vi "Diagnostics.Main.CmdResp.Engine.vi"(8 "error in (no error)":errorcluster, 11 "State Variables":T1={"Comm"=refnum, "Parameters"={"Name"="", "CAN"={"Interface"="", "Baud Rate"=0, "Diagnostic Protocol"=enum."GMLAN", "Transport Protocol"=enum."ISO TP - Normal Mode", "Transmit ID"=0, "Receive ID"=2, "Transmit Extension"=1, "Receive Extension"=255, "Receive UUDT ID"=0, "Enable Stream"=TRUE, "VW TP Channel ID"=1, "Fill Frame"=FALSE, "Fill Byte"=0, "Termination"=FALSE, "LIN Cluster"="", "NAD"=8, "IO Mode"=0, "Max DLC"=0, "FD Baud Rate"=2, "Timeout"=1, "FD ISO Mode"=0}, "986x"={"Enable"=FALSE, "RIO Device"="", "Bitfile"=path ""}, "Reads"=[], "Frames Lookup"=variant(enum16{"GMLAN", "KWP-2000", "UDS"} enum."GMLAN"), "Writes"=[], "DPIDs"=[], "DPID Lookup"=variant(u32 0), "DTC"={"Descriptor"={"DTC Byte Length"=1, "Status Byte Length"=1, "Add Data Byte Length"=1, "Byte Order"=enum."Motorola"}, "Value.Code"=[], "Value.String"=[], "Value.J2012String"=[], "Status.Code"=[], "Status.String"=[]}, "Created DTCs"=0, "Polls"=[], "Service Channels Status Lookup"=variant, "Trigger Lookup"=variant, "Security"={"Type"=enum."None", "Source DLL Path"=path "", "Target DLL Path"=path "", "Security Level"=0}}, "ADCS Connection"={"Diag CAN Handle"=0, "Transport Protocol"=enum."ISO TP - Normal Mode", "Receive Address Extension"=0, "Transmit Address Extension"=0, "Receive CAN Id"=0, "Transmit CAN Id"=0, "Log Frames ?"=FALSE, "My TP Address"=0, "Other TP Address"=0, "T1"=0, "T2"=0, "T3"=0, "T4"=0, "Tx SN"=0, "Block Size"=0, "Rx SN"=0, "VW TP Initialized?"=FALSE, "Tx block no"=0, "baud rate"=0, "Interface"="", "Channel Diag CAN Handle"=0, "UDP Connection ID"=refnum, "TCP Connection ID"=refnum, "Target IP Addr"=0, "Source Address"=0, "Target Address"=0, "Send Header NACK?"=FALSE, "DLL Handle"=0, "NAD"=0, "Time Stamp read first"=0.0, "Time Stamp read last"=0.0, "Time Stamp write first"=0.0, "Time Stamp write last"=0.0, "Time Stamp write"=0.0, "Time Stamp read"=0.0, " I/O Mode"=0, "FD Baudrate"=0, "TX_DL"=8, "RX_DL"=8, "DoIP Protocol Version"=1, " Selected I/O Mode"=0, "TesterPresent Counter"=0, "TesterPresent Limit"=0, "TesterPresent Tick[ms]"=10, "TesterPresent RequireResponse?"=FALSE, "TesterPresent Stored Ref?"=FALSE, "TesterPresent Message"=[], "TesterPresent Task Handle"=0, "TesterPresent Semaphore"=refnum, "Response Plausibility Check"=1, "Default Version?"=TRUE, "Diagostic Globals"={"Timeout FC (Bs)"=250, "Timeout CF (Cr)"=250, "Timeout Diag Command"=1000, "Receive Block Size (BS)"=0, "Wait Time CF (STmin)"=5, "Max Waits (N_WFTmax)"=10, "Waits to Send (N_WAIT)"=0, "Time between Waits (TW)"=25, "Fill CAN Frames?"=TRUE, "Fill Byte"=255, "Invalid Response as Error?"=FALSE, "Max RspPending Count"=5, "VWTP Command Timeout"=50, "Transport Protocol"=enum."Diagnostics on IP", "Diag CAN Handle"=0, "DLL Handle"=0, "Timeout RspPending"=1000}, "Session-based Properties?"=FALSE}, "XNET References"={"Database"="", "GMLAN.DPID.Frame"="", "Cluster.Convert"=""}, "XNETEngine (GMLAN)"=refnum, "Process"=refnum, "Reads"=refnum, "Writes"=refnum, "Cmds"=refnum, "DTCs"=refnum, "DTC Count"=refnum, "Status"=refnum, "Triggers"=refnum, "CANConnected"=refnum, "LocalStop"=refnum, "LocalCommStatus"=refnum, "Service Channels Status"=refnum, "Settings"=refnum, "Streaming Refs"={"Addon"="", "Port"="", "Filter Ref"=refnum, "Default Filter"={"ID Filters"=[], "Direction Filter"=enum."Tx/Rx", "Type Filter"=enum."All"}, "Port Settings"={"Mode"=0, "Baud Rate"=0, "Termination"=0, "FD ISO Mode"=0, "FD Baud Rate"=0}}} {"Streaming Refs"."Port Settings"."FD ISO Mode" items=["ISO", "Non ISO", "ISO Legacy"]; "Streaming Refs"."Port Settings"."Termination" items=["Off", "On"]; "Streaming Refs"."Port Settings"."Mode" items=["CAN 2.0", "CAN FD", "CAN FD+BRS"]; "ADCS Connection"."Diagostic Globals"."Fill Byte" format="%x"; "ADCS Connection"."TesterPresent Message" format="%.0x"; "ADCS Connection"."Selected I/O Mode" items=["CAN", "CAN FD", "CAN FD+BRS", "ECU Determined"]; "ADCS Connection"."DoIP Protocol Version" items=["2010"=1, "2012"=2]; "ADCS Connection"."RX_DL" items=["8"=8, "12"=12, "16"=16, "20"=20, "24"=24, "32"=32, "48"=48, "64"=64]; "ADCS Connection"."TX_DL" items=["8"=8, "12"=12, "16"=16, "20"=20, "24"=24, "32"=32, "48"=48, "64"=64]; "ADCS Connection"."I/O Mode" items=["CAN", "CAN FD", "CAN FD+BRS", "Not yet determined"]; "Parameters"."Writes"."Signals"."Byte Order" items=["Little Endian", "Big Endian"]; "Parameters"."Writes"."Signals"."Data Type" items=["Signed", "Unsigned", "IEEE Float"]; "Parameters"."CAN"."FD ISO Mode" items=["ISO", "Non ISO", "ISO Legacy"]; "Parameters"."CAN"."IO Mode" items=["CAN 2.0", "CAN FD", "CAN FD+BRS"]; "Parameters"."CAN"."Fill Byte" format="%.0x"; "Parameters"."CAN"."VW TP Channel ID" format="%.0x"; "Parameters"."CAN"."Receive UUDT ID" format="%.0x"; "Parameters"."CAN"."Receive Extension" format="%.0x"; "Parameters"."CAN"."Transmit Extension" format="%.0x"; "Parameters"."CAN"."Receive ID" format="%.0x"; "Parameters"."CAN"."Transmit ID" format="%.0x"; "Parameters"."Reads"."Signals"."Byte Order" items=["Little Endian", "Big Endian"]; "Parameters"."Reads"."Signals"."Data Type" items=["Signed", "Unsigned", "IEEE Float"]}) -> (0 "error out":errorcluster)   [LabVIEW 2019, in "Diagnostics Addon Engine.lvlib"]
doc: "Async loop that handles the UDS commands sent either by the channel engine or the TCP engine"
uses:
  Diagnostics Addon Engine.lvlib
  Types/Diagnostics.State.ctl
  <vilib>/NI/NIVS Inline Async API/_VS Inline Async API/Process/Process.lvclass
  <vilib>/NI/NI VeriStand Addon Network Comm/Engine/VeriStand Comm.lvclass
  Addon Shared/Types/SysDef.Compile.ctl
  Addon Shared/Types/CAN.ctl
  Addon Shared/Types/CAN.Interface.ctl
  Addon Shared/Types/Protocol.ctl
  Addon Shared/Types/Transport.ctl
  Addon Shared/Types/986x.ctl
  Addon Shared/Types/Frame.Compile.ctl
  Addon Shared/Types/Type.ctl
  Addon Shared/Types/Signal.ctl
  Addon Shared/Types/DPID.ctl
  Addon Shared/Types/DPID.Rate.ctl
  Addon Shared/Types/DTC.Settings.ctl
  Addon Shared/Types/DTC.Descriptor.ctl
  Addon Shared/Types/Poll.Compiled.ctl
  Addon Shared/Types/Security.ctl
  Addon Shared/Types/Security.Type.ctl
  <vilib>/Automotive Diagnostic Command Set/Diagnostic Transport.llb/Diag Reference.ctl
  <vilib>/Automotive Diagnostic Command Set/Diagnostic Transport.llb/Transport Protocol Selector.ctl
  <vilib>/Automotive Diagnostic Command Set/Diagnostic Transport.llb/DoIP Protocol Version.ctl
  <vilib>/Automotive Diagnostic Command Set/Diagnostic Transport.llb/Diag Globals.ctl
  Types/XNET.Refs.ctl
  <vilib>/NI/AMC/Message Queue.ctl
  <vilib>/NI/AMC/Message.ctl
  <vilib>/NI/Tools/Keyed Array/KeyedArray.ctl
  <vilib>/NI/NIVS Inline Async API/_Data Access Engine/Data Access Engine/Types/Write.DVR.ctl
  <vilib>/NI/NIVS Inline Async API/_Data Access Engine/Access Type Classes/Write/Write.lvclass
  <vilib>/NI/NIVS Inline Async API/_Data Access Engine/Data Access Engine/Types/Read.DVR.ctl
  <vilib>/NI/NIVS Inline Async API/_Data Access Engine/Access Type Classes/Read/Read.lvclass
  <vilib>/NI/NIVS Inline Async API/_Data Access Engine/Data Access Engine/Types/ReadWrite.DVR.ctl
  <vilib>/NI/NIVS Inline Async API/_Data Access Engine/Access Type Classes/ReadWrite/ReadWrite.lvclass
  SubModules/CAN-Streaming-Support/Source/Addon/Addon Engine/Types/Engine Stream Refs.ctl
  SubModules/CAN-Streaming-Support/Source/Addon/Addon Shared/Types/Direction Filter.ctl
  SubModules/CAN-Streaming-Support/Source/Addon/Addon Shared/Types/Type Filter.ctl
  SubModules/CAN-Streaming-Support/Source/Addon/Addon Shared/Types/Filter Parameters.ctl
  SubModules/CAN-Streaming-Support/Source/Addon/Addon Engine/Types/Engine Stream Port Settings.ctl
  Types/Polling.States.ctl
  Addon Shared/Types/DTC.Info.ctl
  <vilib>/NI/NI VeriStand Addon Network Comm/Engine/VeriStand Comm.lvclass/VeriStand Comm.ctl
  <vilib>/NI/NIVS Inline Async API/_Data Access Engine/Access Type Classes/Write/Write.lvclass/Write.ctl
  <vilib>/Automotive Diagnostic Command Set/Diagnostic Transport.llb/Property ID.ctl
  Support Libraries/GMLAN/_Types/ReadFailureRecordData_readFailureRecordParameters_failureRecordIdentifier.ctl
  Addon Shared/Types/Command.ReadDTCbyDTCNumber.ctl
  Support Libraries/GMLAN/_Types/ReadDataByPacketIdentifier_SubFunctions.ctl
  <vilib>/NI/NIVS Inline Async API/_Data Access Engine/Access Type Classes/Read/Read.lvclass/Read.ctl
  Support Libraries/GMLAN/_Types/TesterPresent_Parameter.ctl
  Support Libraries/GMLAN/_Types/InitiateDiagnosticOperation_Parameter.ctl
  Support Libraries/GMLAN/_Types/InitiateDiagnosticOperation_SubFunctions.ctl
  Addon Shared/Types/Command.Communication.ctl
  Support Libraries/GMLAN/_Types/DisableNormalCommunication_Parameter.ctl
  Addon Shared/Types/Command.ReadDTC.ctl
  Addon Shared/Types/DTC.Descriptor.Override.ctl
  Addon Shared/Types/Command.ClearDTC.ctl
  Addon Shared/Types/Frame.Data.ctl
  Addon Shared/Types/Command.PassThru.Channel.ctl
  Addon Shared/Types/Command.ControlDTC.ctl
  Addon Shared/Types/Command.Memory.ctl
  Addon Shared/Types/Command.IO.ctl
  <vilib>/NI/NIVS Inline Async API/_VS Inline Async API/Process/Process.lvclass/Process.ctl
  <vilib>/NI/NIVS Inline Async API/_Data Access Engine/Data Access Engine/Methods/Write.Data.Commit.vi
  <vilib>/NI/NIVS Inline Async API/_Data Access Engine/Data Access Engine/Methods/Write.Data.vi
  <vilib>/NI/NIVS Inline Async API/_Data Access Engine/Data Access Engine/Methods/Write.Data.Buffer.vi
  Addon Shared/SubVIs/LookupID.Create.vi
  <vilib>/NI/AMC/Send Local Messages.vi
  <vilib>/Utility/error.llb/Clear Errors.vi
  <vilib>/NI/NIVS Inline Async API/_Data Access Engine/Access Type Classes/Write/Write.Commit.vi
  <vilib>/NI/NIVS Inline Async API/_Data Access Engine/Data Access Engine/Methods/Read.Data.vi
  Support Libraries/GMLAN/Utilities/GMLAN Service Broadcast.vi
  Support Libraries/GMLAN/GMLAN SecurityAccess.vi
  Support Libraries/GMLAN/_SubVIs/SecurityAccess_sendKey.vi
  Security.DLL.vi
  Support Libraries/GMLAN/_SubVIs/SecurityAccess_requestSeed.vi
  <vilib>/NI/NIVS Inline Async API/_Data Access Engine/Access Type Classes/Write/Write.ProcessData.vi
  <vilib>/NI/AMC/Create Single Message.vi
  <vilib>/NI/AMC/Update Message Routing Info.vi
  <vilib>/NI/NIVS Inline Async API/_VS Inline Async API/Error Handling Process/SubVIs/Error.ConvertArray.vi
  <vilib>/NI/AMC/Read Next Message.vi
  <vilib>/NI/Tools/Keyed Array/Index.vi
  <vilib>/NI/NIVS Inline Async API/_Data Access Engine/Access Type Classes/Write/Write.Buffer.vi
  <vilib>/NI/AMC/Create Multiple Messages.vi
  <vilib>/NI/NIVS Inline Async API/_Data Access Engine/Access Type Classes/Read/Read.ProcessData.vi
  <vilib>/Automotive Diagnostic Command Set/Diagnostic Transport.llb/Diagnostic Service Send.vi
  <vilib>/Automotive Diagnostic Command Set/Diagnostic Transport.llb/Diagnostic Response Recv.vi
  <vilib>/NI/AMC/Read Termination Message.vi
  <vilib>/NI/Tools/Keyed Array/Map String.vi
  <vilib>/Automotive Diagnostic Command Set/Diagnostic Transport.llb/ISOTP Transmit.vi
  <vilib>/Automotive Diagnostic Command Set/Diagnostic Transport.llb/ISOTP7 Transmit.vi
  <vilib>/Automotive Diagnostic Command Set/Diagnostic Transport.llb/DoIP Transmit.vi
  <vilib>/Automotive Diagnostic Command Set/Diagnostic Transport.llb/LIN ISOTP Transmit.vi
  <vilib>/Automotive Diagnostic Command Set/Diagnostic Transport.llb/Diagnostic Service Recv.vi
  <vilib>/NI/Tools/String/Get Case Matching.vi
  <vilib>/Automotive Diagnostic Command Set/Diagnostic Transport.llb/ISOTP Send FF.vi
  <vilib>/Automotive Diagnostic Command Set/Diagnostic Transport.llb/ISOTP Send CFs.vi
  <vilib>/Automotive Diagnostic Command Set/Diagnostic Transport.llb/ISOTP Send Frame.vi
  <vilib>/Automotive Diagnostic Command Set/Diagnostic Transport.llb/ISOTP7 Send FF.vi
  <vilib>/Automotive Diagnostic Command Set/Diagnostic Transport.llb/ISOTP7 Send CFs.vi
  <vilib>/Automotive Diagnostic Command Set/Diagnostic Transport.llb/ISOTP7 Send Frame.vi
  <vilib>/Automotive Diagnostic Command Set/Diagnostic Transport.llb/DoIP TCP Msg Send.vi
  <vilib>/Automotive Diagnostic Command Set/Diagnostic Transport.llb/DoIP TCP Msg Recv.vi
  <vilib>/Automotive Diagnostic Command Set/Diagnostic Transport.llb/DoIP Check Addresses.vi
  <vilib>/Automotive Diagnostic Command Set/Diagnostic Transport.llb/DoIP Check ACK Code.vi
  <vilib>/Automotive Diagnostic Command Set/Diagnostic Transport.llb/ISOTP Receive.vi
  <vilib>/Automotive Diagnostic Command Set/Diagnostic Transport.llb/ISOTP7 Receive.vi
  <vilib>/Automotive Diagnostic Command Set/Diagnostic Transport.llb/DoIP Receive.vi
  <vilib>/Automotive Diagnostic Command Set/Diagnostic Transport.llb/LIN ISOTP Receive.vi
  <vilib>/Automotive Diagnostic Command Set/Diagnostic Transport.llb/Diag Get Globals.vi
  <vilib>/Automotive Diagnostic Command Set/Diagnostic Transport.llb/ISOTP Recv FC.vi
  <vilib>/Automotive Diagnostic Command Set/Diagnostic Transport.llb/ISOTP Send CF.vi
  <vilib>/Automotive Diagnostic Command Set/Diagnostic Transport.llb/Diag Fill Frame.vi
  <vilib>/Automotive Diagnostic Command Set/Diagnostic Transport.llb/ISOTP Calc Send Params.vi
  <vilib>/Automotive Diagnostic Command Set/Diagnostic Transport.llb/ISOTP7 Recv FC.vi
  <vilib>/Automotive Diagnostic Command Set/Diagnostic Transport.llb/ISOTP7 Send CF.vi
  <vilib>/Automotive Diagnostic Command Set/Diagnostic Transport.llb/DoIP Add Addresses.vi
  <vilib>/Automotive Diagnostic Command Set/Diagnostic Transport.llb/DoIP TCP Send.vi
  <vilib>/Automotive Diagnostic Command Set/Diagnostic Transport.llb/DoIP TCP Recv.vi
  <vilib>/Automotive Diagnostic Command Set/Diagnostic Transport.llb/DoIP Add Header.vi
  <vilib>/Automotive Diagnostic Command Set/Diagnostic Transport.llb/ISOTP Recv Frame.vi
  <vilib>/Automotive Diagnostic Command Set/Diagnostic Transport.llb/ISOTP Recv CFs.vi
  <vilib>/Automotive Diagnostic Command Set/Diagnostic Transport.llb/ISOTP7 Recv Frame.vi
  <vilib>/Automotive Diagnostic Command Set/Diagnostic Transport.llb/ISOTP7 Recv CFs.vi
  <vilib>/Automotive Diagnostic Command Set/Diagnostic Transport.llb/DoIP Send Alive.vi
  <vilib>/Automotive Diagnostic Command Set/Diagnostic Transport.llb/DoIP Check Error.vi
  <vilib>/Automotive Diagnostic Command Set/Diagnostic Transport.llb/ISOTP Check Redo.vi
  <vilib>/Automotive Diagnostic Command Set/Diagnostic Transport.llb/ISOTP Recv Block.vi
  <vilib>/Automotive Diagnostic Command Set/Diagnostic Transport.llb/ISOTP7 Recv Block.vi
  <vilib>/Automotive Diagnostic Command Set/Diagnostic Transport.llb/ISOTP Send FC.vi
  <vilib>/Automotive Diagnostic Command Set/Diagnostic Transport.llb/ISOTP Add CF.vi
  <vilib>/Automotive Diagnostic Command Set/Diagnostic Transport.llb/ISOTP7 Send FC.vi
  <vilib>/Automotive Diagnostic Command Set/Diagnostic Transport.llb/ISOTP7 Add CF.vi
  <vilib>/NI/NI VeriStand Addon Network Comm/Shared/Comm Constants.vi
  <vilib>/NI/AMC/Globals.vi
  <vilib>/NI/AMC/Send Message.vi
  <vilib>/Automotive Diagnostic Command Set/Diagnostic Transport.llb/Apply Success Failure Error.vi
  Addon Shared/SubVIs/Constants.vi
  <vilib>/xnet/xnet.llb/XNET Convert.vi
  <vilib>/xnet/xnet.llb/XNET Convert (Frame CAN to Signal).vi
  <vilib>/xnet/xnet.llb/XNET Convert (Signal to Frame CAN).vi
  <vilib>/Automotive Diagnostic Command Set/Diagnostic Transport.llb/Diag Globals.vi
  <vilib>/Automotive Diagnostic Command Set/Diagnostic Transport.llb/CAN Send Frame Check Queue.vi
  <vilib>/Automotive Diagnostic Command Set/Diagnostic Transport.llb/Diag CAN get timestamp.vi
  <vilib>/Automotive Diagnostic Command Set/Diagnostic Transport.llb/Diag CAN read.vi
  <vilib>/Automotive Diagnostic Command Set/Diagnostic Transport.llb/ISOTP Calc Actual IO Mode.vi
  <vilib>/Automotive Diagnostic Command Set/Diagnostic Transport.llb/ISOTP Get FC Data.vi
  <vilib>/Automotive Diagnostic Command Set/Diagnostic Transport.llb/VWTP Write.vi
  <vilib>/Automotive Diagnostic Command Set/Diagnostic Transport.llb/DoIP Analyze Header.vi
  <vilib>/Automotive Diagnostic Command Set/Diagnostic Transport.llb/Diag CAN status.vi
  <vilib>/Automotive Diagnostic Command Set/Diagnostic Transport.llb/VWTP Read.vi
  <vilib>/Automotive Diagnostic Command Set/Diagnostic Transport.llb/Apply Diagnostic Error.vi
  <vilib>/Automotive Diagnostic Command Set/Diagnostic Protocols.llb/UDS RequestSeed.vi
  <vilib>/Automotive Diagnostic Command Set/Diagnostic Protocols.llb/RequestSeed.vi
  <vilib>/Automotive Diagnostic Command Set/Diagnostic Protocols.llb/UDS SendKey.vi
  <vilib>/Automotive Diagnostic Command Set/Diagnostic Protocols.llb/SendKey.vi
  Addon Shared/Diagnostics Addon Shared.lvlib
  <vilib>/NI/AMC/AMC.lvlib
  Support Libraries/GMLAN/GMLAN.lvlib
  <vilib>/addons/Automotive Diagnostic Command Set/NI_Automotive Diagnostic Command Set.lvlib
  <vilib>/NI/NIVS Inline Async API/_Data Access Engine/Data Access Engine/Data Access Engine.lvclass
  <vilib>/Utility/SystemLogging/NI_SystemLogging.lvlib
  SubModules/CAN-Streaming-Support/Source/Addon/Addon Engine/CAN Stream Support Engine.lvlib
  SubModules/CAN-Streaming-Support/Source/Addon/Addon Shared/CAN Stream Support Shared.lvlib
  <vilib>/NI/Tools/Keyed Array/Tools_KeyedArray.lvlib
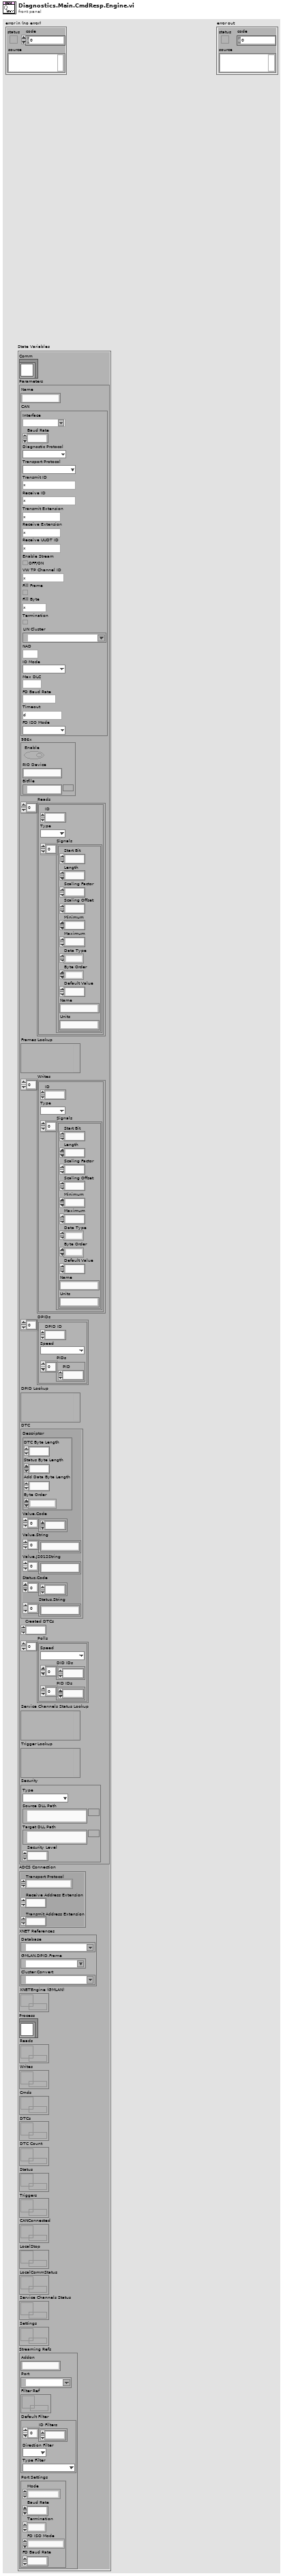
[diagram p1: front panel]
types:
  T1 = typedef "Diagnostics Addon Engine.lvlib/Diagnostics.State.ctl" = cluster{"Comm":refnum<class "VeriStand Comm.lvclass">, "Parameters":T2, "ADCS Connection":T18, "XNET References":T23, "XNETEngine (GMLAN)":T24, "Process":refnum<class "Process.lvclass">, "Reads":T25, "Writes":T26, "Cmds":T27, "DTCs":T25, "DTC Count":T25, "Status":T25, "Triggers":T27, "CANConnected":T25, "LocalStop":refnum<data-value>, "LocalCommStatus":refnum<data-value>, "Service Channels Status":T25, "Settings":T26, "Streaming Refs":T28}
  T2 = typedef "Diagnostics Addon Shared.lvlib/SysDef.Compile.ctl" = cluster{"Name":string, "CAN":T3, "986x":T7, "Reads":T8[], "Frames Lookup":variant, "Writes":T8[], "DPIDs":T11[], "DPID Lookup":variant, "DTC":T13, "Created DTCs":u32, "Polls":T15[], "Service Channels Status Lookup":variant, "Trigger Lookup":variant, "Security":T16}
  T3 = typedef "Diagnostics Addon Shared.lvlib/CAN.ctl" = cluster{"Interface":T4, "Baud Rate":u64, "Diagnostic Protocol":T5, "Transport Protocol":T6, "Transmit ID":u32, "Receive ID":u32, "Transmit Extension":u8, "Receive Extension":u8, "Receive UUDT ID":u32, "Enable Stream":bool, "VW TP Channel ID":u32, "Fill Frame":bool, "Fill Byte":u8, "Termination":bool, "LIN Cluster":refnum<k21>, "NAD":u8, "IO Mode":u32, "Max DLC":u16, "FD Baud Rate":u64, "Timeout":u32, "FD ISO Mode":u32}
  T4 = typedef "Diagnostics Addon Shared.lvlib/CAN.Interface.ctl" = string
  T5 = typedef "Diagnostics Addon Shared.lvlib/Protocol.ctl" = enum16{"GMLAN", "KWP-2000", "UDS", "User-Defined"}
  T6 = typedef "Diagnostics Addon Shared.lvlib/Transport.ctl" = enum16{"ISO TP - Normal Mode", "ISO TP - Mixed Mode", "VW TP 2.0", "Diagnostics on IP", "ISO TP LIN"}
  T7 = typedef "Diagnostics Addon Shared.lvlib/986x.ctl" = cluster{"Enable":bool, "RIO Device":string, "Bitfile":path}
  T8 = typedef "Diagnostics Addon Shared.lvlib/Frame.Compile.ctl" = cluster{"ID":u32, "Type":T9, "Signals":T10[]}
  T9 = typedef "Diagnostics Addon Shared.lvlib/Type.ctl" = enum16{"DID", "CDID", "PID", "CPID", "Read Memory", "Write Memory", "IO Control", "Routine Start", "Routine Request", "Routine Stop", "User Defined", "DTC Control", "Clear DTCs", "Read DTCs", "Start DTCs", "DTC Change Count", "Tester Present", "Unlock ECU", "Reset ECU", "Diag Session Control", "Communication Control", "DPID Control", "Poll Control", "Diag CAN Control"}
  T10 = typedef "Diagnostics Addon Shared.lvlib/Signal.ctl" = cluster{"Start Bit":u32, "Length":u32, "Scaling Factor":dbl, "Scaling Offset":dbl, "Minimum":dbl, "Maximum":dbl, "Data Type":u32, "Byte Order":u32, "Default Value":dbl, "Name":string, "Units":string}
  T11 = typedef "Diagnostics Addon Shared.lvlib/DPID.ctl" = cluster{"DPID ID":u8, "Speed":T12, "PIDs":u16[]}
  T12 = typedef "Diagnostics Addon Shared.lvlib/DPID.Rate.ctl" = enum16{"Slow", "Medium", "Fast"}
  T13 = typedef "Diagnostics Addon Shared.lvlib/DTC.Settings.ctl" = cluster{"Descriptor":T14, "Value.Code":dbl[], "Value.String":string[], "Value.J2012String":string[], "Status.Code":dbl[], "Status.String":string[]}
  T14 = typedef "Diagnostics Addon Shared.lvlib/DTC.Descriptor.ctl" = cluster{"DTC Byte Length":i32, "Status Byte Length":i32, "Add Data Byte Length":i32, "Byte Order":enum16{"Motorola", "Intel"}}
  T15 = typedef "Diagnostics Addon Shared.lvlib/Poll.Compiled.ctl" = cluster{"Speed":T12, "DID IDs":u32[], "PID IDs":u32[]}
  T16 = typedef "Diagnostics Addon Shared.lvlib/Security.ctl" = cluster{"Type":T17, "Source DLL Path":path, "Target DLL Path":path, "Security Level":u8}
  T17 = typedef "Diagnostics Addon Shared.lvlib/Security.Type.ctl" = enum16{"None", "SeedKey", "MasterKey"}
  T18 = typedef "NI_Automotive Diagnostic Command Set.lvlib/Diag Reference.ctl" = cluster{"Diag CAN Handle":u32, "Transport Protocol":T19, "Receive Address Extension":u8, "Transmit Address Extension":u8, "Receive CAN Id":u32, "Transmit CAN Id":u32, "Log Frames ?":bool, "My TP Address":u8, "Other TP Address":u8, "T1":u16, "T2":u16, "T3":u16, "T4":u16, "Tx SN":u8, "Block Size":u8, "Rx SN":u8, "VW TP Initialized?":bool, "Tx block no":u8, "baud rate":u64, "Interface":string, "Channel Diag CAN Handle":u32, "UDP Connection ID":refnum<k16>, "TCP Connection ID":refnum<k5>, "Target IP Addr":u32, "Source Address":u16, "Target Address":u16, "Send Header NACK?":bool, "DLL Handle":u32, "NAD":u8, "Time Stamp read first":dbl, "Time Stamp read last":dbl, "Time Stamp write first":dbl, "Time Stamp write last":dbl, "Time Stamp write":dbl, "Time Stamp read":dbl, " I/O Mode":u32, "FD Baudrate":u64, "TX_DL":u16, "RX_DL":u16, "DoIP Protocol Version":T20, " Selected I/O Mode":u32, "TesterPresent Counter":u32, "TesterPresent Limit":u32, "TesterPresent Tick[ms]":i32, "TesterPresent RequireResponse?":bool, "TesterPresent Stored Ref?":bool, "TesterPresent Message":u8[], "TesterPresent Task Handle":i32, "TesterPresent Semaphore":T21, "Response Plausibility Check":u32, "Default Version?":bool, "Diagostic Globals":T22, "Session-based Properties?":bool}
  T19 = typedef "NI_Automotive Diagnostic Command Set.lvlib/Transport Protocol Selector.ctl" = enum16{"ISO TP - Normal Mode", "ISO TP - Mixed Mode", "VW TP 2.0", "Diagnostics on IP", "ISO TP LIN"}
  T20 = typedef "NI_Automotive Diagnostic Command Set.lvlib/DoIP Protocol Version.ctl" = u8
  T21 = typedef "Semaphore RefNum" = refnum<k1>
  T22 = typedef "NI_Automotive Diagnostic Command Set.lvlib/Diag Globals.ctl" = cluster{"Timeout FC (Bs)":u32, "Timeout CF (Cr)":u32, "Timeout Diag Command":u32, "Receive Block Size (BS)":u8, "Wait Time CF (STmin)":u8, "Max Waits (N_WFTmax)":u8, "Waits to Send (N_WAIT)":i32, "Time between Waits (TW)":u32, "Fill CAN Frames?":bool, "Fill Byte":u32, "Invalid Response as Error?":bool, "Max RspPending Count":u32, "VWTP Command Timeout":u32, "Transport Protocol":T19, "Diag CAN Handle":u32, "DLL Handle":u32, "Timeout RspPending":u32}
  T23 = typedef "Diagnostics Addon Engine.lvlib/XNET.Refs.ctl" = cluster{"Database":refnum<k21>, "GMLAN.DPID.Frame":refnum<k21>, "Cluster.Convert":refnum<k21>}
  T24 = typedef "AMC.lvlib/Message Queue.ctl" = refnum<queue>
  T25 = typedef "Data Access Engine.lvlib/Data Access Engine.lvclass/Write.DVR.ctl" = refnum<data-value>
  T26 = typedef "Data Access Engine.lvlib/Data Access Engine.lvclass/Read.DVR.ctl" = refnum<data-value>
  T27 = typedef "Data Access Engine.lvlib/Data Access Engine.lvclass/ReadWrite.DVR.ctl" = refnum<data-value>
  T28 = typedef "CAN Stream Support Engine.lvlib/Engine Stream Refs.ctl" = cluster{"Addon":string, "Port":refnum<k21>, "Filter Ref":refnum<data-value>, "Default Filter":T29, "Port Settings":T32}
  T29 = typedef "CAN Stream Support Shared.lvlib/Filter Parameters.ctl" = cluster{"ID Filters":u32[], "Direction Filter":T30, "Type Filter":T31}
  T30 = typedef "CAN Stream Support Shared.lvlib/Direction Filter.ctl" = enum16{"Tx/Rx", "Rx", "Tx"}
  T31 = typedef "CAN Stream Support Shared.lvlib/Type Filter.ctl" = enum16{"All", "CAN Data", "CAN Remote", "CAN Bus Error", "CAN 2.0 Data", "CAN FD Data", "CAN FD+BRS Data", "J1939 Data", "Delay", "Log Trigger", "Start Trigger"}
  T32 = typedef "CAN Stream Support Engine.lvlib/Engine Stream Port Settings.ctl" = cluster{"Mode":u32, "Baud Rate":u64, "Termination":u32, "FD ISO Mode":u32, "FD Baud Rate":u64}
  T33 = typedef "Diagnostics Addon Engine.lvlib/Polling.States.ctl" = cluster{"Enabled":bool[], "Last Generation":u32[], "Queued":bool[]}
  T34 = typedef "Diagnostics Addon Shared.lvlib/DTC.Info.ctl" = cluster{"Timestamp":dbl, "DTC":dbl, "Status":dbl, "Add Data":dbl}
  T35 = cluster{"Active DTCs":T34[], "status mask":u8, "PID IDs":u32[], "DID IDs":u32[], "Memory IDs":u32[], "TesterPresentEnabled?":bool, "Polling":T33}
  T36 = typedef "NI_Automotive Diagnostic Command Set.lvlib/Property ID.ctl" = enum16{"Timeout Diag Command", "Timeout FC (Bs)", "Timeout CF (Cr)", "Receive Block Size (BS)", "Wait Time CF (STmin)", "Max Wait Frames (N_WFTmax)", "Wait Frames to Send (N_WAIT)", "Time between Waits (T_W)", "Fill CAN Frames", "Fill Byte", "Invalid Response as Error", "Max RspPending Count", "VWTP Command Timeout", "STmin", "P2min", "Termination", "Timeout RspPending", "LIN Sleep", "Actual CAN IO Mode", "Response Plausibility Check", "Session-based Properties"}
  T37 = typedef "GMLAN.lvlib/ReadFailureRecordData_readFailureRecordParameters_failureRecordIdentifier.ctl" = cluster{"failureRecordNumber":u8, "DTC ID":u16, "DTCFailureType":u8}
  T38 = enum16{"open", "replace", "create", "open or create", "replace or create", "replace or create with confirmation"}
  T39 = typedef "Diagnostics Addon Shared.lvlib/Command.ReadDTCbyDTCNumber.ctl" = cluster{"DTC":u16, "FailTypeByte":u8}
  T40 = typedef "GMLAN.lvlib/ReadDataByPacketIdentifier_SubFunctions.ctl" = enum8{"stopSending", "sendOneResponse", "scheduleAtSlowRate", "scheduleAtMediumRate", "scheduleAtFastRate"}
  T41 = typedef "GMLAN.lvlib/TesterPresent_Parameter.ctl" = enum8{"SpecificECU", "EntireNetwork"}
  T42 = typedef "GMLAN.lvlib/InitiateDiagnosticOperation_Parameter.ctl" = enum8{"SpecificECU", "EntireNetwork"}
  T43 = typedef "Diagnostics Addon Shared.lvlib/Command.Communication.ctl" = cluster{"Type":u8, "CommType":u8}
  T44 = typedef "GMLAN.lvlib/DisableNormalCommunication_Parameter.ctl" = enum8{"SpecificECU", "EntireNetwork"}
  T45 = typedef "Diagnostics Addon Shared.lvlib/Command.ReadDTC.ctl" = cluster{"Extension":u32, "Mask":u32, "Mode/Status":u32, "Byte Lengths":T46}
  T46 = typedef "Diagnostics Addon Shared.lvlib/DTC.Descriptor.Override.ctl" = cluster{"Override":bool, "DTC":u32, "Status":u32, "Failure":u32}
  T47 = typedef "Diagnostics Addon Shared.lvlib/Command.ClearDTC.ctl" = cluster{"Group of DTC":u32, "Byte Lengths":T46}
  T48 = typedef "Diagnostics Addon Shared.lvlib/Frame.Data.ctl" = cluster{"ID":u32, "Raw Frame":u8[], "error out":errorcluster}
  T49 = typedef "Diagnostics Addon Shared.lvlib/Command.PassThru.Channel.ctl" = cluster{"Service":u64, "Service Length":u8, "Data Length":u32, "Response Required":bool}
  T50 = cluster{"resp":u8[], "error code":u8, "error out":errorcluster}
  T51 = typedef "Diagnostics Addon Shared.lvlib/Command.ControlDTC.ctl" = cluster{"Group/Type":u32, "Byte Lengths (KWP only)":T46}
  T52 = typedef "Diagnostics Addon Shared.lvlib/Command.Memory.ctl" = cluster{"Address":u64, "Service Type":u32, "Address Length":u8, "Size Length":u8}
  T53 = typedef "Diagnostics Addon Shared.lvlib/Command.IO.ctl" = cluster{"ID":u16, "Mode":u8}
  T54 = typedef "NI VeriStand Addon Network Comm.lvlib/VeriStand Comm.lvclass/Response Information.ctl" = cluster{"response name":string, "responseQ":string}
  T55 = cluster{"ID Filters":u32[], "Direction Filter":T30, "Type Filter":T31}
  T56 = cluster{"Boolean array[0]":bool, "Boolean array[1]":bool, "Boolean array[2]":bool, "Boolean array[3]":bool, "Boolean array[4]":bool, "Boolean array[5]":bool, "Boolean array[6]":bool, "Boolean array[7]":bool}
  T57 = typedef "Diagnostics Addon Engine.lvlib/DPIDs.IDs.Sorted.ctl" = cluster{"Slow":u8[], "Medium":u8[], "Fast":u8[]}
  T58 = typedef "GMLAN.lvlib/InitiateDiagnosticOperation_SubFunctions.ctl" = u8
  T59 = typedef "Diagnostic Trouble Code.ctl" = cluster{"DTC":u32, "Status":u32, "Add Data":u32}
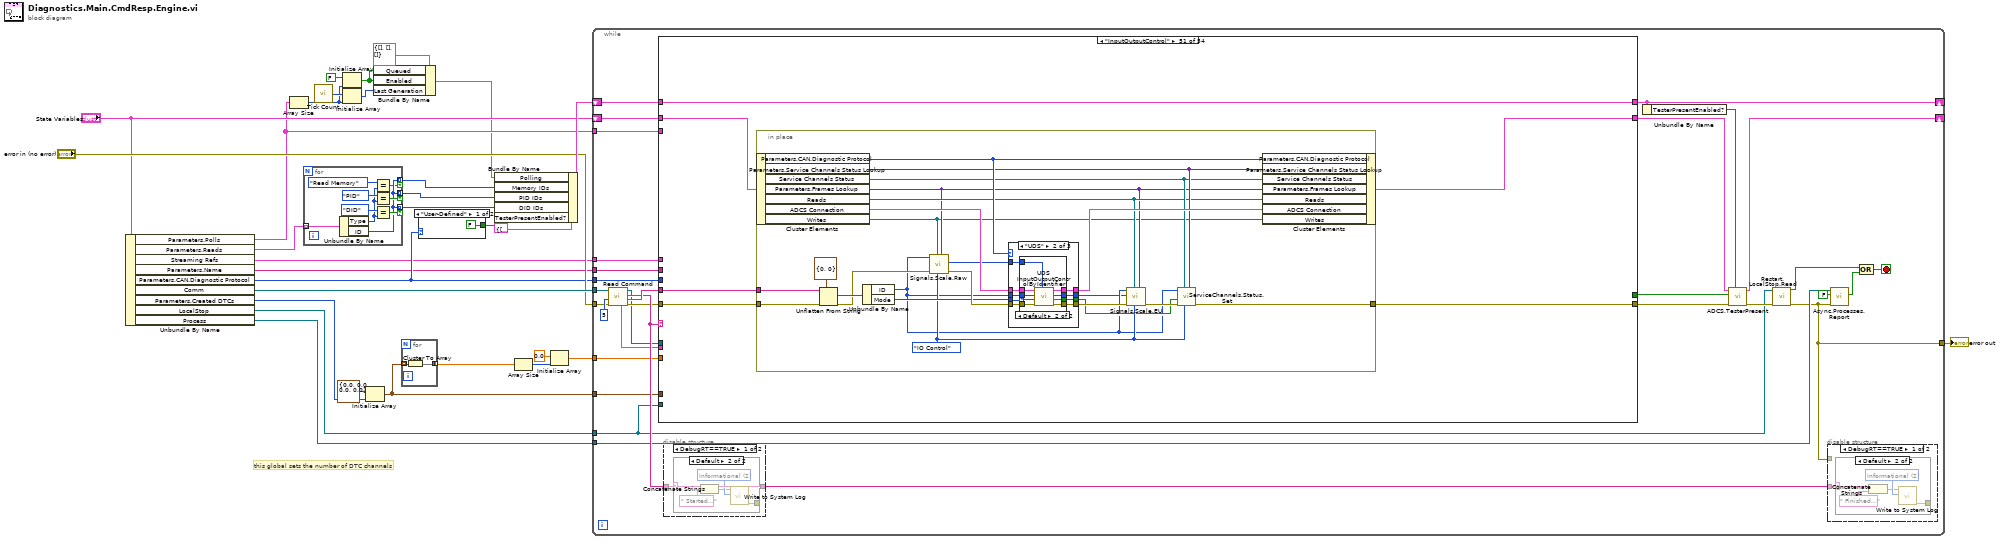
[diagram p0: block diagram]
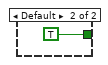
[diagram p2: hidden frame]
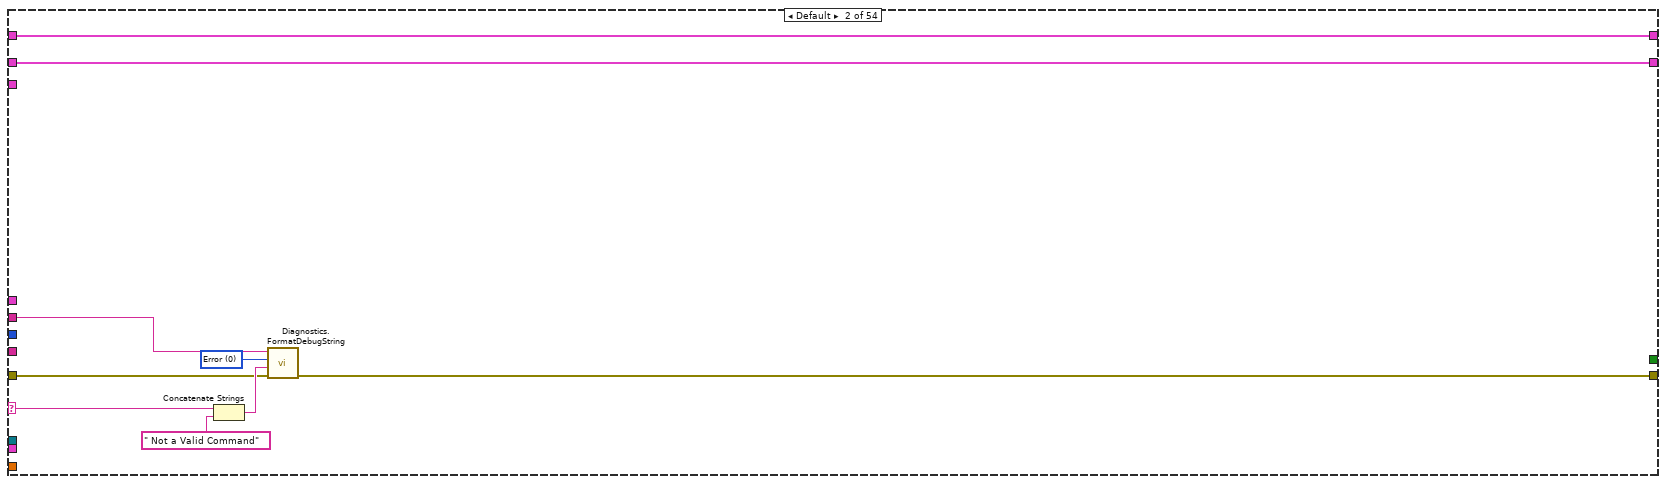
[diagram p8: hidden frame]
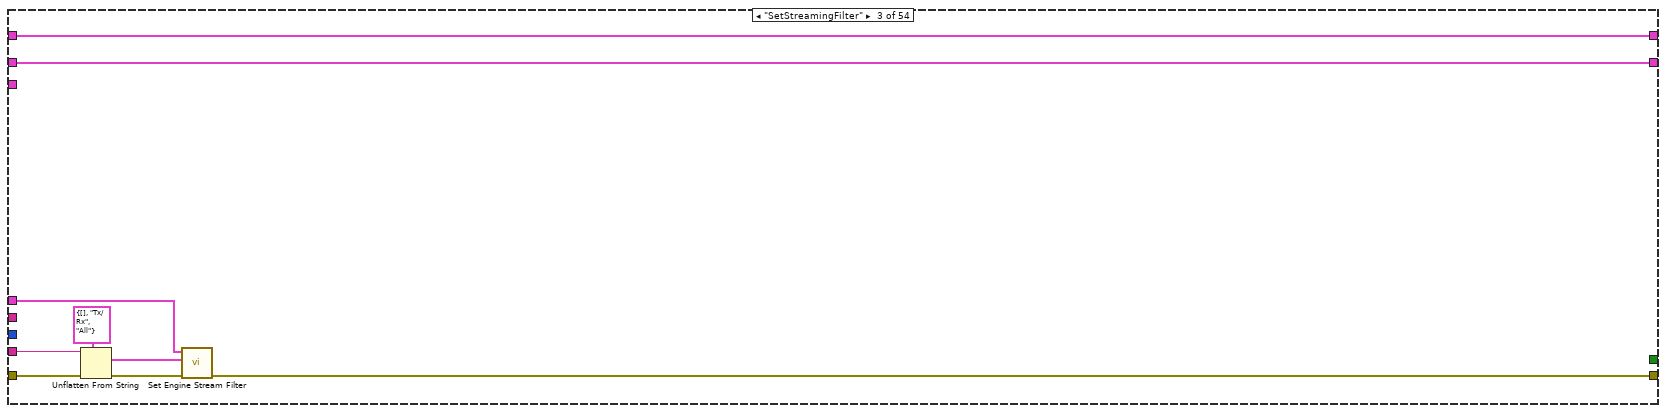
[diagram p9: hidden frame]
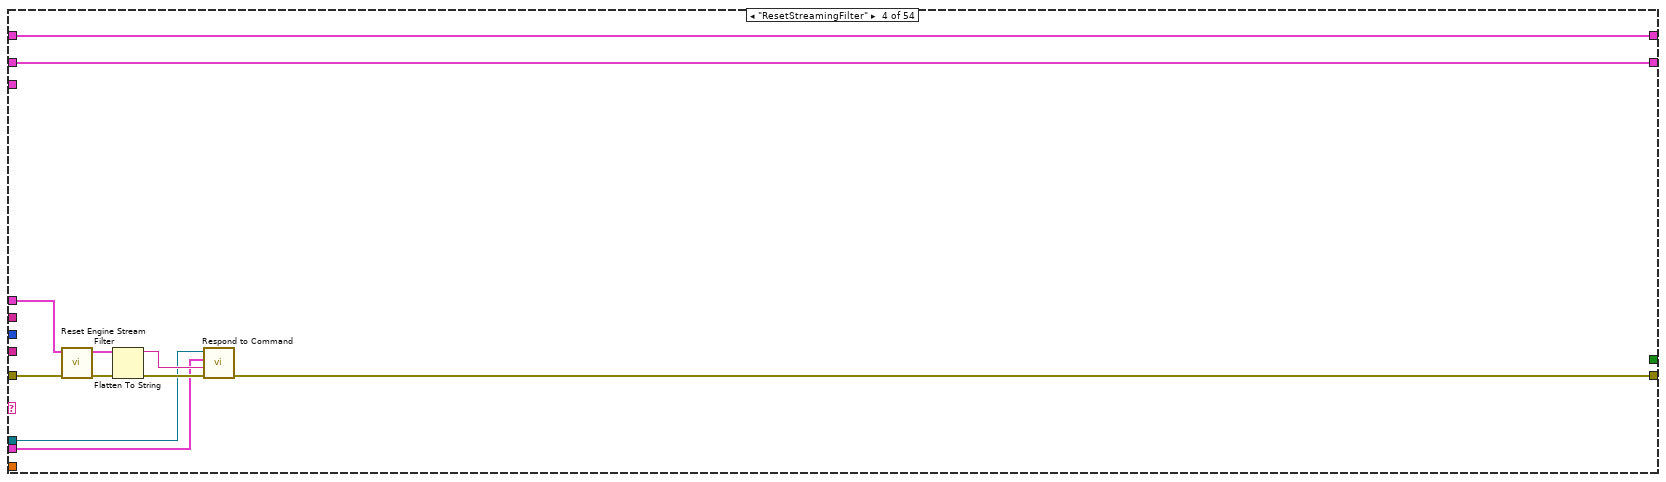
[diagram p10: hidden frame]
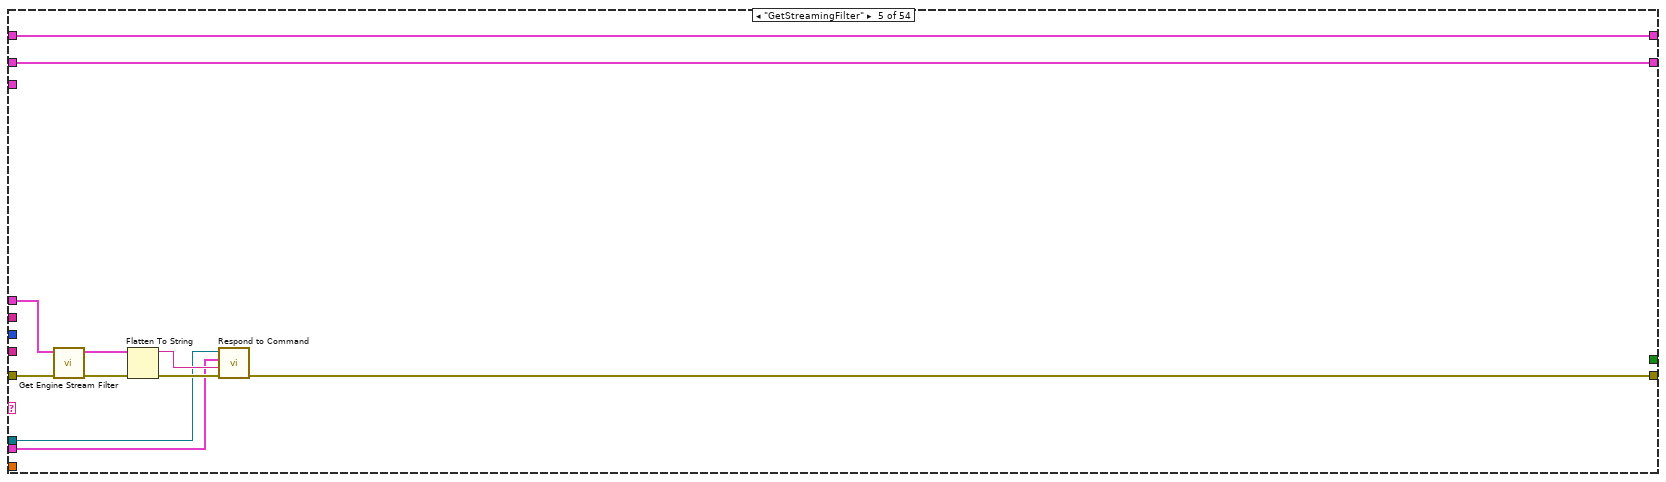
[diagram p11: hidden frame]
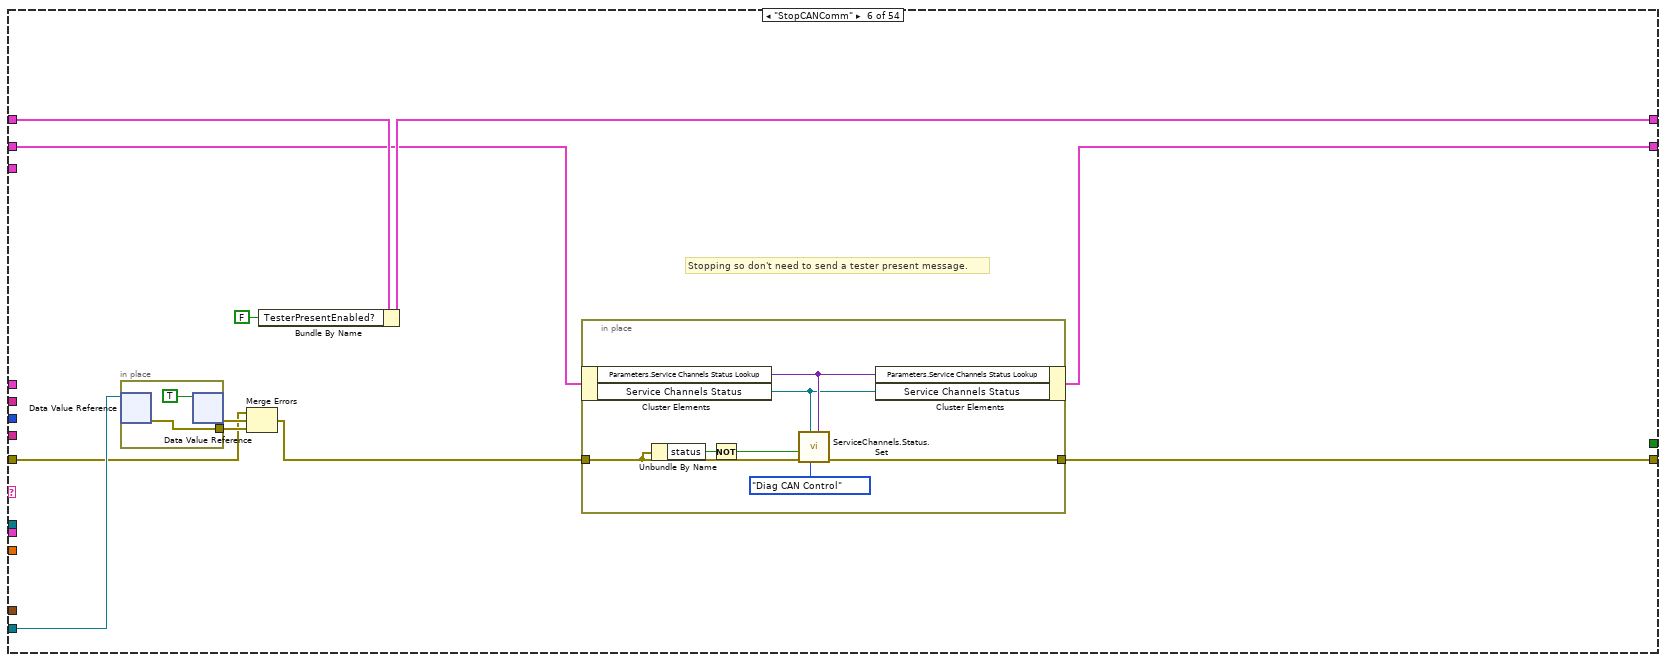
[diagram p12: hidden frame]
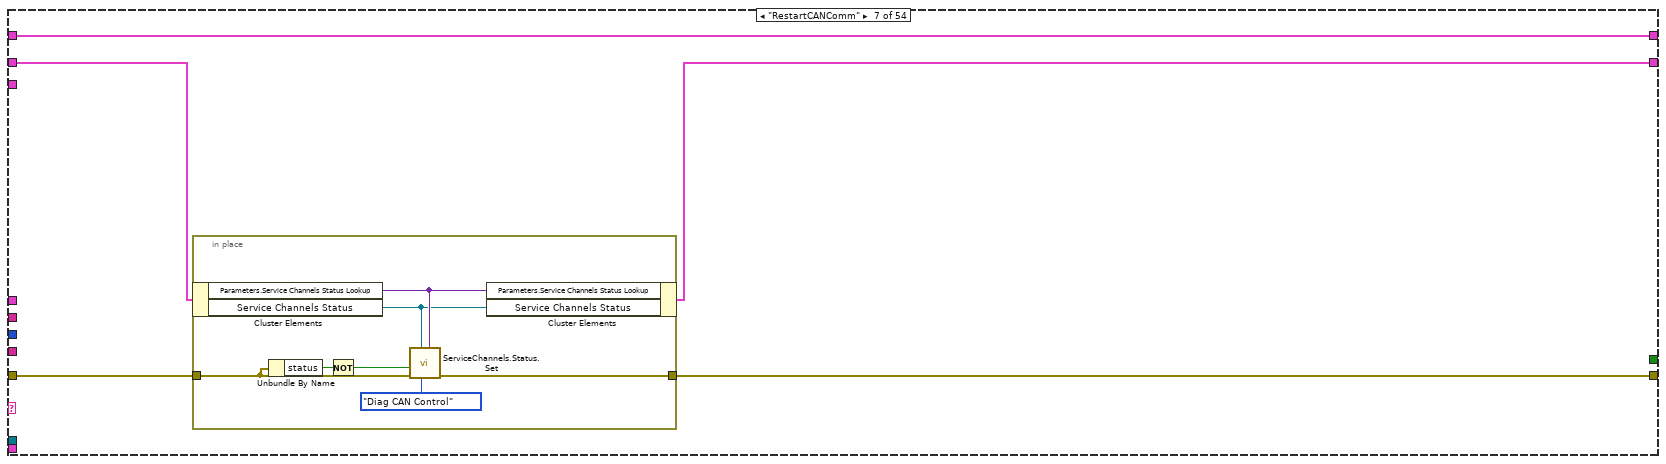
[diagram p13: hidden frame]
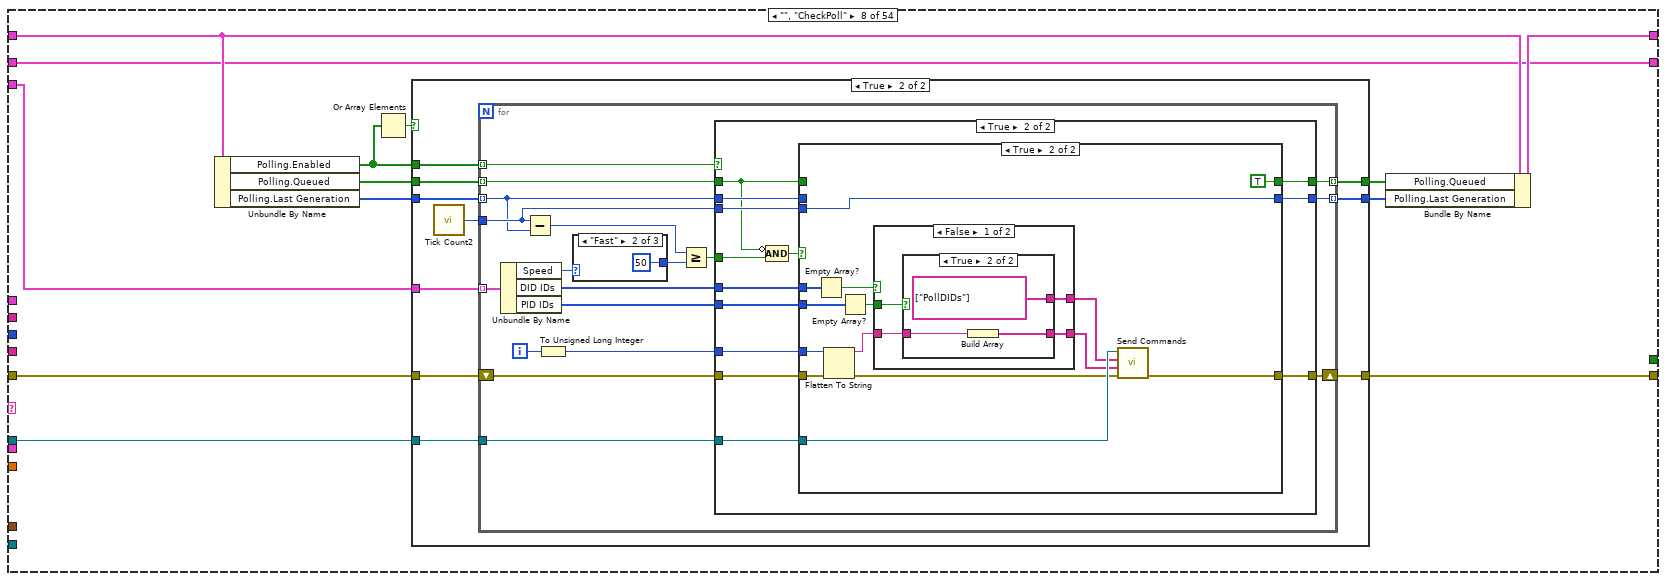
[diagram p14: hidden frame]
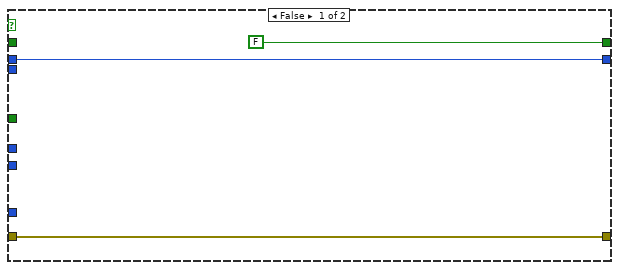
[diagram p16: hidden frame]
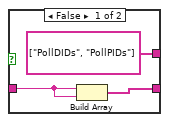
[diagram p18: hidden frame]
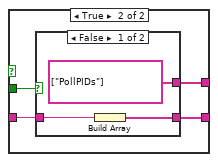
[diagram p19: hidden frame]
diagram:
  # "this global sets the number of DTC channels"
  n1 = Unbundle By Name("State Variables") -> ("Parameters.Polls"=w7:T15[], "Parameters.Reads"=w28:T8[], "Streaming Refs"=w1:T28, "Parameters.Name"=w2:string, "Parameters.CAN.Diagnostic Protocol"=w4:T5, "Comm"=w30:refnum<class "VeriStand Comm.lvclass">, "Parameters.Created DTCs"=w21:u32, "LocalStop"=w14:refnum<data-value>, "Process"=w20:refnum<class "Process.lvclass">)
  n2 = Array Size(array=w7) -> (size(s)=w8:i32)
  n3 = for {
    tunnel: w28 -> [w40] mode=indexing
    tunnel: [w33] -> w24 mode=indexing if=w37
    tunnel: [w33] -> w25 mode=indexing if=w36
    tunnel: [w33] -> w23 mode=indexing if=w32
    n4 = Unbundle By Name(w40) -> ("Type"=w35:T9, "ID"=w33:u32)
    n5 = Equal?(x=Type."Read Memory", y=w35) -> (x = y?=w32:bool)
    n6 = Equal?(x=Type."PID", y=w35) -> (x = y?=w36:bool)
    n7 = Equal?(x=Type."DID", y=w35) -> (x = y?=w37:bool)
  }
  n8 = call "Tick Count"() -> ("Tick Count(mSec)"=w11:u32)
  n9 = Initialize Array(FALSE, w8) -> (w3:bool[])
  n10 = Initialize Array(w11, w8) -> (w10:u32[])
  n11 = Initialize Array(T34 {"Timestamp"=0.0, "DTC"=0.0, "Status"=0.0, "Add Data"=0.0} ("Diagnostic Trouble Code"), w21) -> (w19:T34[])
  n12 = Bundle By Name(cluster=T33 {"Enabled"=[], "Last Generation"=[], "Queued"=[]}, "Queued"=w3, "Enabled"=w3, "Last Generation"=w10) -> (w5:T33)
  n13 = for {
    tunnel: w19 -> [w42] mode=indexing
    tunnel: [w41] -> w18 mode=concatenating
    # "Put 10 newest DTCs in VS"
    n14 = Cluster To Array(cluster=w42) -> (array=w41:dbl[])
  }
  n15 = case shown="\"User-Defined\"" w4 {
    tunnel: [FALSE ("TesterPresentEnabled?") TRUE ("TesterPresentEnabled?")] -> w22
    frame "User-Defined" {
    }
    frame Default {
    }
  }
  n16 = Bundle By Name(cluster=T35 {"Active DTCs"=[], "status mask"=0, "PID IDs"=[], "DID IDs"=[], "Memory IDs"=[], "TesterPresentEnabled?"=FALSE, "Polling"={"Enabled"=[], "Last Generation"=[], "Queued"=[]}}, "Polling"=w5, "Memory IDs"=w23, "PID IDs"=w25, "DID IDs"=w24, "TesterPresentEnabled?"=w22) -> (w26:T35)
  n17 = Array Size(array=w18) -> (size(s)=w17:i32)
  n18 = Initialize Array(0.0 ("element"), w17) -> (w15:dbl[])
  n19 = while {
    tunnel: w30 -> [w75]
    tunnel: "error in (no error)" -> [w73]
    tunnel: [w47] -> w31
    tunnel: w20 -> [w59]
    shift-right: [w61] -> _
    shift-left: w26 -> [w71]
    tunnel: w19 -> [w68]
    shift-right: [w65] -> _
    shift-left: "State Variables" -> [w67]
    tunnel: w15 -> [w57]
    tunnel: w14 -> [w51]
    tunnel: w7 -> [w50]
    tunnel: w4 -> [w49]
    tunnel: w2 -> [w46]
    tunnel: w1 -> [w45]
    stop <- w52 stop-if-true
    n20 = call <vilib>:"Read Command.vi"("error in (no error)"=w73, "timeout (100 ms)"=5 ("timeout (1ms)"), "VeriStand Comm in"=w75) -> ("error out"=w64:errorcluster, "message value"=w72:string, "message name"=w70:string, "VeriStand Comm out"=w56:refnum<class "VeriStand Comm.lvclass">, "ResponseInfo"=w69:T54)  [unwired: 3 in, 1 out]
    n21 = case shown="\"InputOutputControl\"" w70 {
      selector: w70 -> [_ w98 _ _ _ _ _ _ _ _ _ w311 _ _ _ _ _ _ _ _ _ _ _ _ _ _ _ _ _ _ _ _ _ _ _ _ w1553 _ _ w1827 _ w1930 _ _ _ _ _ _ _ _ _ _ _ _]
      tunnel: w64 -> [w91 w92 w106 w117 w128 w139 w155 w175 w268 w289 w303 w313 w374 w427 w480 w499 w540 w594 w663 w760 w830 w898 w932 w1005 w1071 w1113 w1119 w1124 w1130 w1174 w1183 w1223 w1260 w1307 w1345 w1378 w1550 w1664 w1747 w1826 w1882 w1928 w1959 w2004 w2010 w2053 w2058 w2107 w2142 w2214 w2281 w2364 w2410 w2455]
      tunnel: w72 -> [_ _ w107 _ _ _ _ _ w269 w290 _ w310 w372 w428 w477 w500 _ w590 _ w754 _ w897 _ w1001 w1070 _ _ _ w1126 _ w1181 _ w1257 _ w1341 w1377 w1551 w1660 _ w1825 w1881 w1929 w1958 _ w2011 _ w2056 w2105 w2140 w2212 w2280 w2360 w2409 w2454]
      tunnel: [w91 w93 w103 w112 w124 w134 w154 w174 w266 w287 w303 w312 w373 w426 w479 w498 w539 w593 w662 w759 w829 w896 w931 w1004 w1069 w1113 w1119 w1124 w1129 w1173 w1182 w1224 w1261 w1308 w1344 w1380 w1552 w1663 w1746 w1824 w1880 w1931 w1955 w2004 w2012 w2053 w2057 w2106 w2141 w2213 w2279 w2363 w2408 w2452] -> w63
      tunnel: [w90 w100 w109 w120 w131 w136 w156 w170 w272 w293 w305 w306 w368 w429 w478 w501 w541 w595 w666 w755 w826 w893 w933 w1006 w1072 w1115 w1117 w1121 w1132 w1175 w1184 w1225 w1262 w1309 w1346 w1373 w1544 w1658 w1743 w1821 w1883 w1933 w1960 w2006 w2014 w2055 w2061 w2108 w2143 w2215 w2282 w2365 w2411 w2457] -> w61
      tunnel: w71 -> [w90 w100 w109 w120 w131 w137 w156 w169 w271 w292 w305 w309 w369 w429 w476 w501 w541 w595 w666 w756 w826 w893 w933 w1006 w1072 w1115 w1118 w1122 w1132 w1175 w1184 w1225 w1262 w1309 w1346 w1374 w1547 w1657 w1743 w1821 w1883 w1933 w1960 w2006 w2014 w2055 w2061 w2108 w2143 w2215 w2282 w2365 w2411 w2457]
      tunnel: w69 -> [_ _ _ w111 w121 _ _ _ _ _ _ _ _ _ _ _ _ _ _ _ _ w892 _ _ _ _ _ _ _ _ _ _ _ _ _ w1379 w1554 _ _ w1820 _ w1932 _ _ w2013 _ _ _ _ _ _ _ _ _]
      tunnel: w68 -> [_ _ _ _ _ _ _ _ _ _ _ _ _ _ _ _ _ _ _ _ _ _ _ _ _ _ _ _ _ _ _ _ _ _ _ w1376 _ _ _ _ _ _ _ _ _ _ _ _ _ _ _ _ _ _]
      tunnel: w67 -> [w89 w97 w108 w119 w130 w132 w152 w164 w264 w285 w304 w308 w371 w425 w475 w497 w538 w592 w665 w758 w828 w895 w930 w1003 w1068 w1114 w1120 w1125 w1128 w1172 w1180 w1222 w1259 w1306 w1343 w1375 w1549 w1662 w1745 w1823 w1879 w1927 w1957 w2005 w2009 w2054 w2060 w2104 w2139 w2211 w2278 w2362 w2407 w2456]
      tunnel: [w89 w97 w108 w119 w130 w133 w153 w164 w265 w286 w304 w307 w370 w424 w475 w496 w537 w591 w664 w757 w827 w894 w929 w1002 w1067 w1114 w1120 w1125 w1127 w1171 w1179 w1221 w1258 w1305 w1342 w1372 w1548 w1661 w1744 w1822 w1878 w1926 w1956 w2005 w2008 w2054 w2059 w2103 w2138 w2210 w2277 w2361 w2406 w2453] -> w66
      tunnel: [_ _ _ _ _ _ _ _ _ _ _ _ _ _ _ _ _ _ _ _ _ _ _ _ _ _ _ _ TRUE _ _ _ _ _ _ _ _ _ _ _ _ _ _ _ _ _ _ _ _ _ _ _ _ _] -> w62
      tunnel: w57 -> [_ _ _ _ _ _ _ _ _ _ _ _ _ _ _ _ _ _ _ _ _ _ _ _ _ _ _ _ _ _ _ _ _ _ _ _ w1543 _ _ _ _ _ _ _ _ _ _ _ _ _ _ _ _ _]
      tunnel: w56 -> [_ _ _ w110 w122 _ _ w173 _ _ _ _ _ _ _ _ _ _ _ _ _ w891 _ _ _ _ _ _ _ _ _ _ _ _ _ w1371 w1542 _ _ w1819 _ _ _ _ w2007 _ _ _ _ _ _ _ _ _]
      tunnel: w51 -> [_ _ _ _ _ w142 _ _ _ _ _ _ _ _ _ _ _ _ _ _ _ _ _ _ _ _ _ _ _ _ _ _ _ _ _ _ _ _ _ _ _ _ _ _ _ _ _ _ _ _ _ _ _ _]
      tunnel: w50 -> [_ _ _ _ _ _ _ w172 _ _ _ _ _ _ _ _ _ _ _ w753 _ _ _ _ _ _ _ _ _ _ _ _ _ _ _ _ _ w1659 _ _ _ _ _ _ _ _ _ _ _ _ _ _ _ _]
      tunnel: w49 -> [_ _ _ _ _ _ _ _ _ _ _ _ _ _ _ _ _ _ _ _ _ _ _ _ _ _ _ _ _ _ _ _ _ _ _ _ _ _ _ _ _ _ _ _ _ _ _ _ _ _ _ _ _ _]
      tunnel: w46 -> [_ w96 _ _ _ _ _ _ _ _ _ _ _ _ _ _ _ _ _ _ _ _ _ _ _ _ _ _ _ _ _ _ _ _ _ _ _ _ _ _ _ _ _ _ _ _ _ _ _ _ _ _ _ _]
      tunnel: w45 -> [_ _ w104 w118 w129 _ _ _ _ _ _ _ _ _ _ _ _ _ _ _ _ _ _ _ _ _ _ _ _ _ _ _ _ _ _ _ _ _ _ _ _ _ _ _ _ _ _ _ _ _ _ _ _ _]
      frame "<--------------- Application ONLY --------------->" {
      }
      frame Default {
        w94 = 0 items=["Error", "Warning", "Informational"] ("severity (Informational)")
        n22 = Concatenate Strings(w98, " Not a Valid Command" ("string")) -> (w95:string)
        n23 = call "Diagnostics.FormatDebugString.vi"("error in (no error)"=w92, "State"=w95, "severity (Informational)"=w94, "Name"=w96) -> ("error out"=w93:errorcluster)  [unwired: 7 in]
      }
      frame "SetStreamingFilter" {
        n24 = Unflatten From String(type=T29 {"ID Filters"=[], "Direction Filter"=enum."Tx/Rx", "Type Filter"=enum."All"} ("Filter"), binary string=w107, error in (no error)=w106) -> (value=w101:T29, error out=w105:errorcluster)  [unwired: 2 in, 1 out]
        n25 = call "Set Engine Stream Filter.vi"("error in (no error)"=w105, "Filter"=w101, "Refs"=w104) -> ("error out"=w103:errorcluster)  [unwired: 8 in]
      }
      frame "ResetStreamingFilter" {
        n26 = call "Reset Engine Stream Filter.vi"("error in (no error)"=w117, "Refs"=w118) -> ("error out"=w113:errorcluster, "Filter"=w114:T29)  [unwired: 8 in]
        n27 = Flatten To String(anything=w114, error in (no error)=w113) -> (data string=w115:string, error out=w116:errorcluster)  [unwired: 2 in, 1 out]
        n28 = call <vilib>:"Respond to Command.vi"("error in (no error)"=w116, "message value"=w115, "ResponseInfo"=w111, "VeriStand Comm in"=w110) -> ("error out"=w112:errorcluster)  [unwired: 5 in, 2 out]
      }
      frame "GetStreamingFilter" {
        n29 = call "Get Engine Stream Filter.vi"("error in (no error)"=w128, "Refs"=w129) -> ("error out"=w125:errorcluster, "Filter"=w123:T55)  [unwired: 8 in]
        n30 = Flatten To String(anything=w123, error in (no error)=w125) -> (data string=w126:string, error out=w127:errorcluster)  [unwired: 2 in, 1 out]
        n31 = call <vilib>:"Respond to Command.vi"("error in (no error)"=w127, "message value"=w126, "ResponseInfo"=w121, "VeriStand Comm in"=w122) -> ("error out"=w124:errorcluster)  [unwired: 5 in, 2 out]
      }
      frame "StopCANComm" {
        # "Stopping so don't need to send a tester present message."
        n32 = in-place {
          in-place-border: [w150] -> w140
          n33 = in-place-dvr #1(w142) -> (w150:errorcluster)  [unwired: 1 out]
          n34 = in-place-dvr #1(TRUE ("data value")) -> (w141:errorcluster)  [unwired: 1 out]
        }
        n35 = Merge Errors(w139, w141, w140) -> (w135:errorcluster)
        n36 = Bundle By Name(cluster=w137, "TesterPresentEnabled?"=FALSE) -> (w136:T35)
        n37 = in-place {
          in-place-border: w135 -> [w146]
          in-place-border: [w148] -> w134
          n38 = in-place-cluster #2(w132) -> ("Parameters.Service Channels Status Lookup"=w147:variant, "Service Channels Status"=w143:T25)
          n39 = Unbundle By Name(w146) -> ("status"=w145:bool)
          n40 = Not(x=w145) -> (.not. x?=w144:bool)
          n41 = call "ServiceChannels.Status.Set.vi"("Status Lookup"=w147, "Type"=Type."Diag CAN Control", "Service Channels Status Ref"=w143, "error in (no error)"=w146, "Status"=w144) -> ("error out"=w148:errorcluster)  [unwired: 6 in]
          n42 = in-place-cluster #2("Parameters.Service Channels Status Lookup"=w147, "Service Channels Status"=w143) -> (w133:T1)
        }
      }
      frame "RestartCANComm" {
        n43 = in-place {
          in-place-border: w155 -> [w158]
          in-place-border: [w162] -> w154
          n44 = in-place-cluster #3(w152) -> ("Parameters.Service Channels Status Lookup"=w161:variant, "Service Channels Status"=w160:T25)
          n45 = Unbundle By Name(w158) -> ("status"=w159:bool)
          n46 = Not(x=w159) -> (.not. x?=w157:bool)
          n47 = call "ServiceChannels.Status.Set.vi"("Status Lookup"=w161, "Type"=Type."Diag CAN Control", "Service Channels Status Ref"=w160, "error in (no error)"=w158, "Status"=w157) -> ("error out"=w162:errorcluster)  [unwired: 6 in]
          n48 = in-place-cluster #3("Parameters.Service Channels Status Lookup"=w161, "Service Channels Status"=w160) -> (w153:T1)
        }
      }
      frame "", "CheckPoll" {
        n49 = Unbundle By Name(w169) -> ("Polling.Enabled"=w168:bool[], "Polling.Queued"=w165:bool[], "Polling.Last Generation"=w171:u32[])
        n50 = Or Array Elements(Boolean array=w168) -> (logical OR=w167:bool)
        n51 = case shown="True" w167 {
          tunnel: [w179 w189] -> w176
          tunnel: w175 -> [w178 w188]
          tunnel: [w178 w187] -> w174
          tunnel: w173 -> [_ w186]
          tunnel: w172 -> [_ w185]
          tunnel: w171 -> [w179 w184]
          tunnel: w168 -> [_ w183]
          tunnel: w165 -> [w177 w181]
          tunnel: [w177 w180] -> w166
          frame False {
          }
          frame True {
            n52 = call "Tick Count2"() -> ("Tick Count(mSec)"=w182:u32)
            n53 = for {
              tunnel: w185 -> [w206] mode=indexing
              tunnel: w184 -> [w194] mode=indexing
              tunnel: [w207] -> w189 mode=indexing
              shift-right: [w202] -> w187
              shift-left: w188 -> [w203]
              tunnel: w186 -> [w201]
              tunnel: w183 -> [w193] mode=indexing
              tunnel: w182 -> [w200]
              tunnel: w181 -> [w192] mode=indexing
              tunnel: [w197] -> w180 mode=indexing
              i -> [w196]
              n54 = Unbundle By Name(w206) -> ("Speed"=w205:T12, "DID IDs"=w198:u32[], "PID IDs"=w199:u32[])
              n55 = Subtract(x=w200, y=w194) -> (x-y=w195:u32)
              n56 = To Unsigned Long Integer(number=w196) -> (unsigned 32bit integer=w191:u32)
              n57 = case shown="\"Fast\"" w205 {
                tunnel: [u32 1000 ("Tick Count(mSec)") u32 50 ("Tick Count(mSec)") u32 100 ("Tick Count(mSec)")] -> w190
                frame "Slow" {
                }
                frame "Fast" {
                }
                frame "Medium" {
                }
              }
              n58 = Greater Or Equal?(x=w195, y=w190) -> (x >= y?=w204:bool)
              n59 = case shown="True" w193 {
                tunnel: w194 -> [w208 w223]
                tunnel: [w208 w222] -> w207
                tunnel: w200 -> [_ w221]
                tunnel: w204 -> [_ w213]
                tunnel: w203 -> [w210 w220]
                tunnel: [w210 w219] -> w202
                tunnel: w201 -> [_ w218]
                tunnel: w199 -> [_ w217]
                tunnel: w198 -> [_ w216]
                tunnel: w191 -> [_ w215]
                tunnel: w192 -> [_ w211]
                tunnel: [FALSE w212] -> w197
                frame False {
                }
                frame True {
                  n60 = Compound Arithmetic op=AND(invert w211, w213) -> (w214:bool)
                  n61 = case shown="True" w214 {
                    tunnel: w221 -> [_ w229]
                    tunnel: w223 -> [w224 _]
                    tunnel: [w224 w229] -> w222
                    tunnel: w220 -> [w226 w233]
                    tunnel: [w226 w240] -> w219
                    tunnel: w218 -> [_ w237]
                    tunnel: w217 -> [_ w239]
                    tunnel: w216 -> [_ w238]
                    tunnel: w215 -> [_ w227]
                    tunnel: [w225 TRUE] -> w212
                    tunnel: w211 -> [w225 _]
                    frame False {
                    }
                    frame True {
                      n62 = Empty Array?(array=w238) -> (empty?=w236:bool)
                      n63 = Flatten To String(anything=w227, error in (no error)=w233) -> (data string=w228:string, error out=w232:errorcluster)  [unwired: 2 in, 1 out]
                      n64 = Empty Array?(array=w239) -> (empty?=w235:bool)
                      n65 = case shown="False" w236 {
                        tunnel: w235 -> [w244 w254]
                        tunnel: [w243 w253] -> w234
                        tunnel: w228 -> [w242 w252]
                        tunnel: [w241 w251] -> w231
                        frame False {
                          n66 = case shown="True" w244 {
                            tunnel: [string[] ["PollDIDs", "PollPIDs"] ("message names") string[] ["PollDIDs"] ("message names")] -> w243
                            tunnel: w242 -> [w246 w249]
                            tunnel: [w245 w248] -> w241
                            frame False {
                              n67 = Build Array(w246, w246) -> (w245:string[])
                            }
                            frame True {
                              n68 = Build Array(w249) -> (w248:string[])
                            }
                          }
                        }
                        frame True {
                          n69 = case shown="False" w254 {
                            tunnel: [string[] ["PollPIDs"] ("message names") _] -> w253
                            tunnel: w252 -> [w256 _]
                            tunnel: [w255 _] -> w251
                            frame False {
                              n70 = Build Array(w256) -> (w255:string[])
                            }
                            frame True {
                            }
                          }
                        }
                      }
                      n71 = call <vilib>:"Send Commands.vi"("error in (no error)"=w232, "message values"=w231, "message names"=w234, "VeriStand Comm in"=w237) -> ("error out"=w240:errorcluster)  [unwired: 6 in, 1 out]
                    }
                  }
                }
              }
            }
          }
        }
        n72 = Bundle By Name(cluster=w169, "Polling.Queued"=w166, "Polling.Last Generation"=w176) -> (w170:T35)
      }
      frame "StopPolling" {
        n73 = Unflatten From String(type=u32 0, binary string=w269, error in (no error)=w268) -> (value=w261:u32, error out=w267:errorcluster)  [unwired: 2 in, 1 out]
        n74 = Unbundle By Name(w271) -> ("Polling.Enabled"=w263:bool[])
        n75 = Replace Array Subset(array=w263, new element=FALSE, index=w261) -> (w262:bool[])
        n76 = Bundle By Name(cluster=w271, "Polling.Enabled"=w262) -> (w272:T35)
        n77 = in-place {
          in-place-border: w267 -> [w275]
          in-place-border: [w280] -> w266
          in-place-border: w261 -> [w277]
          n78 = in-place-cluster #4(w264) -> ("Parameters.Service Channels Status Lookup"=w279:variant, "Service Channels Status"=w278:T25)
          n79 = Unbundle By Name(w275) -> ("status"=w276:bool)
          n80 = Not(x=w276) -> (.not. x?=w274:bool)
          n81 = call "ServiceChannels.Status.Set.vi"("Status Lookup"=w279, "Type"=Type."Poll Control", "Service Channels Status Ref"=w278, "error in (no error)"=w275, "Status"=w274, "ID"=w277) -> ("error out"=w280:errorcluster)  [unwired: 5 in]
          n82 = in-place-cluster #4("Parameters.Service Channels Status Lookup"=w279, "Service Channels Status"=w278) -> (w265:T1)
        }
      }
      frame "StartPolling" {
        n83 = Unflatten From String(type=u32 0, binary string=w290, error in (no error)=w289) -> (value=w282:u32, error out=w288:errorcluster)  [unwired: 2 in, 1 out]
        n84 = Unbundle By Name(w292) -> ("Polling.Enabled"=w284:bool[])
        n85 = Replace Array Subset(array=w284, new element=TRUE, index=w282) -> (w283:bool[])
        n86 = Bundle By Name(cluster=w292, "Polling.Enabled"=w283) -> (w293:T35)
        n87 = in-place {
          in-place-border: w288 -> [w299]
          in-place-border: [w301] -> w287
          in-place-border: w282 -> [w297]
          n88 = in-place-cluster #5(w285) -> ("Parameters.Service Channels Status Lookup"=w296:variant, "Service Channels Status"=w295:T25)
          n89 = Unbundle By Name(w299) -> ("status"=w300:bool)
          n90 = Not(x=w300) -> (.not. x?=w298:bool)
          n91 = call "ServiceChannels.Status.Set.vi"("Status Lookup"=w296, "Type"=Type."Poll Control", "Service Channels Status Ref"=w295, "error in (no error)"=w299, "Status"=w298, "ID"=w297) -> ("error out"=w301:errorcluster)  [unwired: 5 in]
          n92 = in-place-cluster #5("Parameters.Service Channels Status Lookup"=w296, "Service Channels Status"=w295) -> (w286:T1)
        }
      }
      frame "<--------------- GMLAN ONLY --------------->" {
      }
      frame "DTCCountChanged", "StartDTCs" {
        n93 = in-place {
          in-place-border: w313 -> [w327]
          in-place-border: [w326] -> w312
          in-place-border: w311 -> [w325]
          in-place-border: w310 -> [w324]
          n94 = in-place-cluster #6(w308) -> ("Parameters.Service Channels Status Lookup"=w315:variant, "Service Channels Status"=w316:T25, "ADCS Connection"=w322:T18, "Parameters.CAN.Diagnostic Protocol"=w320:T5)
          n95 = in-place-cluster #7(w309) -> ("status mask"=w323:u8)
          n96 = case shown="\"GMLAN\"" w320 {
            selector: w320 -> [w331 w341]
            tunnel: w327 -> [w332 w350]
            tunnel: [w332 w349] -> w326
            tunnel: w325 -> [_ w348]
            tunnel: w324 -> [_ w347]
            tunnel: w323 -> [w330 w340]
            tunnel: w322 -> [w333 w345]
            tunnel: [w333 w342] -> w321
            tunnel: [w331 w341] -> w319
            tunnel: [w330 w340] -> w318
            tunnel: [w329 w334] -> w317
            tunnel: w316 -> [w329 w334]
            tunnel: w315 -> [w328 w335]
            tunnel: [w328 w335] -> w314
            frame Default {
            }
            frame "GMLAN" {
              w358 = Property_ID."Timeout Diag Command" ("property ID")
              n97 = case shown="Default" w348 {
                tunnel: w350 -> [w362 w367]
                tunnel: w347 -> [_ w366]
                tunnel: [w361 w364] -> w353
                tunnel: [w362 w363] -> w356
                tunnel: w340 -> [w361 _]
                frame "DTCCountChanged" {
                }
                frame Default {
                  n98 = Unflatten From String(type=u8 0 ("status mask"), binary string=w366, error in (no error)=w367) -> (value=w364:u8, error out=w363:errorcluster)  [unwired: 2 in, 1 out]
                }
              }
              n99 = Number To Boolean Array(number=w353) -> (Boolean array=w352:bool[])
              n100 = Array To Cluster(array=w352) -> (cluster=w351:T56)
              n101 = call <vilib>:"Diag Get Property.vi"("error in (no error)"=w356, "property ID"=w358, "diag ref in"=w345) -> ("error out"=w360:errorcluster, "property value"=w354:u32, "diag ref out"=w346:T18)  [unwired: 6 in]
              n102 = call <vilib>:"Diag Set Property.vi"("error in (no error)"=w360, "property value"=u32 100, "property ID"=w358, "diag ref in"=w346) -> ("error out"=w355:errorcluster, "diag ref out"=w344:T18)  [unwired: 6 in]
              n103 = call "ReadDiagnosticInformation_ByStatus.vi"("error in (no error)"=w355, "status mask"=w351, "diag ref in"=w344) -> ("error out"=w339:errorcluster, "success?"=w336:bool, "diag ref out"=w343:T18)  [unwired: 5 in, 1 out]
              n104 = call "ServiceChannels.Status.Set.vi"("Status Lookup"=w335, "Type"=Type."Start DTCs", "Service Channels Status Ref"=w334, "error in (no error)"=w339, "Status"=w336) -> ("error out"=w337:errorcluster)  [unwired: 6 in]
              n105 = call <vilib>:"Diag Set Property.vi"("error in (no error)"=w337, "property value"=w354, "property ID"=Property_ID."Timeout Diag Command", "diag ref in"=w343) -> ("error out"=w349:errorcluster, "diag ref out"=w342:T18)  [unwired: 6 in]
            }
          }
          n106 = in-place-cluster #6("Parameters.Service Channels Status Lookup"=w314, "Service Channels Status"=w317, "ADCS Connection"=w321, "Parameters.CAN.Diagnostic Protocol"=w319) -> (w307:T1)
          n107 = in-place-cluster #7("status mask"=w318) -> (w306:T35)
        }
      }
      frame "DisableChangeDTCCount", "EnableChangeDTCCount" {
        n108 = in-place {
          in-place-border: w374 -> [w389]
          in-place-border: [w388] -> w373
          in-place-border: w372 -> [w387]
          n109 = in-place-cluster #8(w371) -> ("Status"=w383:T25, "Parameters.Service Channels Status Lookup"=w377:variant, "Service Channels Status"=w376:T25, "ADCS Connection"=w385:T18, "Parameters.CAN.Diagnostic Protocol"=w380:T5)
          n110 = in-place-cluster #9(w369) -> ("status mask"=w382:u8)
          n111 = case shown="\"GMLAN\"" w380 {
            selector: w380 -> [w392 w404]
            tunnel: w389 -> [w395 w413]
            tunnel: [w395 w412] -> w388
            tunnel: w387 -> [_ w411]
            tunnel: [w396 w410] -> w386
            tunnel: w385 -> [w394 w408]
            tunnel: [w394 w406] -> w384
            tunnel: w383 -> [w393 w405]
            tunnel: w382 -> [w396 _]
            tunnel: [w393 w405] -> w381
            tunnel: [w392 w404] -> w379
            tunnel: [w390 w399] -> w378
            tunnel: w377 -> [w390 w399]
            tunnel: w376 -> [w391 w398]
            tunnel: [w391 w398] -> w375
            frame Default {
            }
            frame "GMLAN" {
              w420 = Property_ID."Timeout Diag Command" ("property ID")
              n112 = Unflatten From String(type=u8 0 ("status mask"), binary string=w411, error in (no error)=w413) -> (value=w410:u8, error out=w418:errorcluster)  [unwired: 2 in, 1 out]
              n113 = Number To Boolean Array(number=w410) -> (Boolean array=w415:bool[])
              n114 = Array To Cluster(array=w415) -> (cluster=w414:T56)
              n115 = call <vilib>:"Diag Get Property.vi"("error in (no error)"=w418, "property ID"=w420, "diag ref in"=w408) -> ("error out"=w422:errorcluster, "property value"=w416:u32, "diag ref out"=w409:T18)  [unwired: 6 in]
              n116 = call <vilib>:"Diag Set Property.vi"("error in (no error)"=w422, "property value"=u32 100, "property ID"=w420, "diag ref in"=w409) -> ("error out"=w417:errorcluster, "diag ref out"=w407:T18)  [unwired: 6 in]
              n117 = call "ReadDiagnosticInformation_sendOnChangeDTCCount.vi"("error in (no error)"=w417, "status mask"=w414, "diag ref in"=w407) -> ("error out"=w403:errorcluster, "success?"=w401:bool, "diag ref out"=w397:T18)  [unwired: 5 in, 1 out]
              n118 = call "ServiceChannels.Status.Set.vi"("Status Lookup"=w399, "Type"=Type."DTC Change Count", "Service Channels Status Ref"=w398, "error in (no error)"=w403, "Status"=w401) -> ("error out"=w400:errorcluster)  [unwired: 6 in]
              n119 = call <vilib>:"Diag Set Property.vi"("error in (no error)"=w400, "property value"=w416, "property ID"=Property_ID."Timeout Diag Command", "diag ref in"=w397) -> ("error out"=w412:errorcluster, "diag ref out"=w406:T18)  [unwired: 6 in]
            }
          }
          n120 = in-place-cluster #8("Status"=w381, "Parameters.Service Channels Status Lookup"=w378, "Service Channels Status"=w375, "ADCS Connection"=w384, "Parameters.CAN.Diagnostic Protocol"=w379) -> (w370:T1)
          n121 = in-place-cluster #9("status mask"=w386) -> (w368:T35)
        }
      }
      frame "ReadFailureRecordParameters" {
        # "NOT CURRENTLY SUPPORTED"
        n122 = in-place {
          in-place-border: w428 -> [w438]
          in-place-border: w427 -> [w437]
          in-place-border: [w436] -> w426
          n123 = in-place-cluster #10(w425) -> ("Status"=w433:T25, "ADCS Connection"=w435:T18, "Parameters.CAN.Diagnostic Protocol"=w431:T5)
          n124 = case shown="\"GMLAN\"" w431 {
            selector: w431 -> [w440 w444]
            tunnel: w438 -> [_ w454]
            tunnel: w437 -> [w439 w453]
            tunnel: [w439 w452] -> w436
            tunnel: w435 -> [w441 w450]
            tunnel: [w441 w447] -> w434
            tunnel: w433 -> [w442 w445]
            tunnel: [w442 w445] -> w432
            tunnel: [w440 w444] -> w430
            frame Default {
            }
            frame "GMLAN" {
              w469 = Property_ID."Timeout Diag Command" ("property ID")
              n125 = Unflatten From String(type=T37 {"failureRecordNumber"=0, "DTC ID"=0, "DTCFailureType"=0} ("failureRecordIdentifier"), binary string=w454, error in (no error)=w453) -> (value=w455:T37, error out=w467:errorcluster)  [unwired: 2 in, 1 out]
              n126 = call <vilib>:"Diag Get Property.vi"("error in (no error)"=w467, "property ID"=w469, "diag ref in"=w450) -> ("error out"=w471:errorcluster, "property value"=w465:u32, "diag ref out"=w451:T18)  [unwired: 6 in]
              n127 = call <vilib>:"Diag Set Property.vi"("error in (no error)"=w471, "property value"=u32 1000, "property ID"=w469, "diag ref in"=w451) -> ("error out"=w466:errorcluster, "diag ref out"=w449:T18)  [unwired: 6 in]
              n128 = call "ReadFailureRecordData_readFailureRecordParameters.vi"("error in (no error)"=w466, "failureRecordIdentifier"=w455, "diag ref in"=w449) -> ("error out"=w443:errorcluster, "data out"=w446:u8[], "diag ref out"=w448:T18)  [unwired: 5 in, 1 out]
              n129 = Open/Create/Replace File(file path (use dialog)=path "C:/ReadFailureRecordParameters.txt", operation (0:open)=T38."replace or create") -> (refnum out=w459:refnum<file>, error out=w462:errorcluster)  [unwired: 4 in, 1 out]
              n130 = Array To Spreadsheet String(array=w446, 3:"%x" ("format string")) -> (spreadsheet string=w457:string)  [unwired: 1 in]
              n131 = Write to Text File(file (use dialog)=w459, text=w457, error in=w462) -> (refnum out=w458:refnum<file>, error out=w461:errorcluster)  [unwired: 1 in, 1 out]
              n132 = Close File(refnum=w458, error in=w461) -> ()  [unwired: 2 out]
              n133 = call <vilib>:"Diag Set Property.vi"("error in (no error)"=w443, "property value"=w465, "property ID"=Property_ID."Timeout Diag Command", "diag ref in"=w448) -> ("error out"=w452:errorcluster, "diag ref out"=w447:T18)  [unwired: 6 in]
            }
          }
          n134 = in-place-cluster #10("Status"=w432, "ADCS Connection"=w434, "Parameters.CAN.Diagnostic Protocol"=w430) -> (w424:T1)
        }
      }
      frame "UpdateDTCReport" {
        n135 = Unbundle By Name(w475) -> ("Parameters.CAN.Diagnostic Protocol"=w474:T5, "Parameters.Service Channels Status Lookup"=w473:variant, "Service Channels Status"=w472:T25)
        n136 = case shown="\"GMLAN\"" w474 {
          tunnel: w480 -> [w482 w493]
          tunnel: [w482 w490] -> w479
          tunnel: w476 -> [w481 w488]
          tunnel: [w481 w492] -> w478
          tunnel: w477 -> [_ w491]
          tunnel: w473 -> [_ w487]
          tunnel: w472 -> [_ w486]
          frame Default {
          }
          frame "GMLAN" {
            n137 = Unflatten From String(type=T34[] [] ("Active DTCs"), binary string=w491, error in (no error)=w493) -> (value=w495:T34[], error out=w484:errorcluster)  [unwired: 2 in, 1 out]
            n138 = Unbundle By Name(w484) -> ("status"=w485:bool)
            n139 = Not(x=w485) -> (.not. x?=w483:bool)
            n140 = call "ServiceChannels.Status.Set.vi"("Status Lookup"=w487, "Type"=Type."Start DTCs", "Service Channels Status Ref"=w486, "error in (no error)"=w484, "Status"=w483) -> ("error out"=w490:errorcluster)  [unwired: 6 in]
            n141 = Bundle By Name(cluster=w488, "Active DTCs"=w495) -> (w492:T35)
          }
        }
      }
      frame "ReadDTCByDTCNumber" {
        n142 = in-place {
          in-place-border: w500 -> [w510]
          in-place-border: w499 -> [w509]
          in-place-border: [w508] -> w498
          n143 = in-place-cluster #11(w497) -> ("Status"=w505:T25, "ADCS Connection"=w507:T18, "Parameters.CAN.Diagnostic Protocol"=w502:T5)
          n144 = case shown="\"GMLAN\"" w502 {
            selector: w502 -> [w513 w516]
            tunnel: w510 -> [_ w525]
            tunnel: w509 -> [w514 w524]
            tunnel: [w514 w523] -> w508
            tunnel: w507 -> [w512 w521]
            tunnel: [w512 w518] -> w506
            tunnel: w505 -> [w511 w517]
            tunnel: [w513 w516] -> w504
            tunnel: [w511 w517] -> w503
            frame Default {
            }
            frame "GMLAN" {
              w534 = Property_ID."Timeout Diag Command" ("property ID")
              n145 = Unflatten From String(type=T39 {"DTC"=0, "FailTypeByte"=0}, binary string=w525, error in (no error)=w524) -> (value=w528:T39, error out=w532:errorcluster)  [unwired: 2 in, 1 out]
              n146 = Unbundle By Name(w528) -> ("DTC"=w527:u16, "FailTypeByte"=w526:u8)
              n147 = call <vilib>:"Diag Get Property.vi"("error in (no error)"=w532, "property ID"=w534, "diag ref in"=w521) -> ("error out"=w536:errorcluster, "property value"=w530:u32, "diag ref out"=w522:T18)  [unwired: 6 in]
              n148 = call <vilib>:"Diag Set Property.vi"("error in (no error)"=w536, "property value"=u32 100, "property ID"=w534, "diag ref in"=w522) -> ("error out"=w531:errorcluster, "diag ref out"=w520:T18)  [unwired: 6 in]
              n149 = call "ReadDiagnosticInformation_readStatusOfDTCByDTCNumber.vi"("error in (no error)"=w531, "FailTypeByte"=w526, "DTC"=w527, "diag ref in"=w520) -> ("error out"=w515:errorcluster, "diag ref out"=w519:T18)  [unwired: 4 in, 2 out]
              n150 = call <vilib>:"Diag Set Property.vi"("error in (no error)"=w515, "property value"=w530, "property ID"=Property_ID."Timeout Diag Command", "diag ref in"=w519) -> ("error out"=w523:errorcluster, "diag ref out"=w518:T18)  [unwired: 6 in]
            }
          }
          n151 = in-place-cluster #11("Status"=w503, "ADCS Connection"=w506, "Parameters.CAN.Diagnostic Protocol"=w504) -> (w496:T1)
        }
      }
      frame "ConfigurePIDs" {
        n152 = in-place {
          in-place-border: w540 -> [w555]
          in-place-border: [w551] -> w539
          n153 = in-place-cluster #12(w538) -> ("Status"=w550:T25, "Parameters.DPIDs"=w554:T11[], "Parameters.Service Channels Status Lookup"=w544:variant, "Service Channels Status"=w542:T25, "ADCS Connection"=w553:T18, "Parameters.CAN.Diagnostic Protocol"=w549:T5)
          n154 = case shown="\"GMLAN\"" w549 {
            selector: w549 -> [w562 w571]
            tunnel: w555 -> [w560 w567]
            tunnel: w554 -> [w558 w570]
            tunnel: w553 -> [w561 w574]
            tunnel: [w561 w573] -> w552
            tunnel: [w560 w572] -> w551
            tunnel: w550 -> [w559 w564]
            tunnel: [w562 w571] -> w548
            tunnel: [w559 w564] -> w547
            tunnel: [w558 w570] -> w546
            tunnel: [w556 w568] -> w545
            tunnel: w544 -> [w556 w568]
            tunnel: [w557 w569] -> w543
            tunnel: w542 -> [w557 w569]
            frame Default {
            }
            frame "GMLAN" {
              n155 = for {
                shift-right: [w588] -> w573
                shift-left: w574 -> [w589]
                tunnel: w570 -> [w587] mode=indexing
                tunnel: [w577] -> w575 mode=indexing
                tunnel: w569 -> [w579]
                tunnel: w568 -> [w580]
                tunnel: w567 -> [w584]
                tunnel: [w581] -> w565 mode=indexing
                stop <- w582 stop-if-true
                n156 = Unbundle By Name(w587) -> ("DPID ID"=w578:u8, "PIDs"=w576:u16[])
                n157 = call "GMLAN DynamicallyDefineMessage.vi"("error in (no error)"=w584, "PID List"=w576, "DPID ID"=w578, "diag ref in"=w589) -> ("error out"=w586:errorcluster, "success?"=w577:bool, "diag ref out"=w588:T18)  [unwired: 5 in]
                n158 = call "ServiceChannels.Status.Set.vi"("Status Lookup"=w580, "Type"=Type."DPID Control", "Service Channels Status Ref"=w579, "error in (no error)"=w586, "Status"=w577, "ID"=w578) -> ("error out"=w583:errorcluster)  [unwired: 5 in]
                n159 = call "Diagnostics.CheckTimeout.vi"("error in (no error)"=w583) -> ("error out"=w581:errorcluster, "Timeout"=w582:bool)  [unwired: 9 in]
              }
              n160 = Merge Errors(w565) -> (w566:errorcluster)
              n161 = And Array Elements(Boolean array=w575) -> (logical AND=w563:bool)
              n162 = call "Status.Set.vi"("Status Ref"=w564, "error in (no error)"=w566, "Status"=w563) -> ("error out"=w572:errorcluster)  [unwired: 8 in]
            }
          }
          n163 = in-place-cluster #12("Status"=w547, "Parameters.DPIDs"=w546, "Parameters.Service Channels Status Lookup"=w545, "Service Channels Status"=w543, "ADCS Connection"=w552, "Parameters.CAN.Diagnostic Protocol"=w548) -> (w537:T1)
        }
      }
      frame "EnableDPID" {
        n164 = in-place {
          in-place-border: w594 -> [w597]
          in-place-border: [w605] -> w593
          in-place-border: w590 -> [w596]
          n165 = in-place-cluster #13(w592) -> ("Parameters.DPIDs"=w608:T11[], "Parameters.Service Channels Status Lookup"=w600:variant, "Service Channels Status"=w598:T25, "ADCS Connection"=w607:T18, "Parameters.CAN.Diagnostic Protocol"=w604:T5)
          n166 = case shown="\"GMLAN\"" w604 {
            selector: w604 -> [w614 w625]
            tunnel: w608 -> [w612 w624]
            tunnel: w607 -> [w613 w631]
            tunnel: [w613 w630] -> w606
            tunnel: [w609 w615] -> w605
            tunnel: [w614 w625] -> w603
            tunnel: [w612 w624] -> w602
            tunnel: [w610 w618] -> w601
            tunnel: w600 -> [w610 w618]
            tunnel: [w611 w617] -> w599
            tunnel: w598 -> [w611 w617]
            tunnel: w597 -> [w609 w628]
            tunnel: w596 -> [_ w627]
            frame Default {
            }
            frame "GMLAN" {
              n167 = Unflatten From String(type=u8 0 ("ID"), binary string=w627, error in (no error)=w628) -> (value=w616:u8, error out=w626:errorcluster)  [unwired: 2 in, 1 out]
              n168 = call "DPIDs.Find.vi"("ID"=w616, "DPIDs"=w624) -> ("Found"=w620:bool, "DPID"=w623:T11)  [unwired: 8 in]
              n169 = case shown="False" w620 {
                tunnel: w631 -> [w636 w648]
                tunnel: [w636 w638] -> w630
                tunnel: w626 -> [w634 w647]
                tunnel: w623 -> [_ w646]
                tunnel: [w632 w643] -> w622
                tunnel: [FALSE ("success?") w642] -> w619
                frame False {
                  n170 = Merge Errors(w634, errorcluster {"status"=TRUE, "code"=-7, "source"=""} ("error out")) -> (w632:errorcluster)
                }
                frame True {
                  n171 = Unbundle By Name(w646) -> ("Speed"=w640:T12, "DPID ID"=w639:u8, "PIDs"=w645:u16[])
                  n172 = call "GMLAN DynamicallyDefineMessage.vi"("error in (no error)"=w647, "PID List"=w645, "DPID ID"=w639, "diag ref in"=w648) -> ("error out"=w644:errorcluster, "success?"=w637:bool, "diag ref out"=w641:T18)  [unwired: 5 in]
                  n173 = case shown="False" w637 {
                    selector: w637 -> [w649 _]
                    tunnel: w644 -> [w650 w658]
                    tunnel: [w650 w657] -> w643
                    tunnel: [w649 w656] -> w642
                    tunnel: w641 -> [w651 w655]
                    tunnel: w640 -> [_ w654]
                    tunnel: w639 -> [_ w653]
                    tunnel: [w651 w652] -> w638
                    frame False {
                    }
                    frame True {
                      w660 = T40[] [enum."scheduleAtSlowRate", enum."scheduleAtMediumRate", enum."scheduleAtFastRate"] items=["stopSending", "sendOneResponse", "scheduleAtSlowRate", "scheduleAtMediumRate", "scheduleAtFastRate"]
                      n174 = Index Array(array=w660, index=w654) -> (element=w659:T40)
                      n175 = Build Array(w653) -> (w661:u8[])
                      n176 = call "GMLAN ReadDataByPacketIdentifier.vi"("error in (no error)"=w658, "DPIDs"=w661, "Sub Function"=w659, "diag ref in"=w655) -> ("error out"=w657:errorcluster, "success?"=w656:bool, "diag ref out"=w652:T18)  [unwired: 4 in, 1 out]
                    }
                  }
                }
              }
              n177 = call "ServiceChannels.Status.Set.vi"("Status Lookup"=w618, "Type"=Type."DPID Control", "Service Channels Status Ref"=w617, "error in (no error)"=w622, "Status"=w619, "ID"=w616) -> ("error out"=w615:errorcluster)  [unwired: 5 in]
            }
          }
          n178 = in-place-cluster #13("Parameters.DPIDs"=w602, "Parameters.Service Channels Status Lookup"=w601, "Service Channels Status"=w599, "ADCS Connection"=w606, "Parameters.CAN.Diagnostic Protocol"=w603) -> (w591:T1)
        }
      }
      frame "StartPIDs" {
        n179 = in-place {
          in-place-border: w663 -> [w681]
          in-place-border: [w680] -> w662
          w667 = T40[] [enum."scheduleAtSlowRate", enum."scheduleAtMediumRate", enum."scheduleAtFastRate"] items=["stopSending", "sendOneResponse", "scheduleAtSlowRate", "scheduleAtMediumRate", "scheduleAtFastRate"]
          n180 = in-place-cluster #14(w665) -> ("Status"=w676:T25, "Parameters.Service Channels Status Lookup"=w670:variant, "Service Channels Status"=w669:T25, "ADCS Connection"=w678:T18, "Parameters.DPIDs"=w679:T11[], "Parameters.CAN.Diagnostic Protocol"=w675:T5)
          n181 = case shown="\"GMLAN\"" w675 {
            selector: w675 -> [w686 w697]
            tunnel: w681 -> [w688 w708]
            tunnel: [w688 w707] -> w680
            tunnel: w679 -> [w687 w696]
            tunnel: w678 -> [w685 w703]
            tunnel: [w685 w700] -> w677
            tunnel: w676 -> [w684 w689]
            tunnel: [w686 w697] -> w674
            tunnel: [w687 w696] -> w673
            tunnel: [w684 w689] -> w672
            tunnel: [w682 w694] -> w671
            tunnel: w670 -> [w682 w694]
            tunnel: w669 -> [w683 w695]
            tunnel: [w683 w695] -> w668
            tunnel: w667 -> [_ w693]
            frame Default {
            }
            frame "GMLAN" {
              w710 = Property_ID."Timeout Diag Command" ("property ID")
              n182 = call "DPIDs.IDs.Sort.vi"("DPIDs"=w696) -> ("Filtered DPIDs IDs"=w713:T57)  [unwired: 10 in]
              n183 = call <vilib>:"Diag Get Property.vi"("error in (no error)"=w708, "property ID"=w710, "diag ref in"=w703) -> ("error out"=w712:errorcluster, "property value"=w706:u32, "diag ref out"=w704:T18)  [unwired: 6 in]
              n184 = call <vilib>:"Diag Set Property.vi"("error in (no error)"=w712, "property value"=u32 100, "property ID"=w710, "diag ref in"=w704) -> ("error out"=w692:errorcluster, "diag ref out"=w702:T18)  [unwired: 6 in]
              n185 = for {
                tunnel: w713 -> [w724]
                shift-right: [w725] -> w701
                shift-left: w702 -> [w726]
                tunnel: w693 -> [w721] mode=indexing
                tunnel: [w720] -> w705 mode=indexing
                tunnel: w695 -> [w719]
                tunnel: w694 -> [w718]
                tunnel: w692 -> [w715]
                tunnel: [w714] -> w691 mode=indexing
                stop <- w717 stop-if-true
                n186 = case shown="\"scheduleAtFastRate\"" w721 {
                  tunnel: w724 -> [w748 w750 _ w752]
                  tunnel: [w747 w749 _ w751] -> w723
                  frame "scheduleAtMediumRate" {
                    n187 = Unbundle By Name(w748) -> ("Medium"=w747:u8[])
                  }
                  frame "scheduleAtFastRate" {
                    n188 = Unbundle By Name(w750) -> ("Fast"=w749:u8[])
                  }
                  frame Default {
                  }
                  frame "scheduleAtSlowRate" {
                    n189 = Unbundle By Name(w752) -> ("Slow"=w751:u8[])
                  }
                }
                n190 = Empty Array?(array=w723) -> (empty?=w722:bool)
                n191 = case shown="False" w722 {
                  tunnel: w715 -> [w736 w745]
                  tunnel: [w731 w745] -> w716
                  tunnel: w726 -> [w735 w746]
                  tunnel: [w734 w746] -> w725
                  tunnel: w721 -> [w733 _]
                  tunnel: w723 -> [w728 _]
                  tunnel: [w727 TRUE ("success?")] -> w720
                  tunnel: w719 -> [w730 _]
                  tunnel: w718 -> [w729 _]
                  frame False {
                    n192 = call "GMLAN ReadDataByPacketIdentifier.vi"("error in (no error)"=w736, "DPIDs"=w728, "Sub Function"=w733, "diag ref in"=w735) -> ("error out"=w732:errorcluster, "success?"=w727:bool, "diag ref out"=w734:T18)  [unwired: 4 in, 1 out]
                    n193 = for {
                      tunnel: w730 -> [w739]
                      tunnel: w729 -> [w740]
                      shift-right: [w741] -> w731
                      shift-left: w732 -> [w742]
                      tunnel: w728 -> [w738] mode=indexing
                      tunnel: w727 -> [w737]
                      n194 = call "ServiceChannels.Status.Set.vi"("Status Lookup"=w740, "Type"=Type."DPID Control", "Service Channels Status Ref"=w739, "error in (no error)"=w742, "Status"=w737, "ID"=w738) -> ("error out"=w741:errorcluster)  [unwired: 5 in]
                    }
                  }
                  frame True {
                  }
                }
                n195 = call "Diagnostics.CheckTimeout.vi"("error in (no error)"=w716) -> ("error out"=w714:errorcluster, "Timeout"=w717:bool)  [unwired: 9 in]
              }
              n196 = And Array Elements(Boolean array=w705) -> (logical AND=w699:bool)
              n197 = Merge Errors(w691) -> (w690:errorcluster)
              n198 = call "Status.Set.vi"("Status Ref"=w689, "error in (no error)"=w690, "Status"=w699) -> ("error out"=w698:errorcluster)  [unwired: 8 in]
              n199 = call <vilib>:"Diag Set Property.vi"("error in (no error)"=w698, "property value"=w706, "property ID"=Property_ID."Timeout Diag Command", "diag ref in"=w701) -> ("error out"=w707:errorcluster, "diag ref out"=w700:T18)  [unwired: 6 in]
            }
          }
          n200 = in-place-cluster #14("Status"=w672, "Parameters.Service Channels Status Lookup"=w671, "Service Channels Status"=w668, "ADCS Connection"=w677, "Parameters.DPIDs"=w673, "Parameters.CAN.Diagnostic Protocol"=w674) -> (w664:T1)
        }
      }
      frame "PollPIDs" {
        n201 = in-place {
          in-place-border: w760 -> [w770]
          in-place-border: [w777] -> w759
          in-place-border: w754 -> [w769]
          in-place-border: w753 -> [w768]
          n202 = in-place-cluster #15(w756) -> ("Polling.Queued"=w772:bool[])
          n203 = in-place-cluster #16(w758) -> ("Status"=w782:T25, "Parameters.Service Channels Status Lookup"=w779:variant, "Service Channels Status"=w778:T25, "Parameters.Frames Lookup"=w785:variant, "Reads"=w763:T25, "XNETEngine (GMLAN)"=w783:T24, "ADCS Connection"=w781:T18, "Parameters.CAN.Diagnostic Protocol"=w784:T5)
          n204 = Unflatten From String(type=u32 0 ("ID"), binary string=w769, error in (no error)=w770) -> (value=w774:u32, error out=w767:errorcluster)  [unwired: 2 in, 1 out]
          n205 = Index Array(array=w768, index=w774) -> (element=w775:T15)
          n206 = Replace Array Subset(array=w772, new element=FALSE ("new element/subarray"), index=w774) -> (w771:bool[])
          n207 = Unbundle By Name(w775) -> ("PID IDs"=w766:u32[])
          n208 = case shown="\"GMLAN\"" w784 {
            tunnel: [w803 w825] -> w761
            tunnel: w767 -> [w804 w825]
            tunnel: w766 -> [w801 _]
            tunnel: w785 -> [w799 _]
            tunnel: w781 -> [w802 w824]
            tunnel: [w800 w824] -> w780
            tunnel: w783 -> [_ _]
            tunnel: w763 -> [w798 _]
            tunnel: w778 -> [w797 _]
            tunnel: w779 -> [w796 _]
            frame "GMLAN" {
              n209 = for {
                shift-right: [w808] -> w800
                shift-left: w802 -> [w823]
                tunnel: w801 -> [w811] mode=indexing
                tunnel: w799 -> [w815]
                tunnel: w798 -> [w814]
                tunnel: w797 -> [w812]
                tunnel: w796 -> [w813]
                tunnel: w804 -> [w816]
                shift-right: [w806] -> w803
                shift-left: errorcluster {"status"=FALSE, "code"=0, "source"=""} ("error IO") -> [w805]
                stop <- w817 stop-if-true
                w819 = TRUE ("Buffer?")
                w821 = Type."PID" ("Type")
                n210 = call "GMLAN ReadDataByParameterIdentifier.vi"("error in (no error)"=w816, "Parameter ID (PID)"=w811, "diag ref in"=w823) -> ("error out"=w820:errorcluster, "success?"=w809:bool, "data out"=w810:u8[], "diag ref out"=w808:T18)  [unwired: 5 in]
                n211 = call "Signals.Scale.EU.vi"("Buffer?"=w819, "Lookup"=w815, "Type"=w821, "Reads Ref"=w814, "error in (no error)"=w820, "Unscaled Data"=w810, "ID"=w811) -> ("error out"=w822:errorcluster)  [unwired: 4 in]
                n212 = call "ServiceChannels.Status.Set.vi"("Buffer?"=w819, "Status Lookup"=w813, "Type"=w821, "Service Channels Status Ref"=w812, "error in (no error)"=w822, "Status"=w809, "ID"=w811) -> ("error out"=w818:errorcluster)  [unwired: 4 in]
                n213 = call "Diagnostics.CheckTimeout.vi"("error in (no error)"=w818) -> ("error out"=w807:errorcluster, "Timeout"=w817:bool)  [unwired: 9 in]
                n214 = Merge Errors(w805, w807) -> (w806:errorcluster)
              }
            }
            frame "KWP-2000".."User-Defined" {
            }
          }
          n215 = flat-sequence {
            tunnel: w761 -> [w788]
            tunnel: w778 -> [w789]
            tunnel: [w789] -> w765
            tunnel: [w788] -> w764
            tunnel: w763 -> [w787]
            tunnel: [w786] -> w762
            tunnel: [w791] -> w777
            tunnel: w765 -> [w794]
            tunnel: w764 -> [w793]
            tunnel: w762 -> [w790]
            frame #0 {
              n216 = call-poly <vilib>:"Data.Processes.Execute.vi"("Ref"=w787) -> ("error out"=w786:errorcluster)  [unwired: 10 in]
            }
            frame #1 {
              n217 = call-poly <vilib>:"Data.Processes.Execute.vi"("Ref"=w794) -> ("error out"=w792:errorcluster)  [unwired: 10 in]
              n218 = Merge Errors(w793, w790, w792) -> (w791:errorcluster)
            }
          }
          n219 = in-place-cluster #16("Status"=w782, "Parameters.Service Channels Status Lookup"=w779, "Service Channels Status"=w778, "Parameters.Frames Lookup"=w785, "Reads"=w763, "XNETEngine (GMLAN)"=w783, "ADCS Connection"=w780, "Parameters.CAN.Diagnostic Protocol"=w784) -> (w757:T1)
          n220 = in-place-cluster #15("Polling.Queued"=w771) -> (w755:T35)
        }
      }
      frame "ReadPIDsOnDemand" {
        n221 = in-place {
          in-place-border: w830 -> [w849]
          in-place-border: [w839] -> w829
          in-place-border: w826 -> [w845]
          n222 = in-place-cluster #17(w828) -> ("Status"=w832:T25, "Parameters.Service Channels Status Lookup"=w841:variant, "Service Channels Status"=w840:T25, "Parameters.Frames Lookup"=w847:variant, "Reads"=w836:T25, "XNETEngine (GMLAN)"=w844:T24, "ADCS Connection"=w843:T18, "Parameters.CAN.Diagnostic Protocol"=w846:T5)
          n223 = Unbundle By Name(w845) -> ("PID IDs"=w848:u32[])
          n224 = case shown="\"GMLAN\"" w846 {
            tunnel: [w869 w890] -> w834
            tunnel: w849 -> [w870 w890]
            tunnel: w848 -> [w867 _]
            tunnel: w847 -> [w865 _]
            tunnel: w843 -> [w868 w889]
            tunnel: [w866 w889] -> w842
            tunnel: w844 -> [_ _]
            tunnel: w836 -> [w864 _]
            tunnel: w840 -> [w863 _]
            tunnel: w841 -> [w862 _]
            tunnel: [w861 FALSE] -> w831
            frame "GMLAN" {
              n225 = for {
                shift-right: [w885] -> w866
                shift-left: w868 -> [w886]
                tunnel: w867 -> [w873] mode=indexing
                tunnel: w865 -> [w877]
                tunnel: w864 -> [w874]
                tunnel: w863 -> [w876]
                tunnel: w862 -> [w878]
                tunnel: w870 -> [w887]
                tunnel: [w879] -> w860 mode=indexing
                tunnel: [w871] -> w859 mode=indexing
                stop <- w880 stop-if-true
                w882 = TRUE ("Buffer?")
                w884 = Type."PID" ("Type")
                n226 = call "GMLAN ReadDataByParameterIdentifier.vi"("error in (no error)"=w887, "Parameter ID (PID)"=w873, "diag ref in"=w886) -> ("error out"=w883:errorcluster, "success?"=w871:bool, "data out"=w872:u8[], "diag ref out"=w885:T18)  [unwired: 5 in]
                n227 = call "Signals.Scale.EU.vi"("Buffer?"=w882, "Lookup"=w877, "Type"=w884, "Reads Ref"=w874, "error in (no error)"=w883, "Unscaled Data"=w872, "ID"=w873) -> ("error out"=w875:errorcluster)  [unwired: 4 in]
                n228 = call "ServiceChannels.Status.Set.vi"("Buffer?"=w882, "Status Lookup"=w878, "Type"=w884, "Service Channels Status Ref"=w876, "error in (no error)"=w875, "Status"=w871, "ID"=w873) -> ("error out"=w881:errorcluster)  [unwired: 4 in]
                n229 = call "Diagnostics.CheckTimeout.vi"("error in (no error)"=w881) -> ("error out"=w879:errorcluster, "Timeout"=w880:bool)  [unwired: 9 in]
              }
              n230 = And Array Elements(Boolean array=w859) -> (logical AND=w861:bool)
              n231 = Merge Errors(w860) -> (w869:errorcluster)
            }
            frame "KWP-2000".."User-Defined" {
            }
          }
          n232 = call "Status.Set.vi"("Status Ref"=w832, "error in (no error)"=w834, "Status"=w831) -> ("error out"=w833:errorcluster)  [unwired: 8 in]
          n233 = flat-sequence {
            tunnel: w833 -> [w852]
            tunnel: w840 -> [w853]
            tunnel: [w853] -> w838
            tunnel: [w852] -> w837
            tunnel: w836 -> [w851]
            tunnel: [w850] -> w835
            tunnel: [w855] -> w839
            tunnel: w838 -> [w858]
            tunnel: w837 -> [w857]
            tunnel: w835 -> [w854]
            frame #0 {
              n234 = call-poly <vilib>:"Data.Processes.Execute.vi"("Ref"=w851) -> ("error out"=w850:errorcluster)  [unwired: 10 in]
            }
            frame #1 {
              n235 = call-poly <vilib>:"Data.Processes.Execute.vi"("Ref"=w858) -> ("error out"=w856:errorcluster)  [unwired: 10 in]
              n236 = Merge Errors(w857, w854, w856) -> (w855:errorcluster)
            }
          }
          n237 = in-place-cluster #17("Status"=w832, "Parameters.Service Channels Status Lookup"=w841, "Service Channels Status"=w840, "Parameters.Frames Lookup"=w847, "Reads"=w836, "XNETEngine (GMLAN)"=w844, "ADCS Connection"=w842, "Parameters.CAN.Diagnostic Protocol"=w846) -> (w827:T1)
        }
      }
      frame "ReadPIDOnDemand" {
        n238 = in-place {
          in-place-border: w898 -> [w911]
          in-place-border: w897 -> [w910]
          in-place-border: [w899] -> w896
          in-place-border: w892 -> [_]
          in-place-border: w891 -> [_]
          n239 = in-place-cluster #18(w895) -> ("Parameters.Service Channels Status Lookup"=w900:variant, "Service Channels Status"=w901:T25, "Parameters.Frames Lookup"=w909:variant, "Reads"=w902:T25, "XNETEngine (GMLAN)"=w907:T24, "ADCS Connection"=w904:T18, "Parameters.CAN.Diagnostic Protocol"=w908:T5)
          n240 = Unflatten From String(type=u16 0 ("ID"), binary string=w910, error in (no error)=w911) -> (value=w905:u16, error out=w912:errorcluster)  [unwired: 2 in, 1 out]
          n241 = case shown="\"GMLAN\"" w908 {
            tunnel: [w923 w928] -> w899
            tunnel: w912 -> [w926 w928]
            tunnel: w905 -> [w916 _]
            tunnel: w909 -> [w918 _]
            tunnel: w904 -> [w925 w927]
            tunnel: [w914 w927] -> w903
            tunnel: w902 -> [w917 _]
            tunnel: w901 -> [w919 _]
            tunnel: w900 -> [w920 _]
            frame "GMLAN" {
              w921 = Type."PID" ("Type")
              n242 = call "GMLAN ReadDataByParameterIdentifier.vi"("error in (no error)"=w926, "Parameter ID (PID)"=w916, "diag ref in"=w925) -> ("error out"=w924:errorcluster, "success?"=w915:bool, "data out"=w913:u8[], "diag ref out"=w914:T18)  [unwired: 5 in]
              n243 = call "Signals.Scale.EU.vi"("Lookup"=w918, "Type"=w921, "Reads Ref"=w917, "error in (no error)"=w924, "Unscaled Data"=w913, "ID"=w916) -> ("error out"=w922:errorcluster)  [unwired: 5 in]
              n244 = call "ServiceChannels.Status.Set.vi"("Status Lookup"=w920, "Type"=w921, "Service Channels Status Ref"=w919, "error in (no error)"=w922, "Status"=w915, "ID"=w916) -> ("error out"=w923:errorcluster)  [unwired: 5 in]
            }
            frame "KWP-2000".."User-Defined" {
            }
          }
          n245 = in-place-cluster #18("Parameters.Service Channels Status Lookup"=w900, "Service Channels Status"=w901, "Parameters.Frames Lookup"=w909, "Reads"=w902, "XNETEngine (GMLAN)"=w907, "ADCS Connection"=w903, "Parameters.CAN.Diagnostic Protocol"=w908) -> (w894:T1)
        }
      }
      frame "StopPIDs" {
        n246 = in-place {
          in-place-border: w932 -> [w947]
          in-place-border: [w946] -> w931
          n247 = in-place-cluster #19(w930) -> ("Status"=w945:T25, "Parameters.Service Channels Status Lookup"=w936:variant, "Service Channels Status"=w934:T25, "ADCS Connection"=w943:T18, "Parameters.DPIDs"=w944:T11[], "Parameters.CAN.Diagnostic Protocol"=w939:T5)
          n248 = case shown="\"GMLAN\"" w939 {
            selector: w939 -> [w950 w958]
            tunnel: w947 -> [w951 w974]
            tunnel: [w951 w972] -> w946
            tunnel: w945 -> [w952 w955]
            tunnel: w944 -> [w954 w959]
            tunnel: w943 -> [w953 w965]
            tunnel: [w953 w962] -> w942
            tunnel: [w952 w955] -> w941
            tunnel: [w954 w959] -> w940
            tunnel: [w950 w958] -> w938
            tunnel: [w948 w956] -> w937
            tunnel: w936 -> [w948 w956]
            tunnel: [w949 w957] -> w935
            tunnel: w934 -> [w949 w957]
            frame Default {
            }
            frame "GMLAN" {
              w976 = Property_ID."Timeout Diag Command" ("property ID")
              n249 = for {
                tunnel: w959 -> [w1000] mode=indexing
                tunnel: [w999] -> w969 mode=indexing
                n250 = Unbundle By Name(w1000) -> ("DPID ID"=w999:u8)
              }
              n251 = call <vilib>:"Diag Get Property.vi"("error in (no error)"=w974, "property ID"=w976, "diag ref in"=w965) -> ("error out"=w978:errorcluster, "property value"=w971:u32, "diag ref out"=w966:T18)  [unwired: 6 in]
              n252 = call <vilib>:"Diag Set Property.vi"("error in (no error)"=w978, "property value"=u32 100, "property ID"=w976, "diag ref in"=w966) -> ("error out"=w973:errorcluster, "diag ref out"=w964:T18)  [unwired: 6 in]
              n253 = Empty Array?(array=w969) -> (empty?=w970:bool)
              n254 = case shown="True" w970 {
                tunnel: w973 -> [w988 w997]
                tunnel: [w983 w997] -> w961
                tunnel: w964 -> [w987 w998]
                tunnel: [w986 w998] -> w963
                tunnel: ReadDataByPacketIdentifier_SubFunctions."stopSending" ("Sub Function") -> [w985 _]
                tunnel: w969 -> [w980 _]
                tunnel: [w979 TRUE ("success?")] -> w960
                tunnel: w957 -> [w982 _]
                tunnel: w956 -> [w981 _]
                frame False {
                  n255 = call "GMLAN ReadDataByPacketIdentifier.vi"("error in (no error)"=w988, "DPIDs"=w980, "Sub Function"=w985, "diag ref in"=w987) -> ("error out"=w984:errorcluster, "success?"=w979:bool, "diag ref out"=w986:T18)  [unwired: 4 in, 1 out]
                  n256 = for {
                    tunnel: w982 -> [w991]
                    tunnel: w981 -> [w992]
                    shift-right: [w993] -> w983
                    shift-left: w984 -> [w994]
                    tunnel: w980 -> [w990] mode=indexing
                    tunnel: w979 -> [w989]
                    n257 = call "ServiceChannels.Status.Set.vi"("Status Lookup"=w992, "Type"=Type."DPID Control", "Service Channels Status Ref"=w991, "error in (no error)"=w994, "Status"=w989, "ID"=w990) -> ("error out"=w993:errorcluster)  [unwired: 5 in]
                  }
                }
                frame True {
                }
              }
              n258 = call "Status.Set.vi"("Status Ref"=w955, "error in (no error)"=w961, "Status"=w960) -> ("error out"=w968:errorcluster)  [unwired: 8 in]
              n259 = call <vilib>:"Diag Set Property.vi"("error in (no error)"=w968, "property value"=w971, "property ID"=Property_ID."Timeout Diag Command", "diag ref in"=w963) -> ("error out"=w972:errorcluster, "diag ref out"=w962:T18)  [unwired: 6 in]
            }
          }
          n260 = in-place-cluster #19("Status"=w941, "Parameters.Service Channels Status Lookup"=w937, "Service Channels Status"=w935, "ADCS Connection"=w942, "Parameters.DPIDs"=w940, "Parameters.CAN.Diagnostic Protocol"=w938) -> (w929:T1)
        }
      }
      frame "DisableDPID" {
        n261 = in-place {
          in-place-border: w1005 -> [w1008]
          in-place-border: [w1019] -> w1004
          in-place-border: w1001 -> [w1007]
          n262 = in-place-cluster #20(w1003) -> ("Parameters.Service Channels Status Lookup"=w1012:variant, "Service Channels Status"=w1010:T25, "ADCS Connection"=w1018:T18, "Parameters.DPIDs"=w1009:T11[], "Parameters.CAN.Diagnostic Protocol"=w1015:T5)
          n263 = case shown="\"GMLAN\"" w1015 {
            selector: w1015 -> [w1022 w1042]
            tunnel: w1008 -> [w1023 w1039]
            tunnel: [w1023 w1049] -> w1019
            tunnel: w1009 -> [w1025 w1037]
            tunnel: w1018 -> [w1024 w1046]
            tunnel: [w1024 w1043] -> w1017
            tunnel: [w1025 w1037] -> w1016
            tunnel: [w1022 w1042] -> w1014
            tunnel: [w1020 w1029] -> w1013
            tunnel: w1012 -> [w1020 w1029]
            tunnel: [w1021 w1028] -> w1011
            tunnel: w1010 -> [w1021 w1028]
            tunnel: w1007 -> [_ w1038]
            frame Default {
            }
            frame "GMLAN" {
              w1052 = Property_ID."Timeout Diag Command" ("property ID")
              n264 = Unflatten From String(type=u8 0 ("ID"), binary string=w1038, error in (no error)=w1039) -> (value=w1027:u8, error out=w1040:errorcluster)  [unwired: 2 in, 1 out]
              n265 = call "DPIDs.Find.vi"("ID"=w1027, "DPIDs"=w1037) -> ("Found"=w1031:bool, "DPID"=w1035:T11)  [unwired: 8 in]
              n266 = call <vilib>:"Diag Get Property.vi"("error in (no error)"=w1040, "property ID"=w1052, "diag ref in"=w1046) -> ("error out"=w1054:errorcluster, "property value"=w1032:u32, "diag ref out"=w1047:T18)  [unwired: 6 in]
              n267 = Unbundle By Name(w1035) -> ("DPID ID"=w1048:u8)
              n268 = call <vilib>:"Diag Set Property.vi"("error in (no error)"=w1054, "property value"=u32 100, "property ID"=w1052, "diag ref in"=w1047) -> ("error out"=w1050:errorcluster, "diag ref out"=w1045:T18)  [unwired: 6 in]
              n269 = Build Array(w1048) -> (w1036:u8[])
              n270 = case shown="False" w1031 {
                tunnel: w1050 -> [w1056 w1066]
                tunnel: w1045 -> [w1059 w1064]
                tunnel: [w1059 w1063] -> w1044
                tunnel: [FALSE ("success?") w1062] -> w1026
                tunnel: w1036 -> [_ w1061]
                tunnel: [w1055 w1060] -> w1033
                frame False {
                  n271 = Merge Errors(w1056, errorcluster {"status"=TRUE, "code"=-7, "source"=""} ("error out")) -> (w1055:errorcluster)
                }
                frame True {
                  n272 = call "GMLAN ReadDataByPacketIdentifier.vi"("error in (no error)"=w1066, "DPIDs"=w1061, "Sub Function"=ReadDataByPacketIdentifier_SubFunctions."stopSending", "diag ref in"=w1064) -> ("error out"=w1060:errorcluster, "success?"=w1062:bool, "diag ref out"=w1063:T18)  [unwired: 4 in, 1 out]
                }
              }
              n273 = call "ServiceChannels.Status.Set.vi"("Status Lookup"=w1029, "Type"=Type."DPID Control", "Service Channels Status Ref"=w1028, "error in (no error)"=w1033, "Status"=w1026, "ID"=w1027) -> ("error out"=w1030:errorcluster)  [unwired: 5 in]
              n274 = call <vilib>:"Diag Set Property.vi"("error in (no error)"=w1030, "property value"=w1032, "property ID"=Property_ID."Timeout Diag Command", "diag ref in"=w1044) -> ("error out"=w1049:errorcluster, "diag ref out"=w1043:T18)  [unwired: 6 in]
            }
          }
          n275 = in-place-cluster #20("Parameters.Service Channels Status Lookup"=w1013, "Service Channels Status"=w1011, "ADCS Connection"=w1017, "Parameters.DPIDs"=w1016, "Parameters.CAN.Diagnostic Protocol"=w1014) -> (w1002:T1)
        }
      }
      frame "GenerateCPID" {
        n276 = in-place {
          in-place-border: w1071 -> [w1087]
          in-place-border: w1070 -> [w1086]
          in-place-border: [w1080] -> w1069
          n277 = in-place-cluster #21(w1068) -> ("Parameters.Service Channels Status Lookup"=w1076:variant, "Service Channels Status"=w1075:T25, "ADCS Connection"=w1085:T18, "Parameters.CAN.Diagnostic Protocol"=w1079:T5, "Parameters.Frames Lookup"=w1083:variant, "Writes"=w1082:T26)
          n278 = case shown="\"GMLAN\"" w1079 {
            selector: w1079 -> [w1093 w1106]
            tunnel: w1087 -> [w1090 w1112]
            tunnel: w1086 -> [_ w1111]
            tunnel: w1085 -> [w1094 w1110]
            tunnel: [w1094 w1109] -> w1084
            tunnel: w1083 -> [w1092 w1099]
            tunnel: w1082 -> [w1091 w1098]
            tunnel: [w1091 w1098] -> w1081
            tunnel: [w1090 w1102] -> w1080
            tunnel: [w1093 w1106] -> w1078
            tunnel: [w1092 w1099] -> w1077
            tunnel: w1076 -> [w1088 w1101]
            tunnel: w1075 -> [w1089 w1100]
            tunnel: [w1088 w1101] -> w1074
            tunnel: [w1089 w1100] -> w1073
            frame Default {
            }
            frame "GMLAN" {
              w1103 = Type."CPID" ("Type")
              n279 = Unflatten From String(type=u16 0, binary string=w1111, error in (no error)=w1112) -> (value=w1097:u16, error out=w1105:errorcluster)  [unwired: 2 in, 1 out]
              n280 = call "Signals.Scale.Raw.vi"("Lookup"=w1099, "Type"=w1103, "Writes Ref"=w1098, "error in"=w1105, "ID"=w1097) -> ("error out"=w1107:errorcluster, "Data"=w1095:u8[])  [unwired: 5 in]
              n281 = call "GMLAN DeviceControl.vi"("error in (no error)"=w1107, "CPIDControlBytes"=w1095, "CPID ID"=w1097, "diag ref in"=w1110) -> ("error out"=w1104:errorcluster, "success?"=w1096:bool, "diag ref out"=w1109:T18)  [unwired: 5 in]
              n282 = call "ServiceChannels.Status.Set.vi"("Status Lookup"=w1101, "Type"=w1103, "Service Channels Status Ref"=w1100, "error in (no error)"=w1104, "Status"=w1096, "ID"=w1097) -> ("error out"=w1102:errorcluster)  [unwired: 5 in]
            }
          }
          n283 = in-place-cluster #21("Parameters.Service Channels Status Lookup"=w1074, "Service Channels Status"=w1073, "ADCS Connection"=w1084, "Parameters.CAN.Diagnostic Protocol"=w1078, "Parameters.Frames Lookup"=w1077, "Writes"=w1081) -> (w1067:T1)
        }
      }
      frame "<--------------- GENERIC SERVICES --------------->" {
      }
      frame "DisableRepeatingTesterPresent" {
        n284 = Bundle By Name(cluster=w1118, "TesterPresentEnabled?"=FALSE) -> (w1117:T35)
      }
      frame "EnableRepeatingTesterPresent" {
        n285 = Bundle By Name(cluster=w1122, "TesterPresentEnabled?"=TRUE) -> (w1121:T35)
      }
      frame "ForceTesterPresent" {
        n286 = in-place {
          in-place-border: w1130 -> [w1142]
          in-place-border: [w1136] -> w1129
          in-place-border: w1126 -> [w1139]
          n287 = in-place-cluster #22(w1128) -> ("Parameters.Service Channels Status Lookup"=w1135:variant, "Service Channels Status"=w1134:T25, "Parameters.CAN.Diagnostic Protocol"=w1144:T5, "ADCS Connection"=w1146:T18)
          n288 = Unflatten From String(type=FALSE, binary string=w1139, error in (no error)=w1142) -> (value=w1140:bool, error out=w1141:errorcluster)  [unwired: 2 in, 1 out]
          n289 = case shown="\"KWP-2000\"" w1144 {
            tunnel: w1141 -> [w1148 w1155 w1158 w1165]
            tunnel: [w1147 w1155 w1157 w1167] -> w1137
            tunnel: w1146 -> [w1152 w1153 w1164 w1170]
            tunnel: [w1151 w1153 w1163 w1169] -> w1145
            tunnel: w1140 -> [w1150 _ w1160 w1168]
            tunnel: [w1149 FALSE ("success?") w1156 w1166] -> w1133
            frame "KWP-2000" {
              n290 = call <vilib>:"TesterPresent.vi"("error in (no error)"=w1148, "response required?"=w1150, "diag ref in"=w1152) -> ("error out"=w1147:errorcluster, "success?"=w1149:bool, "diag ref out"=w1151:T18)  [unwired: 6 in]
            }
            frame "User-Defined" {
            }
            frame "GMLAN" {
              n291 = Select(t=TesterPresent_Parameter."SpecificECU" ("Parameter"), s=w1160, f=TesterPresent_Parameter."EntireNetwork" ("Parameter")) -> (s? t:f=w1159:T41)
              n292 = call "GMLAN TesterPresent.vi"("error in (no error)"=w1158, "Parameter"=w1159, "diag ref in"=w1164) -> ("error out"=w1157:errorcluster, "success?"=w1156:bool, "diag ref out"=w1163:T18)  [unwired: 6 in]
            }
            frame "UDS" {
              n293 = call <vilib>:"UDS TesterPresent.vi"("error in (no error)"=w1165, "response required?"=w1168, "diag ref in"=w1170) -> ("error out"=w1167:errorcluster, "success?"=w1166:bool, "diag ref out"=w1169:T18)  [unwired: 6 in]
            }
          }
          n294 = call "ServiceChannels.Status.Set.vi"("Status Lookup"=w1135, "Type"=Type."Tester Present", "Service Channels Status Ref"=w1134, "error in (no error)"=w1137, "Status"=w1133) -> ("error out"=w1136:errorcluster)  [unwired: 6 in]
          n295 = in-place-cluster #22("Parameters.Service Channels Status Lookup"=w1135, "Service Channels Status"=w1134, "Parameters.CAN.Diagnostic Protocol"=w1144, "ADCS Connection"=w1145) -> (w1127:T1)
        }
      }
      frame "ClearSuccessBit" {
        n296 = in-place {
          in-place-border: w1174 -> [w1178]
          in-place-border: [w1177] -> w1173
          n297 = in-place-cluster #23(w1172) -> ("Status"=w1176:T25)
          n298 = call "Status.Set.vi"("Status Ref"=w1176, "error in (no error)"=w1178) -> ("error out"=w1177:errorcluster)  [unwired: 9 in]
          n299 = in-place-cluster #23("Status"=w1176) -> (w1171:T1)
        }
      }
      frame "EnableDiagnosticSession" {
        n300 = in-place {
          in-place-border: w1183 -> [w1195]
          in-place-border: [w1185] -> w1182
          in-place-border: w1181 -> [w1194]
          n301 = in-place-cluster #24(w1180) -> ("Parameters.Service Channels Status Lookup"=w1188:variant, "Service Channels Status"=w1186:T25, "Parameters.CAN.Diagnostic Protocol"=w1191:T5, "ADCS Connection"=w1193:T18)
          n302 = Unflatten From String(type=u8 0 ("ID"), binary string=w1194, error in (no error)=w1195) -> (value=w1197:u8, error out=w1196:errorcluster)  [unwired: 2 in, 1 out]
          n303 = case shown="\"User-Defined\"" w1191 {
            tunnel: [w1202 w1208 w1214 w1217] -> w1189
            tunnel: [w1204 FALSE ("success?") w1213 w1216] -> w1187
            tunnel: w1197 -> [w1199 _ w1212 w1219]
            tunnel: w1196 -> [w1203 w1208 w1211 w1218]
            tunnel: w1193 -> [w1201 w1207 w1210 w1220]
            tunnel: [w1200 w1207 w1209 w1215] -> w1192
            frame "GMLAN" {
              n304 = call "GMLAN InitiateDiagnosticOperation.vi"("error in (no error)"=w1203, "SubFunctions"=w1199, "Parameter"=InitiateDiagnosticOperation_Parameter."SpecificECU", "diag ref in"=w1201) -> ("error out"=w1202:errorcluster, "success?"=w1204:bool, "diag ref out"=w1200:T18)  [unwired: 5 in]
            }
            frame "User-Defined" {
            }
            frame "UDS" {
              n305 = call <vilib>:"UDS DiagnosticSessionControl.vi"("error in (no error)"=w1211, "mode"=w1212, "diag ref in"=w1210) -> ("error out"=w1214:errorcluster, "success?"=w1213:bool, "diag ref out"=w1209:T18)  [unwired: 5 in, 1 out]
            }
            frame "KWP-2000" {
              n306 = call <vilib>:"StartDiagnosticSession.vi"("error in (no error)"=w1218, "mode"=w1219, "diag ref in"=w1220) -> ("error out"=w1217:errorcluster, "success?"=w1216:bool, "diag ref out"=w1215:T18)  [unwired: 6 in]
            }
          }
          n307 = call "ServiceChannels.Status.Set.vi"("Status Lookup"=w1188, "Type"=Type."Diag Session Control", "Service Channels Status Ref"=w1186, "error in (no error)"=w1189, "Status"=w1187) -> ("error out"=w1185:errorcluster)  [unwired: 6 in]
          n308 = in-place-cluster #24("Parameters.Service Channels Status Lookup"=w1188, "Service Channels Status"=w1186, "Parameters.CAN.Diagnostic Protocol"=w1191, "ADCS Connection"=w1192) -> (w1179:T1)
        }
      }
      frame "DisableDiagnosticSession" {
        n309 = in-place {
          in-place-border: [w1227] -> w1224
          in-place-border: w1223 -> [w1235]
          n310 = in-place-cluster #25(w1222) -> ("Parameters.Service Channels Status Lookup"=w1229:variant, "Service Channels Status"=w1226:T25, "Parameters.CAN.Diagnostic Protocol"=w1232:T5, "ADCS Connection"=w1234:T18)
          n311 = case shown="\"User-Defined\"" w1232 {
            tunnel: [w1238 w1244 w1247 w1256] -> w1230
            tunnel: [w1240 FALSE ("success?") w1246 w1255] -> w1228
            tunnel: w1235 -> [w1237 w1244 w1250 w1253]
            tunnel: w1234 -> [w1236 w1245 w1249 w1252]
            tunnel: [w1239 w1245 w1248 w1251] -> w1233
            frame "GMLAN" {
              w1241 = T58 2 items=["disableAllDTCs"=2, "enableDTCsDuringDevCntrl"=3, "wakeUpLinks"=4] ("SubFunctions")
              n312 = call "GMLAN InitiateDiagnosticOperation.vi"("error in (no error)"=w1237, "SubFunctions"=w1241, "Parameter"=InitiateDiagnosticOperation_Parameter."SpecificECU", "diag ref in"=w1236) -> ("error out"=w1238:errorcluster, "success?"=w1240:bool, "diag ref out"=w1239:T18)  [unwired: 5 in]
            }
            frame "User-Defined" {
            }
            frame "KWP-2000" {
              n313 = call <vilib>:"StopDiagnosticSession.vi"("error in (no error)"=w1250, "diag ref in"=w1249) -> ("error out"=w1247:errorcluster, "success?"=w1246:bool, "diag ref out"=w1248:T18)  [unwired: 7 in]
            }
            frame "UDS" {
              n314 = call <vilib>:"UDS DiagnosticSessionControl.vi"("error in (no error)"=w1253, "mode"=u8 1, "diag ref in"=w1252) -> ("error out"=w1256:errorcluster, "success?"=w1255:bool, "diag ref out"=w1251:T18)  [unwired: 5 in, 1 out]
            }
          }
          n315 = call "ServiceChannels.Status.Set.vi"("Status Lookup"=w1229, "Type"=Type."Diag Session Control", "Service Channels Status Ref"=w1226, "error in (no error)"=w1230, "Status"=w1228) -> ("error out"=w1227:errorcluster)  [unwired: 6 in]
          n316 = in-place-cluster #25("Parameters.Service Channels Status Lookup"=w1229, "Service Channels Status"=w1226, "Parameters.CAN.Diagnostic Protocol"=w1232, "ADCS Connection"=w1233) -> (w1221:T1)
        }
      }
      frame "DisableNormalCommunication" {
        n317 = in-place {
          in-place-border: [w1265] -> w1261
          in-place-border: w1260 -> [w1274]
          in-place-border: w1257 -> [w1272]
          n318 = in-place-cluster #26(w1259) -> ("Parameters.Service Channels Status Lookup"=w1264:variant, "Service Channels Status"=w1263:T25, "Parameters.CAN.Diagnostic Protocol"=w1276:T5, "ADCS Connection"=w1278:T18)
          n319 = Unflatten From String(type=T43 {"Type"=0, "CommType"=0} ("Cluster"), binary string=w1272, error in (no error)=w1274) -> (value=w1275:T43, error out=w1273:errorcluster)  [unwired: 2 in, 1 out]
          n320 = Unbundle By Name(w1275) -> ("Type"=w1270:u8, "CommType"=w1269:u8)
          n321 = case shown="\"GMLAN\"" w1276 {
            tunnel: w1278 -> [w1284 w1290 w1298 w1303]
            tunnel: [w1285 w1290 w1297 w1302] -> w1277
            tunnel: [w1287 w1291 w1296 w1300] -> w1267
            tunnel: [w1286 FALSE ("success?") w1295 w1301] -> w1266
            tunnel: w1273 -> [w1288 w1291 w1294 w1304]
            tunnel: w1270 -> [w1283 _ w1293 _]
            tunnel: w1269 -> [_ _ w1292 _]
            frame "GMLAN" {
              n322 = Not Equal To 0?(x=w1283) -> (x != 0?=w1282:bool)
              n323 = Select(t=DisableNormalCommunication_Parameter."SpecificECU" ("Parameter"), s=w1282, f=DisableNormalCommunication_Parameter."EntireNetwork" ("Parameter")) -> (s? t:f=w1280:T44)
              n324 = call "GMLAN DisableNormalCommunication.vi"("error in (no error)"=w1288, "Parameter"=w1280, "diag ref in"=w1284) -> ("error out"=w1287:errorcluster, "success?"=w1286:bool, "diag ref out"=w1285:T18)  [unwired: 6 in]
            }
            frame "User-Defined" {
            }
            frame "UDS" {
              n325 = call <vilib>:"UDS CommunicationControl.vi"("error in (no error)"=w1294, "communication type"=w1292, "type"=w1293, "diag ref in"=w1298) -> ("error out"=w1296:errorcluster, "success?"=w1295:bool, "diag ref out"=w1297:T18)  [unwired: 5 in]
            }
            frame "KWP-2000" {
              n326 = call <vilib>:"DisableNormalMessageTransmission.vi"("error in (no error)"=w1304, "require response?"=TRUE, "diag ref in"=w1303) -> ("error out"=w1300:errorcluster, "success?"=w1301:bool, "diag ref out"=w1302:T18)  [unwired: 6 in]
            }
          }
          n327 = call "ServiceChannels.Status.Set.vi"("Status Lookup"=w1264, "Type"=Type."Communication Control", "Service Channels Status Ref"=w1263, "error in (no error)"=w1267, "Status"=w1266) -> ("error out"=w1265:errorcluster)  [unwired: 6 in]
          n328 = in-place-cluster #26("Parameters.Service Channels Status Lookup"=w1264, "Service Channels Status"=w1263, "Parameters.CAN.Diagnostic Protocol"=w1276, "ADCS Connection"=w1277) -> (w1258:T1)
        }
      }
      frame "ReturnToNormalMode" {
        n329 = in-place {
          in-place-border: [w1310] -> w1308
          in-place-border: w1307 -> [w1319]
          n330 = in-place-cluster #27(w1306) -> ("Parameters.Service Channels Status Lookup"=w1313:variant, "Service Channels Status"=w1312:T25, "ADCS Connection"=w1318:T18, "Parameters.CAN.Diagnostic Protocol"=w1316:T5)
          n331 = case shown="\"GMLAN\"" w1316 {
            tunnel: [w1322 w1327 w1334 w1336] -> w1314
            tunnel: [w1320 FALSE ("success?") w1333 w1337] -> w1311
            tunnel: w1319 -> [w1324 w1327 w1330 w1340]
            tunnel: w1318 -> [w1323 w1326 w1329 w1339]
            tunnel: [w1321 w1326 w1328 w1338] -> w1317
            frame "GMLAN" {
              n332 = call "GMLAN ReturnToNormalMode.vi"("error in (no error)"=w1324, "diag ref in"=w1323) -> ("error out"=w1322:errorcluster, "success?"=w1320:bool, "diag ref out"=w1321:T18)  [unwired: 7 in]
            }
            frame "User-Defined" {
            }
            frame "UDS" {
              n333 = call <vilib>:"UDS CommunicationControl.vi"("error in (no error)"=w1330, "communication type"=u8 3 ("type"), "type"=u8 0, "diag ref in"=w1329) -> ("error out"=w1334:errorcluster, "success?"=w1333:bool, "diag ref out"=w1328:T18)  [unwired: 5 in]
            }
            frame "KWP-2000" {
              n334 = call <vilib>:"EnableNormalMessageTransmission.vi"("error in (no error)"=w1340, "require response?"=TRUE, "diag ref in"=w1339) -> ("error out"=w1336:errorcluster, "success?"=w1337:bool, "diag ref out"=w1338:T18)  [unwired: 6 in]
            }
          }
          n335 = call "ServiceChannels.Status.Set.vi"("Status Lookup"=w1313, "Type"=Type."Communication Control", "Service Channels Status Ref"=w1312, "error in (no error)"=w1314, "Status"=w1311) -> ("error out"=w1310:errorcluster)  [unwired: 6 in]
          n336 = in-place-cluster #27("Parameters.Service Channels Status Lookup"=w1313, "Service Channels Status"=w1312, "ADCS Connection"=w1317, "Parameters.CAN.Diagnostic Protocol"=w1316) -> (w1305:T1)
        }
      }
      frame "UnlockECU" {
        n337 = in-place {
          in-place-border: w1345 -> [w1348]
          in-place-border: [w1351] -> w1344
          in-place-border: w1341 -> [w1347]
          n338 = in-place-cluster #28(w1343) -> ("Status"=w1357:T25, "Parameters.Service Channels Status Lookup"=w1350:variant, "Service Channels Status"=w1349:T25, "ADCS Connection"=w1359:T18, "Parameters.Security"=w1355:T16, "Parameters.CAN.Diagnostic Protocol"=w1356:T5)
          n339 = case shown="\"GMLAN\"..\"UDS\"" w1356 {
            selector: w1356 -> [_ w1364]
            tunnel: w1348 -> [w1362 w1370]
            tunnel: w1359 -> [w1360 w1369]
            tunnel: w1355 -> [_ w1368]
            tunnel: [w1360 w1367] -> w1358
            tunnel: [w1362 w1366] -> w1353
            tunnel: [FALSE ("success?") w1365] -> w1352
            tunnel: w1347 -> [_ w1363]
            frame "User-Defined" {
            }
            frame "GMLAN".."UDS" {
              n340 = call "ADCS.UnlockECUSecurity.vi"("Diagnostic Protocol"=w1364, "error in (no error)"=w1370, "MasterKey"=w1363, "Security"=w1368, "diag ref in"=w1369) -> ("error out"=w1366:errorcluster, "success?"=w1365:bool, "diag ref out"=w1367:T18)  [unwired: 4 in]
            }
          }
          n341 = call "ServiceChannels.Status.Set.vi"("Status Lookup"=w1350, "Type"=Type."Unlock ECU", "Service Channels Status Ref"=w1349, "error in (no error)"=w1353, "Status"=w1352) -> ("error out"=w1351:errorcluster)  [unwired: 6 in]
          n342 = in-place-cluster #28("Status"=w1357, "Parameters.Service Channels Status Lookup"=w1350, "Service Channels Status"=w1349, "ADCS Connection"=w1358, "Parameters.Security"=w1355, "Parameters.CAN.Diagnostic Protocol"=w1356) -> (w1342:T1)
        }
      }
      frame "ReadDTCs" {
        n343 = in-place {
          in-place-border: [w1402] -> w1380
          in-place-border: w1379 -> [w1401]
          in-place-border: w1378 -> [w1400]
          in-place-border: w1377 -> [w1399]
          in-place-border: w1376 -> [w1398]
          in-place-border: w1371 -> [w1385]
          n344 = in-place-cluster #29(w1375) -> ("Parameters.Service Channels Status Lookup"=w1381:variant, "Service Channels Status"=w1383:T25, "DTC Count"=w1392:T25, "DTCs"=w1391:T25, "Parameters.DTC.Descriptor"=w1394:T14, "ADCS Connection"=w1396:T18, "Parameters.CAN.Diagnostic Protocol"=w1390:T5)
          n345 = in-place-cluster #30(w1374) -> ("Active DTCs"=w1397:T34[])
          n346 = case shown="\"KWP-2000\", \"UDS\"" w1390 {
            selector: w1390 -> [w1416 w1421 w1447]
            tunnel: [w1412 w1419 w1457] -> w1402
            tunnel: w1401 -> [w1406 _ w1438]
            tunnel: w1400 -> [w1413 w1419 w1456]
            tunnel: w1399 -> [_ _ w1455]
            tunnel: w1398 -> [_ _ w1454]
            tunnel: w1397 -> [w1411 w1420 w1451]
            tunnel: w1396 -> [w1410 w1422 w1450]
            tunnel: [w1411 w1420 w1449] -> w1395
            tunnel: w1394 -> [w1409 w1423 w1433]
            tunnel: [w1410 w1422 w1448] -> w1393
            tunnel: w1392 -> [w1407 w1425 w1445]
            tunnel: w1391 -> [w1408 w1424 w1446]
            tunnel: [w1416 w1421 w1447] -> w1389
            tunnel: [w1409 w1423 w1433] -> w1388
            tunnel: [w1408 w1424 w1446] -> w1387
            tunnel: [w1407 w1425 w1445] -> w1386
            tunnel: w1385 -> [w1405 _ w1437]
            tunnel: [w1404 w1418 w1426] -> w1384
            tunnel: w1383 -> [w1404 w1418 w1426]
            tunnel: [w1403 w1417 w1427] -> w1382
            tunnel: w1381 -> [w1403 w1417 w1427]
            frame "GMLAN" {
              n347 = Flatten To String(anything=w1411, error in (no error)=w1413) -> (data string=w1414:string, error out=w1415:errorcluster)  [unwired: 2 in, 1 out]
              n348 = call <vilib>:"Respond to Command.vi"("error in (no error)"=w1415, "message value"=w1414, "ResponseInfo"=w1406, "VeriStand Comm in"=w1405) -> ("error out"=w1412:errorcluster)  [unwired: 5 in, 2 out]
            }
            frame "User-Defined" {
            }
            frame "KWP-2000", "UDS" {
              n349 = Unflatten From String(type=T45 {"Extension"=0, "Mask"=0, "Mode/Status"=0, "Byte Lengths"={"Override"=FALSE, "DTC"=0, "Status"=0, "Failure"=0}}, binary string=w1455, error in (no error)=w1456) -> (value=w1435:T45, error out=w1453:errorcluster)  [unwired: 2 in, 1 out]
              n350 = Unbundle By Name(w1435) -> ("Extension"=w1443:u32, "Mode/Status"=w1442:u32, "Mask"=w1441:u32)
              n351 = Unbundle By Name(w1435) -> ("Byte Lengths"=w1434:T46)
              n352 = call "DTC.Descriptor.Override.vi"("Byte Lengths"=w1434, "Descriptor in"=w1433) -> ("Descriptor out"=w1432:T14)  [unwired: 9 in]
              n353 = case shown="\"UDS\"" w1447 {
                tunnel: w1432 -> [w1467 w1502 _]
                tunnel: w1453 -> [w1462 w1497 w1520]
                tunnel: w1450 -> [w1461 w1496 w1521]
                tunnel: [w1463 w1498 _] -> w1429
                tunnel: [w1466 w1499 w1520] -> w1444
                tunnel: [w1465 w1501 w1521] -> w1448
                tunnel: [w1464 w1500 _] -> w1452
                tunnel: w1443 -> [w1460 w1495 _]
                tunnel: w1441 -> [w1459 w1494 _]
                tunnel: w1442 -> [w1458 w1493 _]
                frame "UDS" {
                  n354 = case shown="8" w1460 {
                    tunnel: w1467 -> [w1471 w1478 w1492]
                    tunnel: w1459 -> [w1469 w1477 w1491]
                    tunnel: [w1475 w1483 w1490] -> w1466
                    tunnel: [w1472 w1480 w1489] -> w1465
                    tunnel: [w1473 w1481 w1488] -> w1464
                    tunnel: [w1474 w1482 w1487] -> w1463
                    tunnel: w1462 -> [w1476 w1484 w1486]
                    tunnel: w1461 -> [w1470 w1479 w1485]
                    tunnel: w1458 -> [w1468 _ _]
                    frame 8 {
                      n355 = call <vilib>:"UDS ReportDTCBySeverityMaskRecord.vi"("DTC descriptor"=w1471, "error in (no error)"=w1476, "status"=w1468, "severity mask"=w1469, "diag ref in"=w1470) -> ("error out"=w1475:errorcluster, "success?"=w1474:bool, "DTCs"=w1473:T59[], "diag ref out"=w1472:T18)  [unwired: 2 in, 1 out]
                    }
                    frame 9 {
                      n356 = call <vilib>:"UDS ReportSeverityInformationOfDTC.vi"("DTC descriptor"=w1478, "error in (no error)"=w1484, "DTC mask record"=w1477, "diag ref in"=w1479) -> ("error out"=w1483:errorcluster, "success?"=w1482:bool, "DTCs"=w1481:T59[], "diag ref out"=w1480:T18)  [unwired: 3 in, 1 out]
                    }
                    frame 2, Default {
                      n357 = call <vilib>:"UDS ReportDTCByStatusMask.vi"("DTC descriptor"=w1492, "error in (no error)"=w1486, "status mask"=w1491, "diag ref in"=w1485) -> ("error out"=w1490:errorcluster, "success?"=w1487:bool, "DTCs"=w1488:T59[], "diag ref out"=w1489:T18)  [unwired: 3 in, 1 out]
                    }
                  }
                }
                frame "KWP-2000" {
                  n358 = case shown="18" w1495 {
                    tunnel: w1494 -> [w1510 w1519]
                    tunnel: w1502 -> [w1509 w1518]
                    tunnel: [w1508 w1517] -> w1501
                    tunnel: [w1507 w1516] -> w1500
                    tunnel: [w1506 w1515] -> w1499
                    tunnel: [w1505 w1514] -> w1498
                    tunnel: w1497 -> [w1504 w1513]
                    tunnel: w1496 -> [w1503 w1512]
                    tunnel: w1493 -> [_ w1511]
                    frame 23, Default {
                      n359 = call <vilib>:"ReadStatusOfDTC.vi"("DTC descriptor"=w1509, "error in (no error)"=w1504, "group of DTC"=w1510, "diag ref in"=w1503) -> ("error out"=w1506:errorcluster, "success?"=w1505:bool, "DTCs"=w1507:T59[], "diag ref out"=w1508:T18)  [unwired: 4 in]
                    }
                    frame 24 {
                      n360 = call <vilib>:"ReadDTCByStatus.vi"("DTC descriptor"=w1518, "error in (no error)"=w1513, "group of DTC"=w1519, "mode"=w1511, "diag ref in"=w1512) -> ("error out"=w1515:errorcluster, "success?"=w1514:bool, "DTCs"=w1516:T59[], "diag ref out"=w1517:T18)  [unwired: 3 in]
                    }
                  }
                }
                frame "GMLAN", "User-Defined" {
                }
              }
              n361 = case shown="No Error" w1444 {
                selector: w1444 -> [w1523 w1541]
                tunnel: w1446 -> [w1525 _]
                tunnel: w1454 -> [w1533 _]
                tunnel: [w1522 w1541] -> w1430
                tunnel: w1445 -> [w1526 _]
                tunnel: w1452 -> [w1532 _]
                tunnel: w1451 -> [w1531 w1540]
                tunnel: [w1530 w1540] -> w1449
                frame No Error {
                  n362 = Get Date/Time In Seconds() -> (seconds since 1Jan1904=w1529:timestamp)
                  n363 = call "DTCs.List.Update.vi"("current time"=w1529, "Previous Changed DTCs"=w1531, "current DTCs"=w1532) -> ("Active DTCs"=w1530:T34[])  [unwired: 8 in]
                  n364 = Replace Array Subset(array=w1533, new element=w1530, index=0) -> (w1535:T34[])
                  n365 = Array Size(array=w1530) -> (size(s)=w1536:i32)
                  n366 = for {
                    tunnel: w1535 -> [w1539] mode=indexing
                    tunnel: [w1538] -> w1528 mode=concatenating
                    # "Put 10 newest DTCs in VS"
                    n367 = Cluster To Array(cluster=w1539) -> (array=w1538:dbl[])
                  }
                  n368 = To Double Precision Float(number=w1536) -> (double precision float=w1537:dbl)
                  n369 = Build Array(w1537) -> (w1527:dbl[])
                  n370 = call-poly <vilib>:"Data.Processes.Execute.vi"("error in (no error)"=w1523, "Values"=w1527, "Ref"=w1526) -> ("error out"=w1524:errorcluster)  [unwired: 8 in]
                  n371 = call-poly <vilib>:"Data.Processes.Execute.vi"("error in (no error)"=w1524, "Values"=w1528, "Ref"=w1525) -> ("error out"=w1522:errorcluster)  [unwired: 8 in]
                }
                frame Error {
                }
              }
              n372 = call "ServiceChannels.Status.Set.vi"("Status Lookup"=w1427, "Type"=Type."Read DTCs", "Service Channels Status Ref"=w1426, "error in (no error)"=w1430, "Status"=w1429) -> ("error out"=w1428:errorcluster)  [unwired: 6 in]
              n373 = Flatten To String(anything=w1449, error in (no error)=w1428) -> (data string=w1439:string, error out=w1440:errorcluster)  [unwired: 2 in, 1 out]
              n374 = call <vilib>:"Respond to Command.vi"("error in (no error)"=w1440, "message value"=w1439, "ResponseInfo"=w1438, "VeriStand Comm in"=w1437) -> ("error out"=w1457:errorcluster)  [unwired: 5 in, 2 out]
            }
          }
          n375 = in-place-cluster #29("Parameters.Service Channels Status Lookup"=w1382, "Service Channels Status"=w1384, "DTC Count"=w1386, "DTCs"=w1387, "Parameters.DTC.Descriptor"=w1388, "ADCS Connection"=w1393, "Parameters.CAN.Diagnostic Protocol"=w1389) -> (w1372:T1)
          n376 = in-place-cluster #30("Active DTCs"=w1395) -> (w1373:T35)
        }
      }
      frame "ClearDTCs" {
        n377 = in-place {
          in-place-border: w1554 -> [w1582]
          in-place-border: w1553 -> [w1581]
          in-place-border: [w1558] -> w1552
          in-place-border: w1551 -> [w1580]
          in-place-border: w1550 -> [w1579]
          in-place-border: w1543 -> [w1565]
          in-place-border: w1542 -> [w1563]
          n378 = in-place-cluster #31(w1549) -> ("Parameters.Service Channels Status Lookup"=w1560:variant, "Service Channels Status"=w1561:T25, "Status"=w1567:T25, "DTC Count"=w1574:T25, "DTCs"=w1575:T25, "Parameters.DTC.Descriptor"=w1576:T14, "Parameters.CAN.Diagnostic Protocol"=w1571:T5, "ADCS Connection"=w1578:T18, "XNETEngine (GMLAN)"=w1569:T24)
          n379 = case shown="\"User-Defined\"" w1571 {
            selector: w1571 -> [w1599 w1609 w1627]
            tunnel: w1582 -> [w1588 _ w1622]
            tunnel: w1581 -> [_ _ _]
            tunnel: [w1593 FALSE ("success?") w1639] -> w1555
            tunnel: [w1585 w1606 w1636] -> w1562
            tunnel: w1580 -> [_ _ w1635]
            tunnel: w1579 -> [w1598 w1606 w1634]
            tunnel: w1578 -> [w1596 w1608 w1631]
            tunnel: [w1595 w1608 w1630] -> w1577
            tunnel: w1576 -> [w1590 w1604 w1616]
            tunnel: w1575 -> [w1601 w1610 w1628]
            tunnel: w1574 -> [w1600 w1611 w1629]
            tunnel: [w1600 w1611 w1629] -> w1573
            tunnel: [w1601 w1610 w1628] -> w1572
            tunnel: [w1599 w1609 w1627] -> w1570
            tunnel: w1569 -> [w1592 w1607 w1626]
            tunnel: [w1592 w1607 w1626] -> w1568
            tunnel: [w1591 w1612 w1625] -> w1566
            tunnel: w1567 -> [w1591 w1612 w1625]
            tunnel: w1565 -> [_ _ w1624]
            tunnel: [w1590 w1604 w1616] -> w1564
            tunnel: w1563 -> [w1587 _ w1621]
            tunnel: w1561 -> [w1584 w1603 w1613]
            tunnel: w1560 -> [w1583 w1602 w1614]
            tunnel: [w1583 w1602 w1614] -> w1557
            tunnel: [w1584 w1603 w1613] -> w1556
            frame "GMLAN" {
              n380 = call <vilib>:"Send Local Message.vi"("message queue in"=w1592, "message name"="ClearDTCs" ("Message Name"), "error in"=w1598) -> ("error out"=w1597:errorcluster)  [unwired: 10 in, 2 out]
              n381 = call "GMLAN ClearDiagnosticInformation.vi"("error in (no error)"=w1597, "diag ref in"=w1596) -> ("error out"=w1586:errorcluster, "success?"=w1593:bool, "diag ref out"=w1595:T18)  [unwired: 7 in]
              n382 = call <vilib>:"Respond to Command.vi"("error in (no error)"=w1586, "message value"="Cleared" ("Message Value"), "ResponseInfo"=w1588, "VeriStand Comm in"=w1587) -> ("error out"=w1585:errorcluster)  [unwired: 5 in, 2 out]
            }
            frame "User-Defined" {
            }
            frame "KWP-2000", "UDS" {
              (unwired) u32 16777215 items=["All"=16777215] ("Group of DTC")
              n383 = Unflatten From String(type=T47 {"Group of DTC"=16777215, "Byte Lengths"={"Override"=FALSE, "DTC"=0, "Status"=0, "Failure"=0}} ("Clear DTC Settings"), binary string=w1635, error in (no error)=w1634) -> (value=w1632:T47, error out=w1633:errorcluster)  [unwired: 2 in, 1 out]
              n384 = Unbundle By Name(w1632) -> ("Byte Lengths"=w1617:T46, "Group of DTC"=w1618:u32)
              n385 = call "DTC.Descriptor.Override.vi"("Byte Lengths"=w1617, "Descriptor in"=w1616) -> ("Descriptor out"=w1615:T14)  [unwired: 9 in]
              n386 = case shown="\"KWP-2000\"" w1627 {
                tunnel: w1631 -> [w1642 w1647 w1656]
                tunnel: [w1642 w1646 w1655] -> w1630
                tunnel: [w1641 w1644 w1654] -> w1620
                tunnel: [FALSE ("success?") w1645 w1653] -> w1639
                tunnel: w1615 -> [_ w1643 w1652]
                tunnel: w1633 -> [w1641 w1649 w1651]
                tunnel: w1618 -> [_ w1648 w1650]
                frame "GMLAN", "User-Defined" {
                }
                frame "KWP-2000" {
                  n387 = call <vilib>:"ClearDiagnosticInformation.vi"("DTC descriptor"=w1643, "error in (no error)"=w1649, "group of DTC"=w1648, "diag ref in"=w1647) -> ("error out"=w1644:errorcluster, "success?"=w1645:bool, "diag ref out"=w1646:T18)  [unwired: 5 in]
                }
                frame "UDS" {
                  n388 = call <vilib>:"UDS ClearDiagnosticInformation.vi"("DTC descriptor"=w1652, "error in (no error)"=w1651, "group of DTC"=w1650, "diag ref in"=w1656) -> ("error out"=w1654:errorcluster, "success?"=w1653:bool, "diag ref out"=w1655:T18)  [unwired: 5 in]
                }
              }
              n389 = call-poly <vilib>:"Data.Processes.Execute.vi"("error in (no error)"=w1620, "Values"=w1624, "Ref"=w1628) -> ("error out"=w1637:errorcluster)  [unwired: 8 in]
              n390 = call <vilib>:"Respond to Command.vi"("error in (no error)"=w1620, "message value"="Cleared" ("Message Value"), "ResponseInfo"=w1622, "VeriStand Comm in"=w1621) -> ()  [unwired: 5 in, 3 out]
              n391 = call-poly <vilib>:"Data.Processes.Execute.vi"("error in (no error)"=w1637, "Values"=dbl[] [0.0] ("element"), "Ref"=w1629) -> ("error out"=w1636:errorcluster)  [unwired: 8 in]
            }
          }
          n392 = call "ServiceChannels.Status.Set.vi"("Status Lookup"=w1557, "Type"=Type."Clear DTCs", "Service Channels Status Ref"=w1556, "error in (no error)"=w1562, "Status"=w1555) -> ("error out"=w1558:errorcluster)  [unwired: 6 in]
          n393 = in-place-cluster #31("Parameters.Service Channels Status Lookup"=w1557, "Service Channels Status"=w1556, "Status"=w1566, "DTC Count"=w1573, "DTCs"=w1572, "Parameters.DTC.Descriptor"=w1564, "Parameters.CAN.Diagnostic Protocol"=w1570, "ADCS Connection"=w1577, "XNETEngine (GMLAN)"=w1568) -> (w1548:T1)
        }
        n394 = Bundle By Name(cluster=w1547, "Active DTCs"=T34[] [], "status mask"=u8 0) -> (w1544:T35)
      }
      frame "PollDIDs" {
        n395 = in-place {
          in-place-border: w1664 -> [w1683]
          in-place-border: [w1671] -> w1663
          in-place-border: w1660 -> [w1681]
          in-place-border: w1659 -> [w1680]
          n396 = in-place-cluster #32(w1657) -> ("Polling.Queued"=w1677:bool[])
          n397 = in-place-cluster #33(w1662) -> ("Status"=w1685:T25, "Parameters.Service Channels Status Lookup"=w1672:variant, "Service Channels Status"=w1673:T25, "Reads"=w1668:T25, "ADCS Connection"=w1688:T18, "Parameters.Frames Lookup"=w1689:variant, "Parameters.CAN.Diagnostic Protocol"=w1686:T5)
          n398 = Unflatten From String(type=u32 0 ("ID"), binary string=w1681, error in (no error)=w1683) -> (value=w1676:u32, error out=w1682:errorcluster)  [unwired: 2 in, 1 out]
          n399 = Replace Array Subset(array=w1677, new element=FALSE ("new element/subarray"), index=w1676) -> (w1674:bool[])
          n400 = Index Array(array=w1680, index=w1676) -> (element=w1679:T15)
          n401 = Unbundle By Name(w1679) -> ("DID IDs"=w1678:u32[])
          n402 = for {
            shift-right: [w1715] -> w1687
            shift-left: w1688 -> [w1716]
            tunnel: w1689 -> [w1705]
            tunnel: w1678 -> [w1703] mode=indexing
            tunnel: w1686 -> [w1717]
            tunnel: w1668 -> [w1704]
            tunnel: w1673 -> [w1706]
            tunnel: w1672 -> [w1707]
            tunnel: w1682 -> [w1718]
            shift-right: [w1700] -> w1666
            shift-left: errorcluster {"status"=FALSE, "code"=0, "source"=""} ("error IO") -> [w1699]
            stop <- w1709 stop-if-true
            w1711 = TRUE ("Buffer?")
            w1712 = Type."DID" ("Type")
            n403 = case shown="\"UDS\"" w1717 {
              tunnel: w1718 -> [w1722 w1730 w1735 w1742]
              tunnel: w1716 -> [w1724 w1732 w1734 w1741]
              tunnel: [w1720 w1729 w1735 w1740] -> w1714
              tunnel: [w1725 w1728 FALSE ("success?") w1739] -> w1708
              tunnel: [w1719 w1727 _ w1738] -> w1702
              tunnel: w1703 -> [w1721 w1731 _ w1737]
              tunnel: [w1723 w1726 w1734 w1736] -> w1715
              frame "GMLAN", Default {
                n404 = call "GMLAN ReadDataByIdentifier.vi"("error in (no error)"=w1722, "Data ID (DID)"=w1721, "diag ref in"=w1724) -> ("error out"=w1720:errorcluster, "success?"=w1725:bool, "data out"=w1719:u8[], "diag ref out"=w1723:T18)  [unwired: 5 in]
              }
              frame "KWP-2000" {
                n405 = call <vilib>:"ReadDataByLocalIdentifier.vi"("error in (no error)"=w1730, "local ID"=w1731, "diag ref in"=w1732) -> ("error out"=w1729:errorcluster, "success?"=w1728:bool, "data out"=w1727:u8[], "diag ref out"=w1726:T18)  [unwired: 5 in]
              }
              frame "User-Defined" {
              }
              frame "UDS" {
                n406 = call <vilib>:"UDS ReadDataByIdentifier.vi"("error in (no error)"=w1742, "ID"=w1737, "diag ref in"=w1741) -> ("error out"=w1740:errorcluster, "success?"=w1739:bool, "data out"=w1738:u8[], "diag ref out"=w1736:T18)  [unwired: 5 in]
              }
            }
            n407 = call "Signals.Scale.EU.vi"("Buffer?"=w1711, "Lookup"=w1705, "Type"=w1712, "Reads Ref"=w1704, "error in (no error)"=w1714, "Unscaled Data"=w1702, "ID"=w1703) -> ("error out"=w1713:errorcluster)  [unwired: 4 in]
            n408 = call "ServiceChannels.Status.Set.vi"("Buffer?"=w1711, "Status Lookup"=w1707, "Type"=w1712, "Service Channels Status Ref"=w1706, "error in (no error)"=w1713, "Status"=w1708, "ID"=w1703) -> ("error out"=w1710:errorcluster)  [unwired: 4 in]
            n409 = call "Diagnostics.CheckTimeout.vi"("error in (no error)"=w1710) -> ("error out"=w1701:errorcluster, "Timeout"=w1709:bool)  [unwired: 9 in]
            n410 = Merge Errors(w1699, w1701) -> (w1700:errorcluster)
          }
          n411 = flat-sequence {
            tunnel: w1666 -> [w1692]
            tunnel: w1673 -> [w1693]
            tunnel: [w1693] -> w1670
            tunnel: [w1692] -> w1669
            tunnel: w1668 -> [w1691]
            tunnel: [w1690] -> w1667
            tunnel: [w1695] -> w1671
            tunnel: w1670 -> [w1698]
            tunnel: w1669 -> [w1697]
            tunnel: w1667 -> [w1694]
            frame #0 {
              n412 = call-poly <vilib>:"Data.Processes.Execute.vi"("Ref"=w1691) -> ("error out"=w1690:errorcluster)  [unwired: 10 in]
            }
            frame #1 {
              n413 = call-poly <vilib>:"Data.Processes.Execute.vi"("Ref"=w1698) -> ("error out"=w1696:errorcluster)  [unwired: 10 in]
              n414 = Merge Errors(w1697, w1694, w1696) -> (w1695:errorcluster)
            }
          }
          n415 = in-place-cluster #33("Status"=w1685, "Parameters.Service Channels Status Lookup"=w1672, "Service Channels Status"=w1673, "Reads"=w1668, "ADCS Connection"=w1687, "Parameters.Frames Lookup"=w1689, "Parameters.CAN.Diagnostic Protocol"=w1686) -> (w1661:T1)
          n416 = in-place-cluster #32("Polling.Queued"=w1674) -> (w1658:T35)
        }
      }
      frame "ReadDIDs" {
        n417 = in-place {
          in-place-border: w1747 -> [w1766]
          in-place-border: [w1756] -> w1746
          in-place-border: w1743 -> [w1760]
          n418 = in-place-cluster #34(w1745) -> ("Status"=w1748:T25, "Service Channels Status"=w1749:T25, "Parameters.Service Channels Status Lookup"=w1757:variant, "Reads"=w1752:T25, "ADCS Connection"=w1763:T18, "Parameters.Frames Lookup"=w1764:variant, "Parameters.CAN.Diagnostic Protocol"=w1761:T5)
          n419 = Unbundle By Name(w1760) -> ("DID IDs"=w1765:u32[])
          n420 = for {
            shift-right: [w1791] -> w1762
            shift-left: w1763 -> [w1792]
            tunnel: w1764 -> [w1781]
            tunnel: w1765 -> [w1779] mode=indexing
            tunnel: [w1777] -> w1767 mode=indexing
            tunnel: w1761 -> [w1793]
            tunnel: w1752 -> [w1780]
            tunnel: w1749 -> [w1782]
            tunnel: w1757 -> [w1783]
            tunnel: w1766 -> [w1794]
            tunnel: [w1785] -> w1759 mode=indexing
            stop <- w1784 stop-if-true
            w1787 = TRUE ("Buffer?")
            w1789 = Type."DID" ("Type")
            n421 = case shown="\"UDS\"" w1793 {
              tunnel: w1794 -> [w1798 w1806 w1811 w1818]
              tunnel: w1792 -> [w1800 w1808 w1810 w1817]
              tunnel: [w1796 w1805 w1811 w1816] -> w1790
              tunnel: [w1801 w1804 FALSE ("success?") w1815] -> w1777
              tunnel: [w1795 w1803 _ w1814] -> w1778
              tunnel: w1779 -> [w1797 w1807 _ w1813]
              tunnel: [w1799 w1802 w1810 w1812] -> w1791
              frame "GMLAN", Default {
                n422 = call "GMLAN ReadDataByIdentifier.vi"("error in (no error)"=w1798, "Data ID (DID)"=w1797, "diag ref in"=w1800) -> ("error out"=w1796:errorcluster, "success?"=w1801:bool, "data out"=w1795:u8[], "diag ref out"=w1799:T18)  [unwired: 5 in]
              }
              frame "KWP-2000" {
                n423 = call <vilib>:"ReadDataByLocalIdentifier.vi"("error in (no error)"=w1806, "local ID"=w1807, "diag ref in"=w1808) -> ("error out"=w1805:errorcluster, "success?"=w1804:bool, "data out"=w1803:u8[], "diag ref out"=w1802:T18)  [unwired: 5 in]
              }
              frame "User-Defined" {
              }
              frame "UDS" {
                n424 = call <vilib>:"UDS ReadDataByIdentifier.vi"("error in (no error)"=w1818, "ID"=w1813, "diag ref in"=w1817) -> ("error out"=w1816:errorcluster, "success?"=w1815:bool, "data out"=w1814:u8[], "diag ref out"=w1812:T18)  [unwired: 5 in]
              }
            }
            n425 = call "Signals.Scale.EU.vi"("Buffer?"=w1787, "Lookup"=w1781, "Type"=w1789, "Reads Ref"=w1780, "error in (no error)"=w1790, "Unscaled Data"=w1778, "ID"=w1779) -> ("error out"=w1788:errorcluster)  [unwired: 4 in]
            n426 = call "ServiceChannels.Status.Set.vi"("Buffer?"=w1787, "Status Lookup"=w1783, "Type"=w1789, "Service Channels Status Ref"=w1782, "error in (no error)"=w1788, "Status"=w1777, "ID"=w1779) -> ("error out"=w1786:errorcluster)  [unwired: 4 in]
            n427 = call "Diagnostics.CheckTimeout.vi"("error in (no error)"=w1786) -> ("error out"=w1785:errorcluster, "Timeout"=w1784:bool)  [unwired: 9 in]
          }
          n428 = And Array Elements(Boolean array=w1767) -> (logical AND=w1758:bool)
          n429 = Merge Errors(w1759) -> (w1755:errorcluster)
          n430 = call "Status.Set.vi"("Status Ref"=w1748, "error in (no error)"=w1755, "Status"=w1758) -> ("error out"=w1750:errorcluster)  [unwired: 8 in]
          n431 = flat-sequence {
            tunnel: w1750 -> [w1770]
            tunnel: w1749 -> [w1771]
            tunnel: [w1771] -> w1754
            tunnel: [w1770] -> w1753
            tunnel: w1752 -> [w1769]
            tunnel: [w1768] -> w1751
            tunnel: [w1773] -> w1756
            tunnel: w1754 -> [w1776]
            tunnel: w1753 -> [w1775]
            tunnel: w1751 -> [w1772]
            frame #0 {
              n432 = call-poly <vilib>:"Data.Processes.Execute.vi"("Ref"=w1769) -> ("error out"=w1768:errorcluster)  [unwired: 10 in]
            }
            frame #1 {
              n433 = call-poly <vilib>:"Data.Processes.Execute.vi"("Ref"=w1776) -> ("error out"=w1774:errorcluster)  [unwired: 10 in]
              n434 = Merge Errors(w1775, w1772, w1774) -> (w1773:errorcluster)
            }
          }
          n435 = in-place-cluster #34("Status"=w1748, "Service Channels Status"=w1749, "Parameters.Service Channels Status Lookup"=w1757, "Reads"=w1752, "ADCS Connection"=w1762, "Parameters.Frames Lookup"=w1764, "Parameters.CAN.Diagnostic Protocol"=w1761) -> (w1744:T1)
        }
      }
      frame "ReadDID" {
        n436 = in-place {
          in-place-border: w1826 -> [w1852]
          in-place-border: w1825 -> [w1851]
          in-place-border: w1827 -> [_]
          in-place-border: [w1844] -> w1824
          in-place-border: w1820 -> [w1843]
          in-place-border: w1819 -> [w1842]
          w1836 = Type."DID" ("Type")
          n437 = in-place-cluster #35(w1823) -> ("Status"=w1847:T25, "Parameters.Service Channels Status Lookup"=w1833:variant, "Service Channels Status"=w1832:T25, "Reads"=w1830:T25, "ADCS Connection"=w1850:T18, "Parameters.Frames Lookup"=w1831:variant, "Parameters.CAN.Diagnostic Protocol"=w1848:T5)
          n438 = Unflatten From String(type=u16 0 ("ID"), binary string=w1851, error in (no error)=w1852) -> (value=w1829:u16, error out=w1853:errorcluster)  [unwired: 2 in, 1 out]
          n439 = case shown="\"User-Defined\"" w1848 {
            tunnel: w1853 -> [w1857 w1865 w1870 w1877]
            tunnel: w1850 -> [w1859 w1867 w1869 w1876]
            tunnel: [w1855 w1864 w1870 w1875] -> w1845
            tunnel: [w1860 w1863 FALSE ("success?") w1874] -> w1834
            tunnel: [w1854 w1862 _ w1873] -> w1828
            tunnel: w1829 -> [w1856 w1866 _ w1872]
            tunnel: [w1858 w1861 w1869 w1871] -> w1849
            frame "GMLAN", Default {
              n440 = call "GMLAN ReadDataByIdentifier.vi"("error in (no error)"=w1857, "Data ID (DID)"=w1856, "diag ref in"=w1859) -> ("error out"=w1855:errorcluster, "success?"=w1860:bool, "data out"=w1854:u8[], "diag ref out"=w1858:T18)  [unwired: 5 in]
            }
            frame "KWP-2000" {
              n441 = call <vilib>:"ReadDataByLocalIdentifier.vi"("error in (no error)"=w1865, "local ID"=w1866, "diag ref in"=w1867) -> ("error out"=w1864:errorcluster, "success?"=w1863:bool, "data out"=w1862:u8[], "diag ref out"=w1861:T18)  [unwired: 5 in]
            }
            frame "User-Defined" {
            }
            frame "UDS" {
              n442 = call <vilib>:"UDS ReadDataByIdentifier.vi"("error in (no error)"=w1877, "ID"=w1872, "diag ref in"=w1876) -> ("error out"=w1875:errorcluster, "success?"=w1874:bool, "data out"=w1873:u8[], "diag ref out"=w1871:T18)  [unwired: 5 in]
            }
          }
          n443 = call "Signals.Scale.EU.vi"("Lookup"=w1831, "Type"=w1836, "Reads Ref"=w1830, "error in (no error)"=w1845, "Unscaled Data"=w1828, "ID"=w1829) -> ("error out"=w1838:errorcluster)  [unwired: 5 in]
          n444 = call "ServiceChannels.Status.Set.vi"("Status Lookup"=w1833, "Type"=w1836, "Service Channels Status Ref"=w1832, "error in (no error)"=w1838, "Status"=w1834, "ID"=w1829) -> ("error out"=w1837:errorcluster)  [unwired: 5 in]
          n445 = Bundle By Name(cluster=T48 {"ID"=0, "Raw Frame"=[], "error out"={"status"=FALSE, "code"=0, "source"=""}}, "ID"=w1829, "Raw Frame"=w1828) -> (w1840:T48)
          n446 = Flatten To String(anything=w1840, error in (no error)=w1837) -> (data string=w1839:string, error out=w1835:errorcluster)  [unwired: 2 in, 1 out]
          n447 = in-place-cluster #35("Status"=w1847, "Parameters.Service Channels Status Lookup"=w1833, "Service Channels Status"=w1832, "Reads"=w1830, "ADCS Connection"=w1849, "Parameters.Frames Lookup"=w1831, "Parameters.CAN.Diagnostic Protocol"=w1848) -> (w1822:T1)
          n448 = call <vilib>:"Respond to Command.vi"("error in (no error)"=w1835, "message value"=w1839, "ResponseInfo"=w1843, "VeriStand Comm in"=w1842) -> ("error out"=w1844:errorcluster)  [unwired: 5 in, 2 out]
        }
      }
      frame "GenerateCDID" {
        n449 = in-place {
          in-place-border: w1882 -> [w1901]
          in-place-border: w1881 -> [w1900]
          in-place-border: [w1891] -> w1880
          w1892 = Type."CDID" ("Type")
          n450 = in-place-cluster #36(w1879) -> ("Parameters.Service Channels Status Lookup"=w1889:variant, "Service Channels Status"=w1888:T25, "ADCS Connection"=w1899:T18, "Parameters.CAN.Diagnostic Protocol"=w1897:T5, "Parameters.Frames Lookup"=w1887:variant, "Writes"=w1886:T26)
          n451 = Unflatten From String(type=u16 0, binary string=w1900, error in (no error)=w1901) -> (value=w1885:u16, error out=w1894:errorcluster)  [unwired: 2 in, 1 out]
          n452 = call "Signals.Scale.Raw.vi"("Lookup"=w1887, "Type"=w1892, "Writes Ref"=w1886, "error in"=w1894, "ID"=w1885) -> ("error out"=w1895:errorcluster, "Data"=w1884:u8[])  [unwired: 5 in]
          n453 = case shown="\"UDS\"" w1897 {
            tunnel: w1885 -> [w1907 w1909 _ w1919]
            tunnel: w1884 -> [w1905 w1910 _ w1920]
            tunnel: [w1904 w1912 w1917 w1925] -> w1893
            tunnel: [w1903 w1911 FALSE ("success?") w1924] -> w1890
            tunnel: w1895 -> [w1908 w1913 w1917 w1923]
            tunnel: w1899 -> [w1906 w1915 w1918 w1922]
            tunnel: [w1902 w1914 w1918 w1921] -> w1898
            frame "KWP-2000" {
              n454 = call <vilib>:"WriteDataByLocalIdentifier.vi"("data in"=w1905, "error in (no error)"=w1908, "local ID"=w1907, "diag ref in"=w1906) -> ("error out"=w1904:errorcluster, "success?"=w1903:bool, "diag ref out"=w1902:T18)  [unwired: 5 in]
            }
            frame "GMLAN" {
              n455 = call "GMLAN WriteDataByIdentifier.vi"("error in (no error)"=w1913, "data"=w1910, "Data ID (DID)"=w1909, "diag ref in"=w1915) -> ("error out"=w1912:errorcluster, "success?"=w1911:bool, "diag ref out"=w1914:T18)  [unwired: 5 in]
            }
            frame "User-Defined" {
            }
            frame "UDS" {
              n456 = call <vilib>:"UDS WriteDataByIdentifier.vi"("data in"=w1920, "error in (no error)"=w1923, "ID"=w1919, "diag ref in"=w1922) -> ("error out"=w1925:errorcluster, "success?"=w1924:bool, "diag ref out"=w1921:T18)  [unwired: 5 in]
            }
          }
          n457 = call "ServiceChannels.Status.Set.vi"("Status Lookup"=w1889, "Type"=w1892, "Service Channels Status Ref"=w1888, "error in (no error)"=w1893, "Status"=w1890, "ID"=w1885) -> ("error out"=w1891:errorcluster)  [unwired: 5 in]
          n458 = in-place-cluster #36("Parameters.Service Channels Status Lookup"=w1889, "Service Channels Status"=w1888, "ADCS Connection"=w1898, "Parameters.CAN.Diagnostic Protocol"=w1897, "Parameters.Frames Lookup"=w1887, "Writes"=w1886) -> (w1878:T1)
        }
      }
      frame "ChannelPassThru" {
        # "NOT CURRENTLY SUPPORTED"
        n459 = in-place {
          in-place-border: w1932 -> [_]
          in-place-border: [w1934] -> w1931
          in-place-border: w1930 -> [_]
          in-place-border: w1929 -> [w1954]
          in-place-border: w1928 -> [w1953]
          n460 = in-place-cluster #37(w1927) -> ("ADCS Connection"=w1951:T18)
          n461 = Unflatten From String(type=T49 {"Service"=0, "Service Length"=0, "Data Length"=0, "Response Required"=FALSE}, binary string=w1954, error in (no error)=w1953) -> (value=w1952:T49, error out=w1937:errorcluster)  [unwired: 2 in, 1 out]
          n462 = Unbundle By Name(w1952) -> ("Response Required"=w1938:bool, "Service"=w1947:u64, "Service Length"=w1944:u8, "Data Length"=w1943:u32)
          n463 = Type Cast(type=u8[] [], x=w1947) -> (*(type *) &x=w1945:u8[])
          n464 = Subtract(x=u8 8 ("y"), y=w1944) -> (x-y=w1935:u8)
          n465 = Array Subset(array=w1945, index=w1935) -> (w1941:u8[])  [unwired: 1 in]
          n466 = Initialize Array(u8 0, w1943) -> (w1940:u8[])
          n467 = Build Array (concatenate)(w1941, w1940) -> (w1939:u8[])
          n468 = call <vilib>:"Diagnostic Service.vi"("error source"="Diagnostic Service.vi", "error in (no error)"=w1937, "data in"=w1939, "require response?"=w1938, "diag ref in"=w1951) -> ("error out"=w1934:errorcluster, "diag ref out"=w1950:T18)  [unwired: 1 in, 4 out]
          n469 = in-place-cluster #37("ADCS Connection"=w1950) -> (w1926:T1)
        }
      }
      frame "UserDefinedMessage" {
        n470 = in-place {
          in-place-border: w1959 -> [w1985]
          in-place-border: [w1969] -> w1955
          in-place-border: w1958 -> [w1984]
          w1970 = Type."User Defined" ("Type")
          n471 = in-place-cluster #38(w1957) -> ("Parameters.Service Channels Status Lookup"=w1967:variant, "Service Channels Status"=w1966:T25, "Parameters.Frames Lookup"=w1964:variant, "Reads"=w1965:T25, "ADCS Connection"=w1982:T18, "Writes"=w1963:T26)
          n472 = Unflatten From String(type=u32 0 ("ID"), binary string=w1984, error in (no error)=w1985) -> (value=w1962:u32, error out=w1972:errorcluster)  [unwired: 2 in, 1 out]
          n473 = call "Signals.Scale.Raw.vi"("Lookup"=w1964, "Type"=w1970, "Writes Ref"=w1963, "error in"=w1972, "ID"=w1962) -> ("error out"=w1978:errorcluster, "Data"=w1981:u8[])  [unwired: 5 in]
          n474 = call "Frames.Lookup.Size.Get.vi"("Type"=w1970, "error in (no error)"=w1978, "ID"=w1962, "Frames Lookup"=w1964) -> ("error out"=w1977:errorcluster, "ByteLength"=w1973:u16)  [unwired: 5 in, 1 out]
          n475 = Not Equal To 0?(x=w1973) -> (x != 0?=w1976:bool)
          n476 = disable-structure shown="Default" {
            disable-tunnel: w1982 -> [w1994 w1998]
            disable-tunnel: w1981 -> [w1993 w1996]
            disable-tunnel: [w1992 w2002] -> w1974
            disable-tunnel: [w1991 w1999] -> w1980
            disable-tunnel: [w1990 w2001] -> w1961
            disable-tunnel: [w1989 w2000] -> w1979
            disable-tunnel: w1977 -> [w1988 w2003]
            disable-tunnel: w1976 -> [w1987 w1997]
            disable-tunnel: "Diagnostic Service.vi" ("error source") -> [w1986 w1995]
            frame condition #0 (active) {
              n477 = call <vilib>:"Diagnostic Service.vi"("error source"=w1986, "error in (no error)"=w1988, "data in"=w1993, "require response?"=w1987, "diag ref in"=w1994) -> ("error out"=w1992:errorcluster, "data out"=w1990:u8[], "error code"=w1989:u8, "diag ref out"=w1991:T18)  [unwired: 1 in, 2 out]
            }
            frame condition #1 {
              n478 = call "CustomerSpecific_SendReceive.vi"("error source"=w1995, "error in (no error)"=w2003, "data in"=w1996, "require response?"=w1997, "diag ref in"=w1998) -> ("error out"=w2002:errorcluster, "data out"=w2001:u8[], "error code"=w2000:u8, "diag ref out"=w1999:T18)  [unwired: 3 in]
            }
          }
          n479 = Equal To 0?(x=w1979) -> (x = 0?=w1968:bool)
          n480 = call "Signals.Scale.EU.vi"("Lookup"=w1964, "Type"=w1970, "Reads Ref"=w1965, "error in (no error)"=w1974, "Unscaled Data"=w1961, "ID"=w1962) -> ("error out"=w1971:errorcluster)  [unwired: 5 in]
          n481 = call "ServiceChannels.Status.Set.vi"("Status Lookup"=w1967, "Type"=w1970, "Service Channels Status Ref"=w1966, "error in (no error)"=w1971, "Status"=w1968, "ID"=w1962) -> ("error out"=w1969:errorcluster)  [unwired: 5 in]
          n482 = in-place-cluster #38("Parameters.Service Channels Status Lookup"=w1967, "Service Channels Status"=w1966, "Parameters.Frames Lookup"=w1964, "Reads"=w1965, "ADCS Connection"=w1980, "Writes"=w1963) -> (w1956:T1)
        }
      }
      frame "<--------------- TCP ONLY --------------->" {
      }
      frame "PassThru" {
        n483 = in-place {
          in-place-border: w2013 -> [w2016]
          in-place-border: [w2034] -> w2012
          in-place-border: w2011 -> [w2029]
          in-place-border: w2010 -> [w2028]
          in-place-border: w2007 -> [w2015]
          n484 = in-place-cluster #39(w2009) -> ("ADCS Connection"=w2025:T18)
          n485 = Unflatten From String(type=cluster{"cmd":u8[], "require response?":bool} {"cmd"=[], "require response?"=TRUE}, binary string=w2029, error in (no error)=w2028) -> (value=w2026:cluster{"cmd":u8[], "require response?":bool}, error out=w2022:errorcluster)  [unwired: 2 in, 1 out]
          n486 = Unbundle By Name(w2026) -> ("require response?"=w2024:bool, "cmd"=w2023:u8[])
          n487 = disable-structure shown="Default" {
            disable-tunnel: w2025 -> [w2043 w2047]
            disable-tunnel: w2023 -> [w2042 w2045]
            disable-tunnel: [w2041 w2051] -> w2021
            disable-tunnel: [w2040 w2048] -> w2018
            disable-tunnel: [w2039 w2050] -> w2020
            disable-tunnel: [w2038 w2049] -> w2019
            disable-tunnel: w2022 -> [w2037 w2052]
            disable-tunnel: w2024 -> [w2036 w2046]
            disable-tunnel: "Diagnostic Service.vi" ("error source") -> [w2035 w2044]
            frame condition #0 (active) {
              n488 = call <vilib>:"Diagnostic Service.vi"("error source"=w2035, "error in (no error)"=w2037, "data in"=w2042, "require response?"=w2036, "diag ref in"=w2043) -> ("error out"=w2041:errorcluster, "data out"=w2039:u8[], "error code"=w2038:u8, "diag ref out"=w2040:T18)  [unwired: 1 in, 2 out]
            }
            frame condition #1 {
              n489 = call "CustomerSpecific_SendReceive.vi"("error source"=w2044, "error in (no error)"=w2052, "data in"=w2045, "require response?"=w2046, "diag ref in"=w2047) -> ("error out"=w2051:errorcluster, "data out"=w2050:u8[], "error code"=w2049:u8, "diag ref out"=w2048:T18)  [unwired: 3 in]
            }
          }
          n490 = Bundle By Name(cluster=T50 {"resp"=[], "error code"=0, "error out"={"status"=FALSE, "code"=0, "source"=""}}, "error code"=w2019, "resp"=w2020, "error out"=w2021) -> (w2031:T50)
          n491 = Flatten To String(anything=w2031, error in (no error)=w2022) -> (data string=w2030:string, error out=w2032:errorcluster)  [unwired: 2 in, 1 out]
          n492 = in-place-cluster #39("ADCS Connection"=w2018) -> (w2008:T1)
          n493 = call <vilib>:"Respond to Command.vi"("error in (no error)"=w2032, "message value"=w2030, "ResponseInfo"=w2016, "VeriStand Comm in"=w2015) -> ("error out"=w2034:errorcluster)  [unwired: 5 in, 2 out]
        }
      }
      frame "<--------------- UDS/KWP ONLY --------------->" {
      }
      frame "ControlDTC" {
        n494 = in-place {
          in-place-border: w2058 -> [w2081]
          in-place-border: [w2068] -> w2057
          in-place-border: w2056 -> [w2080]
          w2070 = Type."DTC Control" ("Type")
          n495 = in-place-cluster #40(w2060) -> ("Parameters.DTC.Descriptor"=w2073:T14, "Parameters.Frames Lookup"=w2065:variant, "Parameters.Service Channels Status Lookup"=w2067:variant, "Service Channels Status"=w2066:T25, "ADCS Connection"=w2083:T18, "Parameters.CAN.Diagnostic Protocol"=w2084:T5, "Writes"=w2064:T26)
          n496 = Unflatten From String(type=T51 {"Group/Type"=16777215, "Byte Lengths (KWP only)"={"Override"=FALSE, "DTC"=0, "Status"=0, "Failure"=0}} ("Clear DTC Settings"), binary string=w2080, error in (no error)=w2081) -> (value=w2079:T51, error out=w2077:errorcluster)  [unwired: 2 in, 1 out]
          n497 = Unbundle By Name(w2079) -> ("Byte Lengths (KWP only)"=w2074:T46, "Group/Type"=w2075:u32)
          n498 = call "DTC.Descriptor.Override.vi"("Byte Lengths"=w2074, "Descriptor in"=w2073) -> ("Descriptor out"=w2072:T14)  [unwired: 9 in]
          n499 = call "Signals.Scale.Raw.vi"("Lookup"=w2065, "Type"=w2070, "Writes Ref"=w2064, "error in"=w2077, "ID"=u32 0) -> ("error out"=w2078:errorcluster, "Data"=w2063:u8[])  [unwired: 5 in]
          n500 = case shown="\"GMLAN\", \"User-Defined\"" w2084 {
            tunnel: w2078 -> [w2087 w2094 w2102]
            tunnel: [w2087 w2093 w2101] -> w2071
            tunnel: w2072 -> [_ _ w2100]
            tunnel: w2083 -> [w2086 w2091 w2099]
            tunnel: [w2086 w2092 w2098] -> w2082
            tunnel: [FALSE ("success?") w2090 w2097] -> w2069
            tunnel: w2075 -> [_ w2089 w2096]
            tunnel: w2063 -> [_ w2088 w2095]
            frame "GMLAN", "User-Defined" {
            }
            frame "UDS" {
              n501 = call <vilib>:"UDS ControlDTCSetting.vi"("error in (no error)"=w2094, "type"=w2089, "data in"=w2088, "diag ref in"=w2091) -> ("error out"=w2093:errorcluster, "success?"=w2090:bool, "diag ref out"=w2092:T18)  [unwired: 5 in]
            }
            frame "KWP-2000" {
              n502 = call <vilib>:"ControlDTCSetting.vi"("DTC descriptor"=w2100, "error in (no error)"=w2102, "group of DTC"=w2096, "data in"=w2095, "diag ref in"=w2099) -> ("error out"=w2101:errorcluster, "success?"=w2097:bool, "diag ref out"=w2098:T18)  [unwired: 4 in]
            }
          }
          n503 = call "ServiceChannels.Status.Set.vi"("Status Lookup"=w2067, "Type"=w2070, "Service Channels Status Ref"=w2066, "error in (no error)"=w2071, "Status"=w2069) -> ("error out"=w2068:errorcluster)  [unwired: 6 in]
          n504 = in-place-cluster #40("Parameters.DTC.Descriptor"=w2073, "Parameters.Frames Lookup"=w2065, "Parameters.Service Channels Status Lookup"=w2067, "Service Channels Status"=w2066, "ADCS Connection"=w2082, "Parameters.CAN.Diagnostic Protocol"=w2084, "Writes"=w2064) -> (w2059:T1)
        }
      }
      frame "ECUReset" {
        n505 = in-place {
          in-place-border: w2107 -> [w2119]
          in-place-border: [w2111] -> w2106
          in-place-border: w2105 -> [w2118]
          n506 = in-place-cluster #41(w2104) -> ("Parameters.Service Channels Status Lookup"=w2110:variant, "Service Channels Status"=w2109:T25, "Parameters.CAN.Diagnostic Protocol"=w2115:T5, "ADCS Connection"=w2117:T18)
          n507 = Unflatten From String(type=u8 0 ("ID"), binary string=w2118, error in (no error)=w2119) -> (value=w2122:u8, error out=w2121:errorcluster)  [unwired: 2 in, 1 out]
          n508 = case shown="\"GMLAN\", \"User-Defined\"" w2115 {
            tunnel: [FALSE ("success?") w2129 w2137] -> w2112
            tunnel: [w2124 w2130 w2136] -> w2114
            tunnel: w2122 -> [_ w2126 w2135]
            tunnel: w2121 -> [w2124 w2131 w2134]
            tunnel: w2117 -> [w2125 w2127 w2133]
            tunnel: [w2125 w2128 w2132] -> w2116
            frame "GMLAN", "User-Defined" {
            }
            frame "KWP-2000" {
              n509 = call <vilib>:"ECUReset.vi"("error in (no error)"=w2131, "mode"=w2126, "diag ref in"=w2127) -> ("error out"=w2130:errorcluster, "success?"=w2129:bool, "diag ref out"=w2128:T18)  [unwired: 6 in]
            }
            frame "UDS" {
              n510 = call <vilib>:"UDS ECUReset.vi"("error in (no error)"=w2134, "mode"=w2135, "diag ref in"=w2133) -> ("error out"=w2136:errorcluster, "success?"=w2137:bool, "diag ref out"=w2132:T18)  [unwired: 5 in, 1 out]
            }
          }
          n511 = call "ServiceChannels.Status.Set.vi"("Status Lookup"=w2110, "Type"=Type."Reset ECU", "Service Channels Status Ref"=w2109, "error in (no error)"=w2114, "Status"=w2112) -> ("error out"=w2111:errorcluster)  [unwired: 6 in]
          n512 = in-place-cluster #41("Parameters.Service Channels Status Lookup"=w2110, "Service Channels Status"=w2109, "Parameters.CAN.Diagnostic Protocol"=w2115, "ADCS Connection"=w2116) -> (w2103:T1)
        }
      }
      frame "ReadMemory" {
        n513 = in-place {
          in-place-border: w2142 -> [w2159]
          in-place-border: [w2151] -> w2141
          in-place-border: w2140 -> [w2158]
          w2152 = Type."Read Memory" ("Type")
          n514 = in-place-cluster #42(w2139) -> ("Parameters.CAN.Diagnostic Protocol"=w2161:T5, "Parameters.Service Channels Status Lookup"=w2150:variant, "Service Channels Status"=w2149:T25, "Parameters.Frames Lookup"=w2148:variant, "Reads"=w2147:T25, "ADCS Connection"=w2162:T18)
          n515 = Unflatten From String(type=T52 {"Address"=0, "Service Type"=0, "Address Length"=0, "Size Length"=0}, binary string=w2158, error in (no error)=w2159) -> (value=w2156:T52, error out=w2155:errorcluster)  [unwired: 2 in, 1 out]
          n516 = case shown="\"UDS\"" w2161 {
            tunnel: [w2171 w2187 w2209] -> w2157
            tunnel: [w2173 w2188 w2208] -> w2160
            tunnel: w2155 -> [w2168 w2177 w2209]
            tunnel: w2162 -> [w2174 w2189 w2208]
            tunnel: [w2170 w2186 _] -> w2144
            tunnel: w2156 -> [w2169 w2184 _]
            tunnel: [w2172 w2185 _] -> w2145
            tunnel: w2148 -> [w2166 w2180 _]
            tunnel: [w2165 w2175 _] -> w2146
            frame "KWP-2000" {
              n517 = Unbundle By Name(w2169) -> ("Address"=w2165:u64)
              n518 = call "Frames.Lookup.Size.Get.vi"("Type"=Type."Read Memory", "error in (no error)"=w2168, "ID"=w2165, "Frames Lookup"=w2166) -> ("error out"=w2167:errorcluster, "ByteLength"=w2164:u16)  [unwired: 5 in, 1 out]
              n519 = call <vilib>:"ReadMemoryByAddress.vi"("error in (no error)"=w2167, "size"=w2164, "address"=w2165, "diag ref in"=w2174) -> ("error out"=w2171:errorcluster, "success?"=w2170:bool, "data out"=w2172:u8[], "diag ref out"=w2173:T18)  [unwired: 4 in]
            }
            frame "UDS" {
              n520 = Unbundle By Name(w2184) -> ("Service Type"=w2183:u32, "Address"=w2175:u64, "Address Length"=w2182:u8, "Size Length"=w2181:u8)
              n521 = call "Frames.Lookup.Size.Get.vi"("Type"=Type."Read Memory", "error in (no error)"=w2177, "ID"=w2175, "Frames Lookup"=w2180) -> ("error out"=w2176:errorcluster, "ByteLength"=w2178:u16)  [unwired: 5 in, 1 out]
              n522 = case shown="2" w2183 {
                tunnel: w2189 -> [w2199 w2207]
                tunnel: [w2195 w2206] -> w2188
                tunnel: w2176 -> [w2198 w2205]
                tunnel: [w2197 w2204] -> w2187
                tunnel: [w2194 w2203] -> w2186
                tunnel: [w2196 w2202] -> w2185
                tunnel: w2175 -> [w2191 w2201]
                tunnel: w2182 -> [w2193 _]
                tunnel: w2181 -> [w2192 _]
                tunnel: w2178 -> [w2190 w2200]
                frame 2 {
                  n523 = call <vilib>:"UDS06 ReadMemoryByAddress.vi"("memory size length"=w2192, "memory address length"=w2193, "error in (no error)"=w2198, "memory size"=w2190, "memory address"=w2191, "diag ref in"=w2199) -> ("error out"=w2197:errorcluster, "success?"=w2194:bool, "data out"=w2196:u8[], "diag ref out"=w2195:T18)  [unwired: 2 in]
                }
                frame 1, Default {
                  n524 = call <vilib>:"UDS ReadMemoryByAddress.vi"("error in (no error)"=w2205, "size"=w2200, "address"=w2201, "diag ref in"=w2207) -> ("error out"=w2204:errorcluster, "success?"=w2203:bool, "data out"=w2202:u8[], "diag ref out"=w2206:T18)  [unwired: 4 in]
                }
              }
            }
            frame "GMLAN", "User-Defined" {
            }
          }
          n525 = call "Signals.Scale.EU.vi"("Lookup"=w2148, "Type"=w2152, "Reads Ref"=w2147, "error in (no error)"=w2157, "Unscaled Data"=w2145, "ID"=w2146) -> ("error out"=w2153:errorcluster)  [unwired: 5 in]
          n526 = call "ServiceChannels.Status.Set.vi"("Status Lookup"=w2150, "Type"=w2152, "Service Channels Status Ref"=w2149, "error in (no error)"=w2153, "Status"=w2144, "ID"=w2146) -> ("error out"=w2151:errorcluster)  [unwired: 5 in]
          n527 = in-place-cluster #42("Parameters.CAN.Diagnostic Protocol"=w2161, "Parameters.Service Channels Status Lookup"=w2150, "Service Channels Status"=w2149, "Parameters.Frames Lookup"=w2148, "Reads"=w2147, "ADCS Connection"=w2160) -> (w2138:T1)
        }
      }
      frame "WriteMemory" {
        n528 = in-place {
          in-place-border: w2214 -> [w2234]
          in-place-border: [w2222] -> w2213
          in-place-border: w2212 -> [w2233]
          w2223 = Type."Write Memory" ("Type")
          n529 = in-place-cluster #43(w2211) -> ("Parameters.CAN.Diagnostic Protocol"=w2236:T5, "Parameters.Service Channels Status Lookup"=w2220:variant, "Service Channels Status"=w2219:T25, "ADCS Connection"=w2237:T18, "Parameters.Frames Lookup"=w2218:variant, "Writes"=w2217:T26)
          n530 = Unflatten From String(type=T52 {"Address"=0, "Service Type"=0, "Address Length"=0, "Size Length"=0}, binary string=w2233, error in (no error)=w2234) -> (value=w2230:T52, error out=w2225:errorcluster)  [unwired: 2 in, 1 out]
          n531 = Unbundle By Name(w2230) -> ("Address"=w2216:u64, "Service Type"=w2228:u32, "Address Length"=w2227:u8, "Size Length"=w2226:u8)
          n532 = call "Signals.Scale.Raw.vi"("Lookup"=w2218, "Type"=w2223, "Writes Ref"=w2217, "error in"=w2225, "ID"=w2216) -> ("error out"=w2232:errorcluster, "Data"=w2231:u8[])  [unwired: 5 in]
          n533 = case shown="\"GMLAN\", \"User-Defined\"" w2236 {
            tunnel: [w2243 w2255 w2276] -> w2224
            tunnel: [w2241 w2253 w2275] -> w2235
            tunnel: w2232 -> [w2244 w2256 w2276]
            tunnel: w2237 -> [w2245 w2252 w2275]
            tunnel: [w2242 w2254 _] -> w2221
            tunnel: w2216 -> [w2240 w2248 _]
            tunnel: w2231 -> [w2238 w2247 _]
            tunnel: w2228 -> [_ w2251 _]
            tunnel: w2218 -> [_ _ _]
            tunnel: w2227 -> [_ w2250 _]
            tunnel: w2226 -> [_ w2249 _]
            frame "KWP-2000" {
              n534 = Array Size(array=w2238) -> (size(s)=w2239:i32)
              n535 = call <vilib>:"WriteMemoryByAddress.vi"("data in"=w2238, "error in (no error)"=w2244, "size"=w2239, "address"=w2240, "diag ref in"=w2245) -> ("error out"=w2243:errorcluster, "success?"=w2242:bool, "diag ref out"=w2241:T18)  [unwired: 4 in]
            }
            frame "UDS" {
              n536 = Array Size(array=w2247) -> (size(s)=w2246:i32)
              n537 = case shown="2" w2251 {
                tunnel: w2256 -> [w2265 w2274]
                tunnel: [w2263 w2273] -> w2255
                tunnel: [w2262 w2272] -> w2254
                tunnel: [w2264 w2271] -> w2253
                tunnel: w2248 -> [w2261 w2270]
                tunnel: w2252 -> [w2266 w2269]
                tunnel: w2247 -> [w2257 w2267]
                tunnel: w2250 -> [w2260 _]
                tunnel: w2249 -> [w2259 _]
                tunnel: w2246 -> [w2258 w2268]
                frame 2 {
                  n538 = call <vilib>:"UDS06 WriteMemoryByAddress.vi"("memory size length"=w2259, "memory address length"=w2260, "data in"=w2257, "error in (no error)"=w2265, "memory size"=w2258, "memory address"=w2261, "diag ref in"=w2266) -> ("error out"=w2263:errorcluster, "success?"=w2262:bool, "diag ref out"=w2264:T18)  [unwired: 2 in]
                }
                frame 1, Default {
                  n539 = call <vilib>:"UDS WriteMemoryByAddress.vi"("data in"=w2267, "error in (no error)"=w2274, "size"=w2268, "address"=w2270, "diag ref in"=w2269) -> ("error out"=w2273:errorcluster, "success?"=w2272:bool, "diag ref out"=w2271:T18)  [unwired: 4 in]
                }
              }
            }
            frame "GMLAN", "User-Defined" {
            }
          }
          n540 = call "ServiceChannels.Status.Set.vi"("Status Lookup"=w2220, "Type"=w2223, "Service Channels Status Ref"=w2219, "error in (no error)"=w2224, "Status"=w2221, "ID"=w2216) -> ("error out"=w2222:errorcluster)  [unwired: 5 in]
          n541 = in-place-cluster #43("Parameters.CAN.Diagnostic Protocol"=w2236, "Parameters.Service Channels Status Lookup"=w2220, "Service Channels Status"=w2219, "ADCS Connection"=w2235, "Parameters.Frames Lookup"=w2218, "Writes"=w2217) -> (w2210:T1)
        }
      }
      frame "InputOutputControl" {
        n542 = in-place {
          in-place-border: w2281 -> [w2302]
          in-place-border: [w2291] -> w2279
          in-place-border: w2280 -> [w2301]
          w2293 = Type."IO Control" ("Type")
          n543 = in-place-cluster #44(w2278) -> ("Parameters.CAN.Diagnostic Protocol"=w2304:T5, "Parameters.Service Channels Status Lookup"=w2290:variant, "Service Channels Status"=w2289:T25, "Parameters.Frames Lookup"=w2287:variant, "Reads"=w2288:T25, "ADCS Connection"=w2305:T18, "Writes"=w2286:T26)
          n544 = Unflatten From String(type=T53 {"ID"=0, "Mode"=0}, binary string=w2301, error in (no error)=w2302) -> (value=w2297:T53, error out=w2295:errorcluster)  [unwired: 2 in, 1 out]
          n545 = Unbundle By Name(w2297) -> ("ID"=w2285:u16, "Mode"=w2296:u8)
          n546 = call "Signals.Scale.Raw.vi"("Lookup"=w2287, "Type"=w2293, "Writes Ref"=w2286, "error in"=w2295, "ID"=w2285) -> ("error out"=w2300:errorcluster, "Data"=w2283:u8[])  [unwired: 5 in]
          n547 = case shown="\"UDS\"" w2304 {
            tunnel: [w2314 w2339 w2359] -> w2299
            tunnel: [w2313 w2335 w2358] -> w2303
            tunnel: w2300 -> [w2311 w2340 w2359]
            tunnel: w2305 -> [w2312 w2337 w2358]
            tunnel: [w2310 w2333 _] -> w2292
            tunnel: w2285 -> [w2309 w2338 _]
            tunnel: w2283 -> [w2308 w2336 _]
            tunnel: [w2307 w2334 _] -> w2284
            tunnel: w2296 -> [w2306 w2332 _]
            frame "KWP-2000" {
              n548 = case shown="0" w2306 {
                selector: w2306 -> [w2315 w2324]
                tunnel: [w2323 w2331] -> w2314
                tunnel: [w2322 w2330] -> w2313
                tunnel: w2312 -> [w2321 w2329]
                tunnel: w2311 -> [w2320 w2328]
                tunnel: [w2319 w2327] -> w2310
                tunnel: w2309 -> [w2318 w2326]
                tunnel: w2308 -> [w2317 _]
                tunnel: [w2316 w2325] -> w2307
                frame Default {
                  n549 = call <vilib>:"InputOutputControlByLocalIdentifier.vi"("data in"=w2317, "error in (no error)"=w2320, "mode"=w2315, "local ID"=w2318, "diag ref in"=w2321) -> ("error out"=w2323:errorcluster, "success?"=w2319:bool, "data out"=w2316:u8[], "diag ref out"=w2322:T18)  [unwired: 3 in]
                }
                frame 0 {
                  n550 = call <vilib>:"InputOutputControlByLocalIdentifier.vi"("error in (no error)"=w2328, "mode"=w2324, "local ID"=w2326, "diag ref in"=w2329) -> ("error out"=w2331:errorcluster, "success?"=w2327:bool, "data out"=w2325:u8[], "diag ref out"=w2330:T18)  [unwired: 4 in]
                }
              }
            }
            frame "UDS" {
              n551 = case shown="Default" w2332 {
                selector: w2332 -> [w2341 w2349]
                tunnel: w2340 -> [w2346 w2357]
                tunnel: [w2345 w2356] -> w2339
                tunnel: w2338 -> [w2347 w2355]
                tunnel: w2337 -> [w2348 w2354]
                tunnel: w2336 -> [_ w2353]
                tunnel: [w2342 w2352] -> w2335
                tunnel: [w2343 w2351] -> w2334
                tunnel: [w2344 w2350] -> w2333
                frame 0 {
                  n552 = call <vilib>:"UDS InputOutputControlByIdentifier.vi"("error in (no error)"=w2346, "mode"=w2341, "ID"=w2347, "diag ref in"=w2348) -> ("error out"=w2345:errorcluster, "success?"=w2344:bool, "data out"=w2343:u8[], "diag ref out"=w2342:T18)  [unwired: 4 in]
                }
                frame Default {
                  n553 = call <vilib>:"UDS InputOutputControlByIdentifier.vi"("data in"=w2353, "error in (no error)"=w2357, "mode"=w2349, "ID"=w2355, "diag ref in"=w2354) -> ("error out"=w2356:errorcluster, "success?"=w2350:bool, "data out"=w2351:u8[], "diag ref out"=w2352:T18)  [unwired: 3 in]
                }
              }
            }
            frame "GMLAN", "User-Defined" {
            }
          }
          n554 = call "Signals.Scale.EU.vi"("Lookup"=w2287, "Type"=w2293, "Reads Ref"=w2288, "error in (no error)"=w2299, "Unscaled Data"=w2284, "ID"=w2285) -> ("error out"=w2294:errorcluster)  [unwired: 5 in]
          n555 = call "ServiceChannels.Status.Set.vi"("Status Lookup"=w2290, "Type"=w2293, "Service Channels Status Ref"=w2289, "error in (no error)"=w2294, "Status"=w2292, "ID"=w2285) -> ("error out"=w2291:errorcluster)  [unwired: 5 in]
          n556 = in-place-cluster #44("Parameters.CAN.Diagnostic Protocol"=w2304, "Parameters.Service Channels Status Lookup"=w2290, "Service Channels Status"=w2289, "Parameters.Frames Lookup"=w2287, "Reads"=w2288, "ADCS Connection"=w2303, "Writes"=w2286) -> (w2277:T1)
        }
      }
      frame "StartRoutine" {
        n557 = in-place {
          in-place-border: w2364 -> [w2383]
          in-place-border: [w2374] -> w2363
          in-place-border: w2360 -> [w2381]
          w2375 = Type."Routine Start" ("Type")
          n558 = in-place-cluster #45(w2362) -> ("Parameters.Service Channels Status Lookup"=w2373:variant, "Service Channels Status"=w2372:T25, "Parameters.CAN.Diagnostic Protocol"=w2385:T5, "Parameters.Frames Lookup"=w2368:variant, "Reads"=w2371:T25, "ADCS Connection"=w2386:T18, "Writes"=w2367:T26)
          n559 = Unflatten From String(type=u16 0, binary string=w2381, error in (no error)=w2383) -> (value=w2366:u16, error out=w2377:errorcluster)  [unwired: 2 in, 1 out]
          n560 = call "Signals.Scale.Raw.vi"("Lookup"=w2368, "Type"=w2375, "Writes Ref"=w2367, "error in"=w2377, "ID"=w2366) -> ("error out"=w2380:errorcluster, "Data"=w2379:u8[])  [unwired: 5 in]
          n561 = case shown="\"GMLAN\", \"User-Defined\"" w2385 {
            tunnel: [w2394 w2403 w2405] -> w2378
            tunnel: [w2393 w2401 w2404] -> w2384
            tunnel: w2380 -> [w2391 w2400 w2405]
            tunnel: w2386 -> [w2392 w2399 w2404]
            tunnel: [w2390 w2398 _] -> w2369
            tunnel: w2366 -> [w2389 w2397 _]
            tunnel: w2379 -> [w2388 w2396 _]
            tunnel: [w2387 w2395 _] -> w2370
            frame "KWP-2000" {
              n562 = call <vilib>:"StartRoutineByLocalIdentifier.vi"("error in (no error)"=w2391, "data in"=w2388, "local ID"=w2389, "diag ref in"=w2392) -> ("error out"=w2394:errorcluster, "success?"=w2390:bool, "data out"=w2387:u8[], "diag ref out"=w2393:T18)  [unwired: 4 in]
            }
            frame "UDS" {
              w2402 = u8 1 items=["Start routine"=1, "Stop routine"=2, "Request routine results"=3] ("mode")
              n563 = call <vilib>:"UDS RoutineControl.vi"("mode"=w2402, "error in (no error)"=w2400, "data in"=w2396, "ID"=w2397, "diag ref in"=w2399) -> ("error out"=w2403:errorcluster, "success?"=w2398:bool, "data out"=w2395:u8[], "diag ref out"=w2401:T18)  [unwired: 3 in]
            }
            frame "GMLAN", "User-Defined" {
            }
          }
          n564 = call "Signals.Scale.EU.vi"("Lookup"=w2368, "Type"=w2375, "Reads Ref"=w2371, "error in (no error)"=w2378, "Unscaled Data"=w2370, "ID"=w2366) -> ("error out"=w2376:errorcluster)  [unwired: 5 in]
          n565 = call "ServiceChannels.Status.Set.vi"("Status Lookup"=w2373, "Type"=w2375, "Service Channels Status Ref"=w2372, "error in (no error)"=w2376, "Status"=w2369, "ID"=w2366) -> ("error out"=w2374:errorcluster)  [unwired: 5 in]
          n566 = in-place-cluster #45("Parameters.Service Channels Status Lookup"=w2373, "Service Channels Status"=w2372, "Parameters.CAN.Diagnostic Protocol"=w2385, "Parameters.Frames Lookup"=w2368, "Reads"=w2371, "ADCS Connection"=w2384, "Writes"=w2367) -> (w2361:T1)
        }
      }
      frame "RequestRoutineStatus" {
        n567 = in-place {
          in-place-border: w2410 -> [w2430]
          in-place-border: [w2419] -> w2408
          in-place-border: w2409 -> [w2428]
          w2421 = Type."Routine Request" ("Type")
          n568 = in-place-cluster #46(w2407) -> ("Status"=w2424:T25, "Parameters.Service Channels Status Lookup"=w2417:variant, "Service Channels Status"=w2420:T25, "Parameters.CAN.Diagnostic Protocol"=w2432:T5, "Parameters.Frames Lookup"=w2414:variant, "Reads"=w2415:T25, "ADCS Connection"=w2433:T18, "Writes"=w2416:T26)
          n569 = Unflatten From String(type=u16 0, binary string=w2428, error in (no error)=w2430) -> (value=w2413:u16, error out=w2423:errorcluster)  [unwired: 2 in, 1 out]
          n570 = call "Signals.Scale.Raw.vi"("Lookup"=w2414, "Type"=w2421, "Writes Ref"=w2416, "error in"=w2423, "ID"=w2413) -> ("error out"=w2427:errorcluster, "Data"=w2426:u8[])  [unwired: 5 in]
          n571 = case shown="\"GMLAN\", \"User-Defined\"" w2432 {
            tunnel: [w2437 w2449 w2451] -> w2425
            tunnel: [w2434 w2447 w2450] -> w2431
            tunnel: w2427 -> [w2439 w2446 w2451]
            tunnel: w2433 -> [w2438 w2445 w2450]
            tunnel: [w2436 w2444 _] -> w2418
            tunnel: w2413 -> [w2440 w2443 _]
            tunnel: w2426 -> [_ w2442 _]
            tunnel: [w2435 w2441 _] -> w2412
            frame "KWP-2000" {
              n572 = call <vilib>:"RequestRoutineResultsByLocalIdentifier.vi"("error in (no error)"=w2439, "local ID"=w2440, "diag ref in"=w2438) -> ("error out"=w2437:errorcluster, "success?"=w2436:bool, "data out"=w2435:u8[], "diag ref out"=w2434:T18)  [unwired: 5 in]
            }
            frame "UDS" {
              w2448 = u8 3 items=["Start routine"=1, "Stop routine"=2, "Request routine results"=3] ("mode")
              n573 = call <vilib>:"UDS RoutineControl.vi"("mode"=w2448, "error in (no error)"=w2446, "data in"=w2442, "ID"=w2443, "diag ref in"=w2445) -> ("error out"=w2449:errorcluster, "success?"=w2444:bool, "data out"=w2441:u8[], "diag ref out"=w2447:T18)  [unwired: 3 in]
            }
            frame "GMLAN", "User-Defined" {
            }
          }
          n574 = call "Signals.Scale.EU.vi"("Lookup"=w2414, "Type"=w2421, "Reads Ref"=w2415, "error in (no error)"=w2425, "Unscaled Data"=w2412, "ID"=w2413) -> ("error out"=w2422:errorcluster)  [unwired: 5 in]
          n575 = call "ServiceChannels.Status.Set.vi"("Status Lookup"=w2417, "Type"=w2421, "Service Channels Status Ref"=w2420, "error in (no error)"=w2422, "Status"=w2418, "ID"=w2413) -> ("error out"=w2419:errorcluster)  [unwired: 5 in]
          n576 = in-place-cluster #46("Status"=w2424, "Parameters.Service Channels Status Lookup"=w2417, "Service Channels Status"=w2420, "Parameters.CAN.Diagnostic Protocol"=w2432, "Parameters.Frames Lookup"=w2414, "Reads"=w2415, "ADCS Connection"=w2431, "Writes"=w2416) -> (w2406:T1)
        }
      }
      frame "StopRoutine" {
        n577 = in-place {
          in-place-border: w2455 -> [w2476]
          in-place-border: [w2461] -> w2452
          in-place-border: w2454 -> [w2474]
          w2467 = Type."Routine Stop" ("Type")
          n578 = in-place-cluster #47(w2456) -> ("Status"=w2470:T25, "Parameters.Service Channels Status Lookup"=w2463:variant, "Service Channels Status"=w2462:T25, "Parameters.CAN.Diagnostic Protocol"=w2478:T5, "Parameters.Frames Lookup"=w2465:variant, "Reads"=w2464:T25, "ADCS Connection"=w2479:T18, "Writes"=w2466:T26)
          n579 = Unflatten From String(type=u16 0, binary string=w2474, error in (no error)=w2476) -> (value=w2459:u16, error out=w2469:errorcluster)  [unwired: 2 in, 1 out]
          n580 = call "Signals.Scale.Raw.vi"("Lookup"=w2465, "Type"=w2467, "Writes Ref"=w2466, "error in"=w2469, "ID"=w2459) -> ("error out"=w2473:errorcluster, "Data"=w2472:u8[])  [unwired: 5 in]
          n581 = case shown="\"GMLAN\", \"User-Defined\"" w2478 {
            tunnel: [w2483 w2496 w2498] -> w2471
            tunnel: [w2486 w2494 w2497] -> w2477
            tunnel: w2473 -> [w2482 w2493 w2498]
            tunnel: w2479 -> [w2487 w2492 w2497]
            tunnel: [w2484 w2491 _] -> w2460
            tunnel: w2459 -> [w2481 w2490 _]
            tunnel: w2472 -> [w2480 w2489 _]
            tunnel: [w2485 w2488 _] -> w2458
            frame "KWP-2000" {
              n582 = call <vilib>:"StopRoutineByLocalIdentifier.vi"("error in (no error)"=w2482, "data in"=w2480, "local ID"=w2481, "diag ref in"=w2487) -> ("error out"=w2483:errorcluster, "success?"=w2484:bool, "data out"=w2485:u8[], "diag ref out"=w2486:T18)  [unwired: 4 in]
            }
            frame "UDS" {
              w2495 = u8 2 items=["Start routine"=1, "Stop routine"=2, "Request routine results"=3] ("mode")
              n583 = call <vilib>:"UDS RoutineControl.vi"("mode"=w2495, "error in (no error)"=w2493, "data in"=w2489, "ID"=w2490, "diag ref in"=w2492) -> ("error out"=w2496:errorcluster, "success?"=w2491:bool, "data out"=w2488:u8[], "diag ref out"=w2494:T18)  [unwired: 3 in]
            }
            frame "GMLAN", "User-Defined" {
            }
          }
          n584 = call "Signals.Scale.EU.vi"("Lookup"=w2465, "Type"=w2467, "Reads Ref"=w2464, "error in (no error)"=w2471, "Unscaled Data"=w2458, "ID"=w2459) -> ("error out"=w2468:errorcluster)  [unwired: 5 in]
          n585 = call "ServiceChannels.Status.Set.vi"("Status Lookup"=w2463, "Type"=w2467, "Service Channels Status Ref"=w2462, "error in (no error)"=w2468, "Status"=w2460, "ID"=w2459) -> ("error out"=w2461:errorcluster)  [unwired: 5 in]
          n586 = in-place-cluster #47("Status"=w2470, "Parameters.Service Channels Status Lookup"=w2463, "Service Channels Status"=w2462, "Parameters.CAN.Diagnostic Protocol"=w2478, "Parameters.Frames Lookup"=w2465, "Reads"=w2464, "ADCS Connection"=w2477, "Writes"=w2466) -> (w2453:T1)
        }
      }
    }
    n587 = disable-structure shown="DebugRT==TRUE" {
      disable-tunnel: w70 -> [w82 w88]
      disable-tunnel: [w82 w88] -> w48
      frame condition #0 {
        n588 = case shown="Default" w82 {
          selector: w82 -> [_ w86]
          tunnel: [_ w83] -> _
          frame "" {
          }
          frame Default {
            w85 = 2 items=["Error", "Warning", "Informational"] ("severity")
            n589 = Concatenate Strings(w86, " Started..." ("string")) -> (w84:string)
            n590 = call <vilib>:"Write to System Log.vi"("severity"=w85, "message"=w84) -> ("error out"=w83:errorcluster)  [unwired: 9 in]
          }
        }
      }
      frame condition #1 (active) {
      }
    }
    n591 = Unbundle By Name(w61) -> ("TesterPresentEnabled?"=w60:bool)
    n592 = call "ADCS.TesterPresent.vi"("Enabled?"=w60, "error in (no error)"=w63, "Reset"=w62, "State Variables in"=w66) -> ("error out"=w55:errorcluster, "State Variables out"=w65:T1)  [unwired: 6 in]
    n593 = call "Restart.LocalStop.Read.vi"("error in (no error)"=w55, "Data Value Reference in"=w51) -> ("error out"=w47:errorcluster, "LocalStop"=w53:bool)  [unwired: 8 in]
    n594 = disable-structure shown="DebugRT==TRUE" {
      disable-tunnel: w48 -> [w76 _]
      disable-tunnel: w47 -> [_ _]
      frame condition #0 {
        n595 = case shown="Default" w76 {
          selector: w76 -> [_ w80]
          tunnel: [_ w77] -> _
          frame "" {
          }
          frame Default {
            w79 = 2 items=["Error", "Warning", "Informational"] ("severity")
            n596 = Concatenate Strings(w80, " Finished..." ("string")) -> (w78:string)
            n597 = call <vilib>:"Write to System Log.vi"("severity"=w79, "message"=w78) -> ("error out"=w77:errorcluster)  [unwired: 9 in]
          }
        }
      }
      frame condition #1 (active) {
      }
    }
    n598 = call <vilib>:"Async.Processes.Report.vi"("Error"=w47, "Stop Async on Error?"=FALSE ("Stop on Error?"), "Process in"=w59) -> ("Stop"=w54:bool)  [unwired: 7 in, 1 out]
    n599 = Compound Arithmetic op=OR(w53, w54) -> (w52:bool)
  }
  "error out" <- w31
